vi "fast scanner v2.1.vi"() -> ()   [LabVIEW 2015]
uses:
  libs/Controls/outofrange.ctl
  libs/Controls/loopclock.ctl
  libs/Controls/fast scanner.ctl
  libs/Controls/String.ctl
  libs/Controls/Number.ctl
  <vilib>/Analysis/Matrix/Datatypes/RealMatrix.ctl
  <vilib>/userdefined/High Color/IMAQdx.ctl
  <vilib>/Analysis/6fits.llb/Curve Fitting Criteria.ctl
  <vilib>/Utility/miscctls.llb/LVFormatAndPrecisionTypeDef.ctl
  <vilib>/Utility/file.llb/Write Delimited Spreadsheet (string).vi
  <vilib>/Utility/file.llb/Read Delimited Spreadsheet (string).vi
  <vilib>/Utility/file.llb/Write Delimited Spreadsheet (I64).vi
  <vilib>/Utility/file.llb/Write Delimited Spreadsheet (DBL).vi
  Zaber A Series/Zaber A Series.lvlib
  libs/Proximity_sensor/MEDAQLib/MEDAQLib.lvlib
  <vilib>/Analysis/Matrix/NI_Matrix.lvlib
  <vilib>/Analysis/NI_AALPro.lvlib
panel:
  in  "Pause button 2":refnum<vi>
  in  "Acceleration\n [mm/s^2] 2":dbl=10.0 min=1.0 max=488.0 step=1.0
  in  "Speed Z [mm/s] 2":dbl(slide) caption="Z Speed\n[mm/s]" min=0.5 max=10.0 step=0.5 scale=0.5..10.0
  out "Measurement On!":bool
  out "Program Closed":bool
  out "Proximity on":bool
  out "Shutter Open":bool
  in  "Data folder path":path=path "D:/Users/XRF/Desktop/Dante_acquire6/Scan Data"
  out "DANTE loaded":bool
  out "IP added":bool
  out "Library Initialized":bool
  out "DANTE configured":bool
  out "Enum":T1=enum."MoveToStartPoint"
  out "scan mode":bool
  out "Port":refnum<visa-resource-name>
  out "MotorsReady":bool
  out "Speed 2":T2 scale=0.0..30.0
  in  "Tab Control":T3(tab)
  in  "Connect/Disconnect Prox":bool
  out "Proximity distance":dbl
  in  "Home":bool
  in  "StopMotion":bool
  in  "GoToZ":bool
  in  "GoToY":bool
  in  "GoToX":bool
  in  "GoTo Z [mm]":dbl format="%#.8g"
  in  "GoTo Y [mm]":dbl format="%#.8g"
  in  "GoTo X [mm]":dbl format="%#.8g"
  in  "Reduced Speed":bool
  in  "Speed Z [mm/s]":dbl(slide)=1.0 caption="Z Speed\n[mm/s]" min=0.5 max=10.0 step=0.5 scale=0.5..10.0
  in  "XY Speed\n[mm/s]":dbl(slide)=1.0 min=1.0 max=75.0 step=1.0 scale=1.0..75.0
  in  "Right":bool
  in  "Left":bool
  in  "Down":bool
  in  "Up":bool
  out "X [mm]":dbl format="%#.8g"
  out "Y [mm]":dbl format="%#.8g"
  out "Z [mm]":dbl format="%#.3g"
  out "Assignment":cluster{"Microstep Size":dbl, "Device":string}[](array[cluster])
  in  "Acceleration\n [mm/s^2]":dbl=10.0 min=1.0 max=488.0 step=1.0
  out "Error!":string
  in  "COM Port 2":string="COM5"
  in  "Sensor type 2":string="ild1420"
  in  "Closer":bool
  in  "Away":bool
  out "?":dbl[](graph)
  in  "Prox. distance lower limit":dbl=70.0
  in  "Prox. distance upper limit":dbl=70.0
  in  "limit":T4(radio)=enum."off Selection 4"
  in  "Connect/Disconnect Camera":bool
  in  "Session In":T5="cam0"
  out "stats out":T6
  in  "Tab Control 2":enum32{"ACQUISITION", "CALIBRATION", "ROI"}(tab)
  in  "Shutter Port":refnum<visa-resource-name>="COM4"
  in  "MEASUREMENT_Start":bool
  out "Elapsed Time":dbl caption="Elapsed Time [s]" format="%#_4g"
  in  "Preset Time [s]":dbl=1.0 min=0.2 step=0.1
  out "Progress":u32 caption="%" min=1 step=1
  in  "Close DANTE":bool
  in  "INIT DANTE":bool
  in  "IP Address":string="10.96.0.113"
  out "identifier out":string
  in  "Config. file path":path=path "D:/Users/XRF/Desktop/Dante_acquire6/Configuration files/DefaultParameters.xml"
  in  "Servo Channel":u8=9
  in  "Pause":bool
  in  "Stop acq":bool
  in  "Open Shutter":bool
  in  "SaveSpectrum":bool
  in  "CALIB_ClearPoints":bool
  in  "CALIB_AddPoint":bool
  in  "CALIB_Execute":bool
  in  "CalibArray":T7
  out "Slope":dbl=0.010046367851622875 caption="Slope (keV/channel)" format="%#.6f"
  out "Intercept":dbl=-0.03941267387944358 caption="Intercept (keV)" format="%#_6f"
  in  "ROI_Load":bool
  in  "ROI_Save":bool
  in  "ROI_RemoveAll":bool
  in  "ROI_Remove":bool
  out "ROI_Array":T10(array[cluster]) {"ROI begin channel" step=0.001; "ROI end channel" step=0.001; "Intensity" step=0.001; "Net Intensity" step=0.001; "Gauss Fit" step=0.001; "FWHM [keV]" step=0.001; "Center [keV]" step=0.001}
  in  "ROI_LowCh":u32=1800 caption="Lower Channel"
  in  "ROI_UpCh":u32=2000 caption="Upper Channel"
  in  "ROI_Cancel":bool
  in  "ROI_Set":bool
  in  "ROI_Add":bool
  in  "APPEARANCE_CursorVis":bool
  in  "APPEARANCE_Log/Lin":bool=TRUE
  out "SpectraPlot":dbl[](graph) caption="Waveform Graph"
  in  "APPEARANCE_E/CH":bool
  in  "Pause scan":bool
  out "LineProgress":dbl(slide) scale=0.0..10.0
  in  "Add acc dist [mm]":dbl=1.0 caption="Single line measurement time:" min=0.0 step=0.1
  in  "X velocity [mm/s]":dbl=50.0 min=0.0 step=0.1
  out "Total scan time [s]":dbl=1.0 min=0.0 step=0.1
  out "Total line time [s]":dbl=1.0 min=0.0 step=0.1
  out "Acq time [s]":dbl=1.0 min=0.0 step=0.1
  in  "AcqStartDelay":dbl caption="Acq start delay [ms]"
  in  "Abort scan":bool
  out "Acc time [s]":dbl=1.0 min=0.0 step=0.1
  out "Acc dist [mm]":dbl=1.0 caption="Single line measurement time:" min=0.0 step=0.1
  in  "X accel":dbl caption="X acceleration [mm/s^2]"
  out "Line #":i32=1 caption="/" min=0 step=1
  out "X scan velocity [mm/s]":dbl=1.0 min=0.0 step=0.1
  in  "QUICKSCAN_Start":bool
  out "Y error":T11
  out "X error":T11
  out "total # of points":i32=1 min=0 step=1
  out "Y steps":i32=1 min=1 step=1
  out "X steps":i32=1 min=1 step=1
  in  "step Y [mm]":dbl=1.0 min=0.0 step=0.1
  in  "Y end [mm]":dbl=1.0
  in  "Y start [mm]":dbl
  in  "step X [mm]":dbl=1.0 min=0.0 step=0.1
  in  "X end [mm]":dbl=1.0
  in  "X start [mm]":dbl
  in  "PresetVal":u32 caption="Time per pixel [ms]"
  out "X speed error":T11
  out "total line #":i32=1 caption="/" min=0 step=1
  out "Return movement time [s]":dbl=1.0 min=0.0 step=0.1
  out "2D graph 1":dbl[][](graph) caption="A"
  in  "MAP-1":u16(ring) items=["Rh-Ka", "Cu-Ka", "Ar-Ka", "All"]
  out "2D graph 2":dbl[][](graph) caption="A"
  in  "MAP-2":u16(ring) items=["Rh-Ka", "Cu-Ka", "Ar-Ka", "All"]
  out "2D graph 3":dbl[][](graph) caption="A"
  in  "MAP-3":u16(ring) items=["Rh-Ka", "Cu-Ka", "Ar-Ka", "All"]
  out "2D graph 4":dbl[][](graph) caption="A"
  in  "MAP-4":u16(ring) items=["Rh-Ka", "Cu-Ka", "Ar-Ka"]
  out "Sum spectra per line":u32[](graph)
  out "Spectra":u16[][](graph)
  out "scan timing [ms]":dbl[][](array[numeric])
  out "Y positions array":dbl[](array[numeric])
  out "2DSet":dbl[][][](array[numeric])
  out "size(s)":i32[](array[numeric])
  out "X-coordinates_map":dbl[][](array[numeric])
  out "Y-coordinates_map":dbl[][](array[numeric])
  out "Z-coordinates_map":dbl[][](array[numeric])
  out "X start position":dbl
  out "X end position":dbl
  out "Y start position":dbl
  out "Y end position":dbl
  out "DPP Configuration":T12={"reset_recovery_time"=300, "edge_peaking_time"=5, "flat_top"=5, "peaking_time"=25, "gain"=1.0, "max_risetime"=35.0, "fast_filter_thr"=100, "zero_peak_freq"=5.0, "inverted_input"=0, "base_offset"=0, "reset_threshold"=1000, "overflow_recovery"=0, "tail_coefficient"=0.0, "energy_filter_thr"=25, "energy_baseline_thr"=25, "max_peaking_time"=0, "edge_flat_top"=1, "time_constant"=0.0, "baseline_samples"=64, "other_param"=0}
  out "ZaberError":errorcluster
  out "Loop Speed [1/s]":dbl caption="Elapsed Time [s]" format="%#_2f"
  # "ROI  Name       Begin           End         Intensity    Net intnsity   Gauss Fit      FWHM         Center\n                         channel      channel                                                              [keV]            [keV]"
  # "waiting \ntill stage \nreaches \nproper speed"
  # "sending \nmovement \ncommand"
  # "waiting till \nstage stops \n(breaking)"
  # "aquisition"
types:
  T1 = typedef "fast scanner.ctl" = enum16{"Initialisation", "IDLE", "Acquire", "SaveSpectra", "PrepareMap", "MoveToStartPoint", "AcquireLine", "Close"}
  T2 = typedef "loopclock.ctl" = dbl
  T3 = enum32{"Stage Control", "Spectrum", "Fast Scan Definition", "Map Data", "Map Data 2", "Map Data 3", "Map Data 4", "Line Data", "scan info", "scan info 2", "DPP Config"}
  T4 = enum32{"lower", "lower/upper", "off Selection 4"}
  T5 = typedef "IMAQdx.ctl" = refnum<k21>
  T6 = cluster{u64, u64, dbl, dbl, u32, u32, u32, u32, u32, u32, u32, u32, u32, u32, u32}
  T7 = typedef "NI_Matrix.lvlib/RealMatrix.ctl" = dbl[][]
  T8 = typedef "String.ctl" = string
  T9 = typedef "Number.ctl" = dbl
  T10 = cluster{"ROI name":T8, "ROI begin channel":T9, "ROI end channel":T9, "Intensity":T9, "Net Intensity":T9, "Gauss Fit":T9, "FWHM [keV]":T9, "Center [keV]":T9}[]
  T11 = typedef "outofrange.ctl" = bool
  T12 = cluster{"reset_recovery_time":u32, "edge_peaking_time":u32, "flat_top":u32, "peaking_time":u32, "gain":dbl, "max_risetime":dbl, "fast_filter_thr":u32, "zero_peak_freq":dbl, "inverted_input":u8, "base_offset":u32, "reset_threshold":u32, "overflow_recovery":u32, "tail_coefficient":dbl, "energy_filter_thr":u32, "energy_baseline_thr":u32, "max_peaking_time":u32, "edge_flat_top":u32, "time_constant":dbl, "baseline_samples":u32, "other_param":u32}
  T13 = cluster{"X min":dbl, "X max":dbl, "Y min":dbl, "Y max":dbl, "Z min":dbl, "Z max":dbl}
  T14 = enum32{"Size Tabs To Contents", "Size All Tabs to Largest Tab", "Fixed Tab Size"}
  T15 = enum8{"Enabled", "Disabled", "Disabled and Grayed Out"}
  T16 = cluster{"ROI name":string, "ROI begin channel":i64, "ROI end channel":i64, "Intensity":i64, "Net Intensity":i64, "Gauss Fit":dbl, "FWHM [keV]":dbl, "Center [keV]":dbl}
  T17 = typedef "LVFormatAndPrecisionTypeDef.ctl" = cluster{"Format":u8, "Precision":u8}
  T18 = cluster{"X abs start":dbl, "X abs end":dbl, "Y abs start":dbl, "Y abs end":dbl, "Z abs start":dbl, "Z abs end":dbl, "X step":dbl, "Y step":dbl, "Z step":dbl}
  T19 = typedef "ConfigurationDPP.ctl" = cluster{"reset_recovery_time":u32, "edge_peaking_time":u32, "flat_top":u32, "peaking_time":u32, "gain":dbl, "max_risetime":dbl, "fast_filter_thr":u32, "zero_peak_freq":dbl, "inverted_input":u8, "base_offset":u32, "reset_threshold":u32, "overflow_recovery":u32, "tail_coefficient":dbl, "energy_filter_thr":u32, "energy_baseline_thr":u32, "max_peaking_time":u32, "edge_flat_top":u32, "time_constant":dbl, "baseline_samples":u32, "other_param":u32}
  T20 = cluster{"ROI name":string, "ROI begin channel":i64, "ROI end channel":i64, "Intensity":i64, "Net Intensity":i64, "Gauss Fit":dbl, "FWHM [keV]":dbl, "Center [keV]":dbl}[]
  T21 = typedef "NI_AALPro.lvlib/Curve Fitting Criteria.ctl" = u16
  T22 = typedef "LVMinMaxIncTypeDef.ctl" = cluster{"Minimum":dbl, "Maximum":dbl, "Increment":dbl}
  T23 = typedef "LVRangeTypeDef.ctl" = cluster{"Minimum":dbl, "Maximum":dbl, "Increment":dbl, "Minor Increment":dbl, "Start":dbl}
  T24 = cluster{"scaledData[0]":dbl, "scaledData[1]":dbl, "scaledData[2]":dbl, "scaledData[3]":dbl, "scaledData[4]":dbl, "scaledData[5]":dbl, "scaledData[6]":dbl, "scaledData[7]":dbl, "scaledData[8]":dbl}
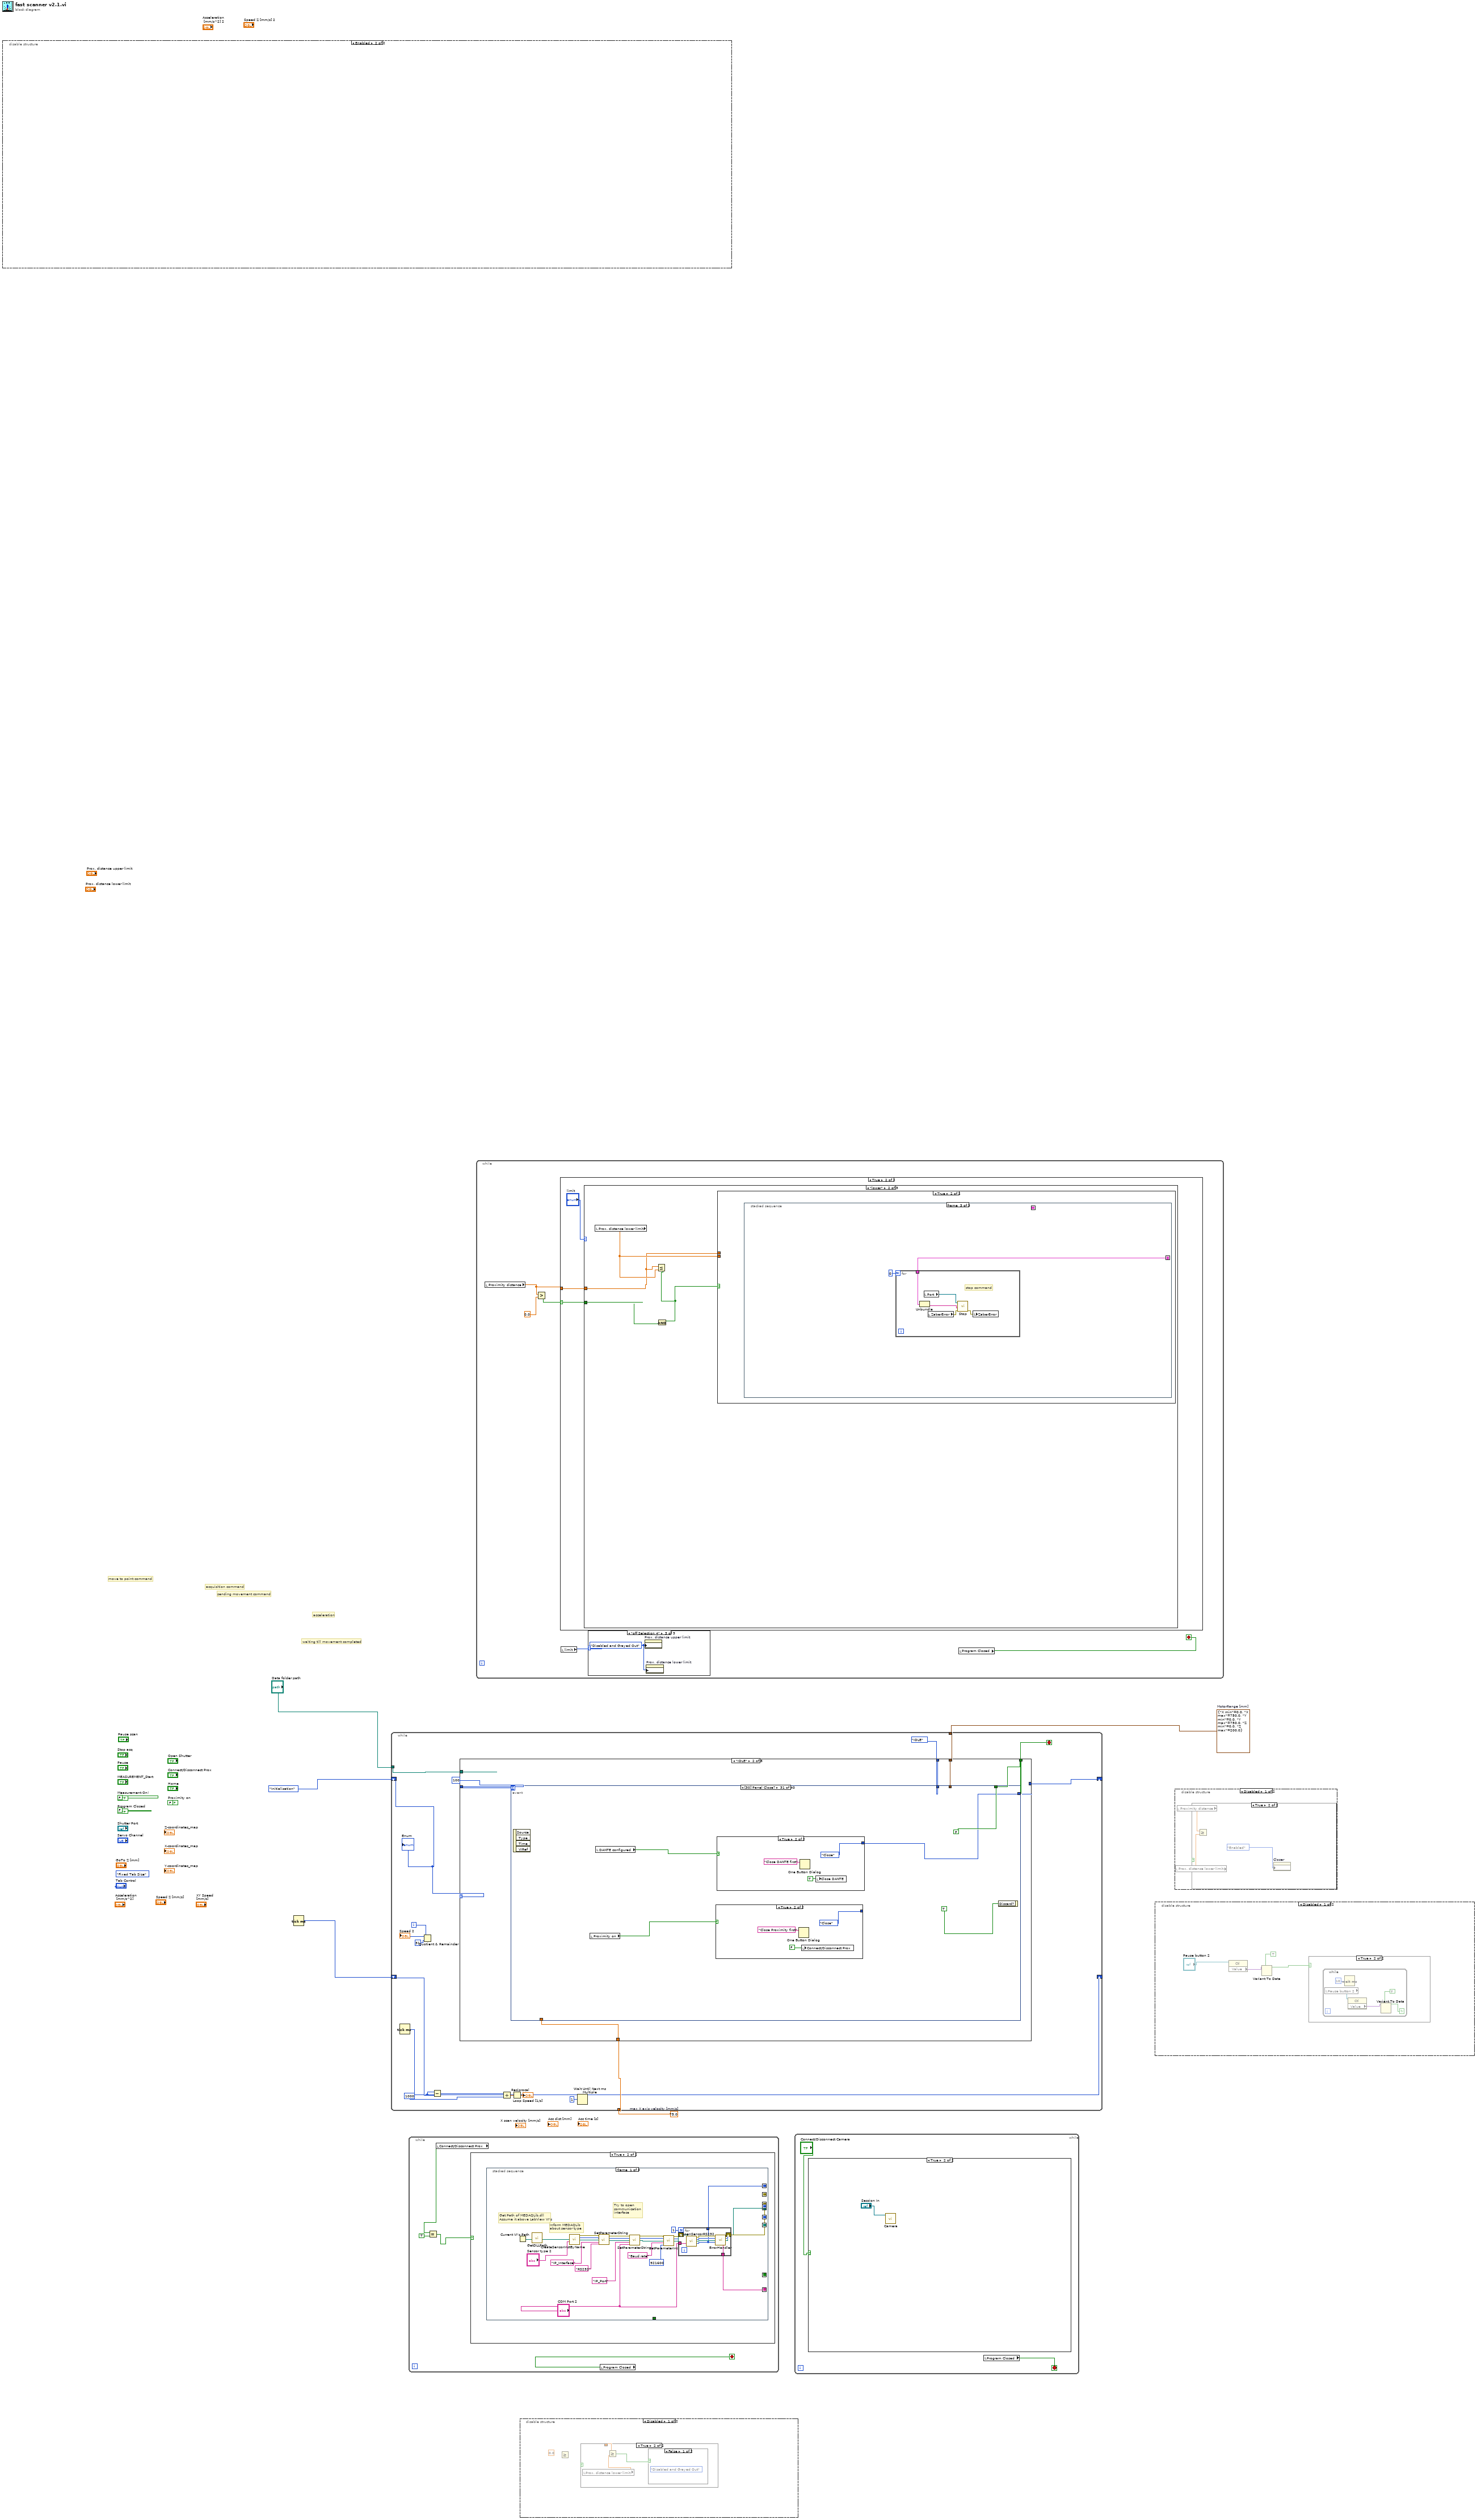
[diagram p0: block diagram]
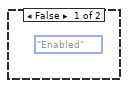
[diagram p2: hidden frame]
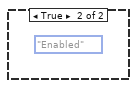
[diagram p3: hidden frame]
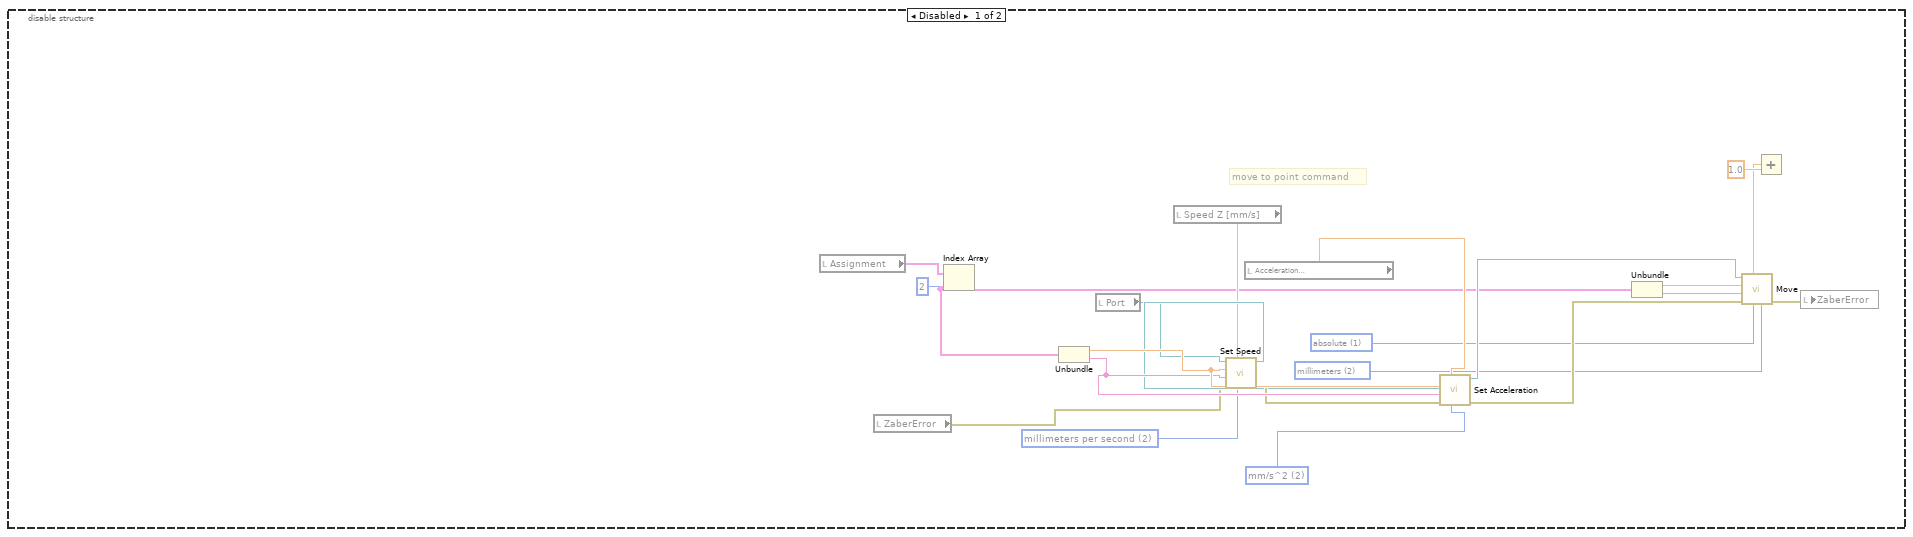
[diagram p10: hidden frame]
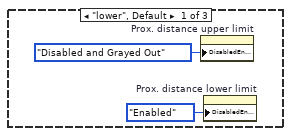
[diagram p11: hidden frame]
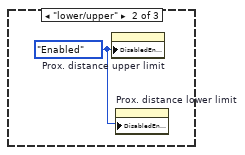
[diagram p12: hidden frame]
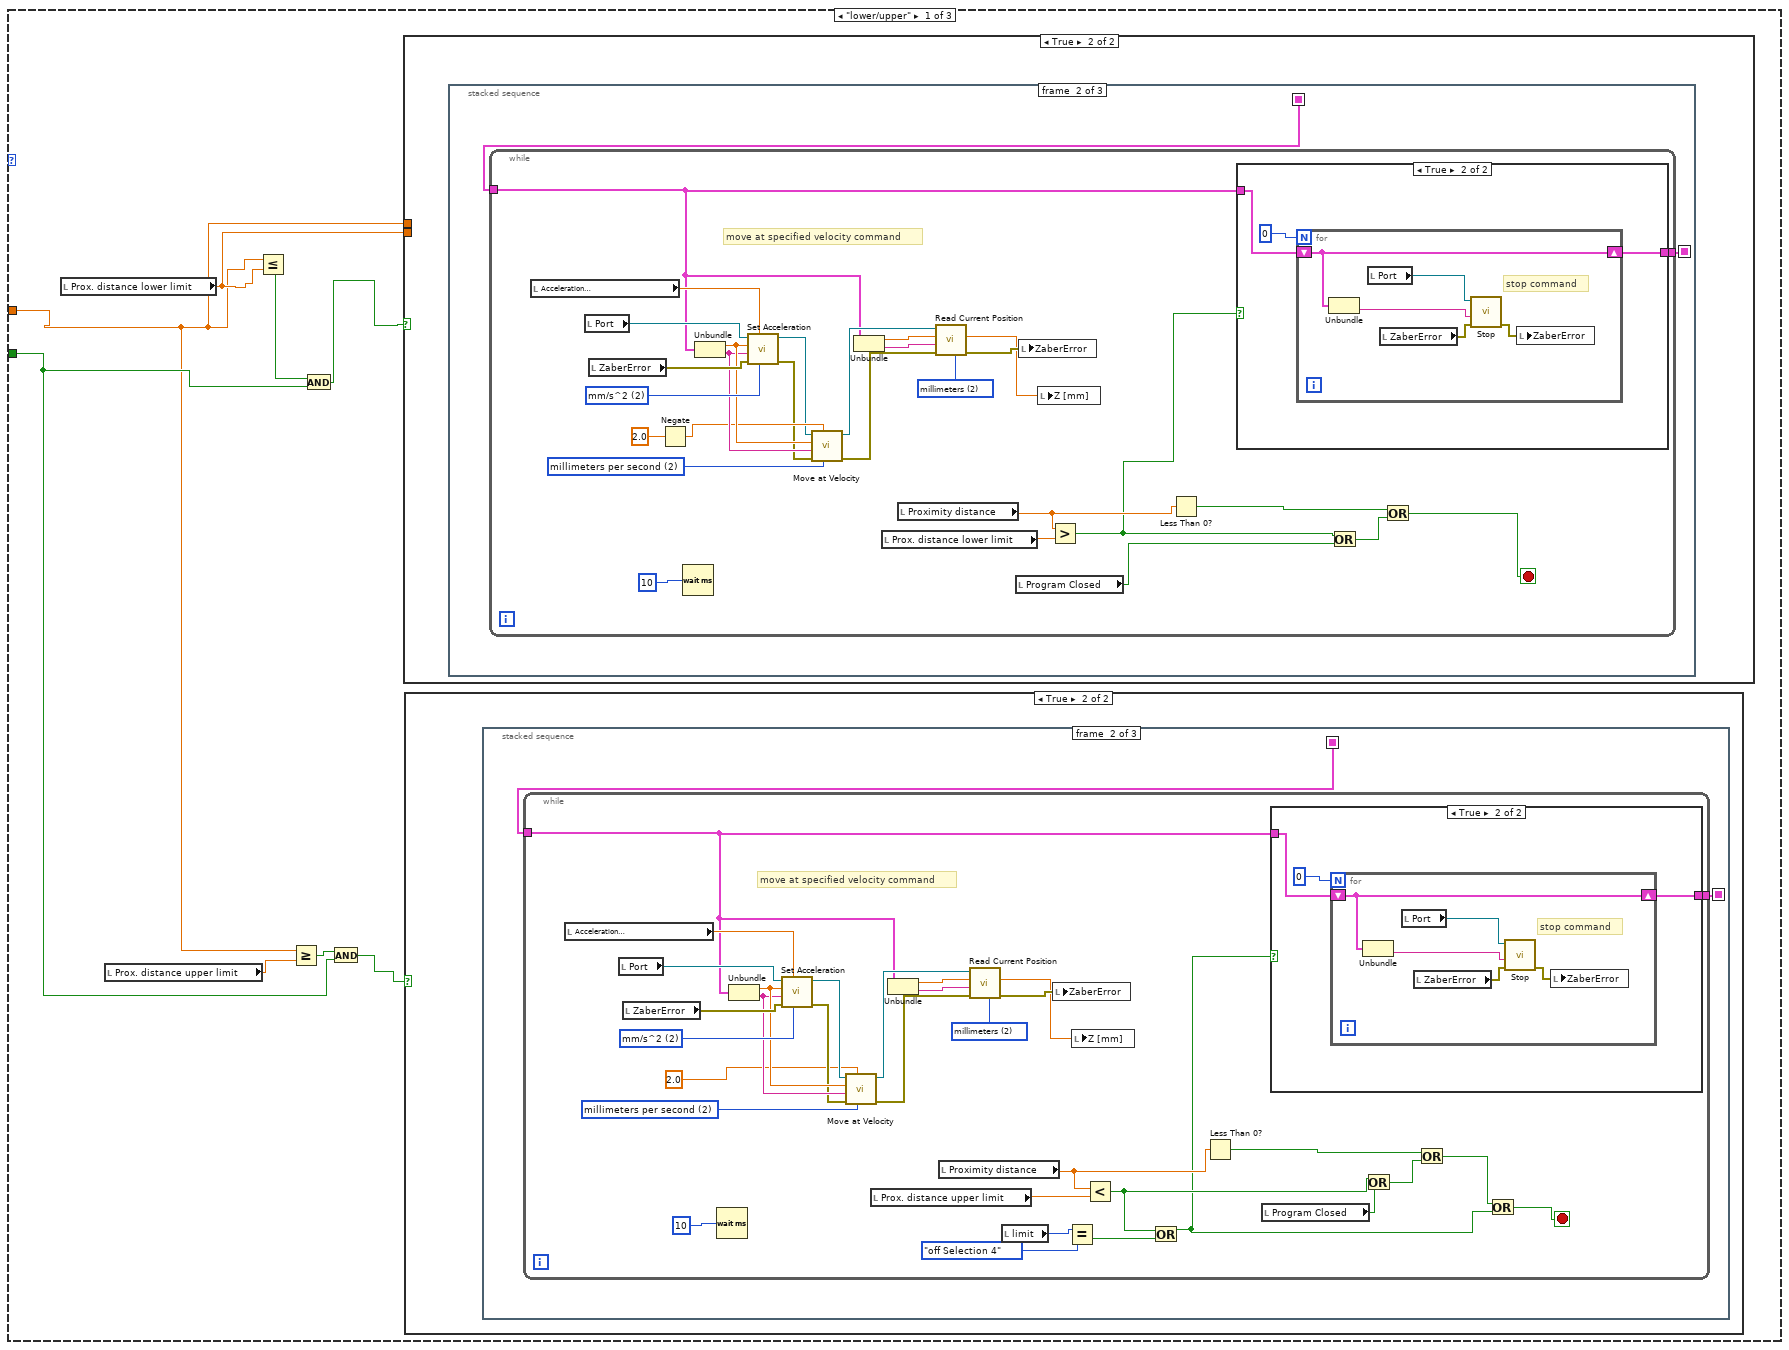
[diagram p14: hidden frame]
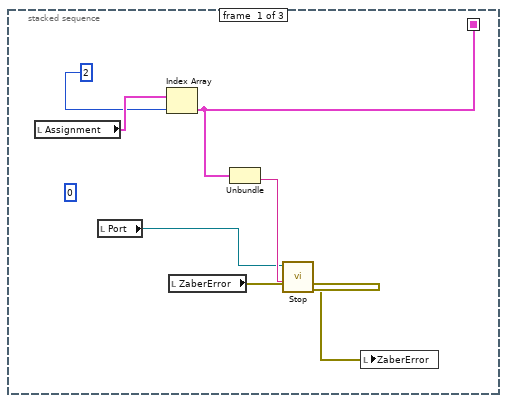
[diagram p16: hidden frame]
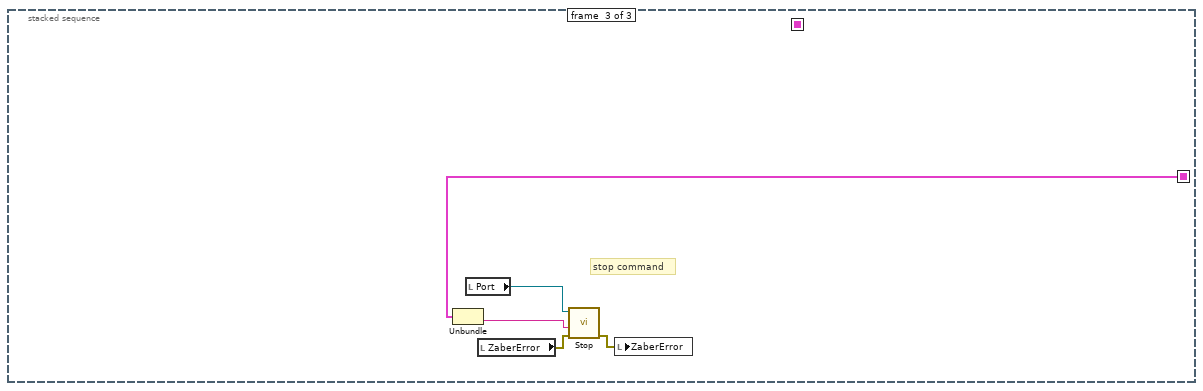
[diagram p18: hidden frame]
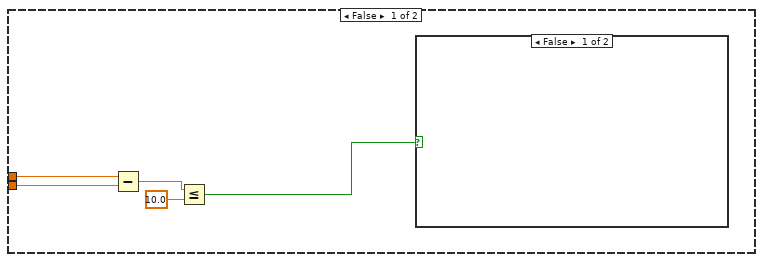
[diagram p19: hidden frame]
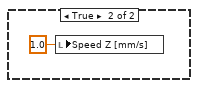
[diagram p20: hidden frame]
diagram:
  w5 = 75.0  # max X axis velocity [mm/s]
  w7 = T13 {"X min"=0.0, "X max"=750.0, "Y min"=0.0, "Y max"=750.0, "Z min"=0.0, "Z max"=200.0}  # MotorRange [mm]
  (unwired) T14."Fixed Tab Size" ("Tab Size")
  # "waiting till movement completed"
  # "sending movement command"
  # "acquisition command"
  # "move to point command"
  # "acceleration"
  n1 = disable-structure shown="Enabled" {
    frame Disabled {
      w23 = u16 2 items=["device units", "microns/s^2", "mm/s^2", "inches/s^2", "degrees/s^2"] ("Units (0: data)")
      w21 = u16 2 items=["device speed units", "microns per second", "millimeters per second", "inches per second", "degrees per second"] ("Units (0: device speed units)")
      w14 = u16 2 items=["microsteps", "microns", "millimeters", "inches", "degrees"] ("Units (0: microsteps)")
      w12 = u16 1 items=["relative", "absolute"] ("Movement Type (0: relative)")
      # "move to point command"
      n2 = local read "Assignment"() -> (w15:cluster{"Microstep Size":dbl, "Device":string}[])
      n3 = local read "ZaberError"() -> (w22:errorcluster)
      n4 = Index Array(array=w15, index=2) -> (element=w16:cluster{"Microstep Size":dbl, "Device":string})
      n5 = Unbundle(w16) -> ("Microstep Size"=w29:dbl, "Device"=w28:string)
      n6 = local read "Port"() -> (w19:refnum<visa-resource-name>)
      n7 = local read "Speed Z [mm/s]"() -> (w20:dbl)
      n8 = call "Set Speed.vi"("Units (0: data)"=w21, "New Speed"=w20, "error in (no error)"=w22, "Device and Axis"=w28, "Microstep Size (0)"=w29, "VISA resource name"=w19) -> ("error out"=w26:errorcluster, "VISA resource name out"=w24:refnum<visa-resource-name>)  [unwired: 4 in]
      n9 = local read "Acceleration\n [mm/s^2]"() -> (w30:dbl)
      n10 = call "Set Acceleration.vi"("Units (0: data)"=w23, "New Acceleration"=w30, "error in (no error)"=w26, "Device and Axis"=w28, "Microstep Size (0)"=w29, "VISA resource name"=w24) -> ("error out"=w27:errorcluster, "VISA resource name out"=w25:refnum<visa-resource-name>)  [unwired: 4 in]
      n11 = Unbundle(w16) -> ("Microstep Size"=w17:dbl, "Device"=w18:string)
      n12 = Add(y=1.0) -> (x+y=w9:dbl)  [unwired: 1 in]
      n13 = call "Move.vi"("Units (0: microsteps)"=w14, "Movement Type (0: relative)"=w12, "Move Distance (0)"=w9, "error in (no error)"=w27, "Device and Axis"=w18, "Microstep Size (0)"=w17, "VISA resource name"=w25) -> ("error out"=w13:errorcluster)  [unwired: 3 in, 1 out]
      n14 = local write "ZaberError"(w13) -> ()
    }
    frame Enabled {
    }
  }
  n15 = Tick Count (ms)() -> (millisecond timer value=w8:u32)
  n16 = while {
    shift-right: [w32] -> _
    shift-left: fast_scanner."Initialisation" ("Enum") -> [w36]
    shift-right: [w31] -> _
    shift-left: w8 -> [w48]
    tunnel: w7 -> [w37]
    tunnel: w5 -> [w35]
    tunnel: "Data folder path" -> [w34]
    i -> [w44]
    stop <- w33 stop-if-true
    n17 = Tick Count (ms)() -> (millisecond timer value=w31:u32)
    n18 = Quotient & Remainder(x=w44, y=31) -> (x-y*floor(x/y)=→"Speed 2":i32)  [unwired: 1 out]
    n19 = Subtract(x=w31, y=w48) -> (x-y=w46:u32)
    n20 = case shown="\"IDLE\"" w36 {
      tunnel: 100 ("LoopTimer [ms]") -> [_ w99 _ _ _ _ _ _]
      tunnel: [w50 w101 fast_scanner."IDLE" ("Enum") w1044 w1054 fast_scanner."AcquireLine" ("Enum") w1178 fast_scanner."Close" ("Enum")] -> w32
      tunnel: [FALSE ("VI stop") w100 FALSE ("VI stop") FALSE ("VI stop") FALSE ("VI stop") FALSE ("VI stop") FALSE ("VI stop") TRUE ("VI stop")] -> w33
      tunnel: fast_scanner."IDLE" ("Enum") -> [w50 w97 _ w1044 w1054 _ w1178 _]
      tunnel: w37 -> [_ w98 _ _ _ _ _ _]
      tunnel: w35 -> [_ w96 _ _ _ _ _ _]
      tunnel: w34 -> [_ _ _ _ _ _ w1177 _]
      frame "Initialisation", Default {
        n21 = stacked-sequence {
          frame #0 {
            w51 = FALSE ("DANTE loaded")
            w52 = T15."Disabled and Grayed Out" ("Disabled")
            w53 = FALSE ("batch mode")
            n22 = local write "scan mode"(w53) -> ()
            n23 = local write "QUICKSCAN_Start"(w53) -> ()
            n24 = local write "DANTE loaded"(w51) -> ()
            n25 = local write "Library Initialized"(w51) -> ()
            n26 = local write "IP added"(w51) -> ()
            n27 = control-ref of="This VI"() -> (w54:refnum<vi>)
            n28 = property class="VI"(reference=w54, "Edit Mode"=TRUE ("Edit Mode On Open")) -> ()  [unwired: 1 in, 2 out]
            n29 = property on="total line #" class="DigNum (strict)"("DisabledEnum"=w52) -> ()  [unwired: 2 in, 2 out]
            n30 = property on="Line #" class="DigNum (strict)"("DisabledEnum"=w52) -> ()  [unwired: 2 in, 2 out]
          }
          frame #1 {
            n31 = property on="Closer" class="Bool (strict)"("DisabledEnum"=T15."Enabled" ("Disabled")) -> ()  [unwired: 2 in, 2 out]
            n32 = property on="APPEARANCE_CursorVis" class="Bool (strict)"() -> ("Value"=w57:bool)  [unwired: 2 in, 2 out]
            n33 = property on="APPEARANCE_Log/Lin" class="Bool (strict)"() -> ("Value"=w58:bool)  [unwired: 2 in, 2 out]
            n34 = property on="APPEARANCE_CursorVis" class="Bool (strict)"("Val(Sgnl)"=w57) -> ()  [unwired: 2 in, 2 out]
            n35 = property on="APPEARANCE_Log/Lin" class="Bool (strict)"("Val(Sgnl)"=w58) -> ()  [unwired: 2 in, 2 out]
          }
          frame #2 {
            w68 = 1.0 ("New Speed")
            w69 = 10.0 ("New Speed")
            w72 = u16 2 items=["device units", "microns/s", "mm/s", "inches/s", "degrees/s"] ("Units (0: data)")
            # "setting default speed"
            n36 = call "Zaber_Init.vi"() -> ("Assignment"=w73:cluster{"Microstep Size":dbl, "Device":string}[], "Axes Ass"=→"MotorsReady":bool, "VISA resource name out"=w81:refnum<visa-resource-name>)
            "Assignment" <- w73
            n37 = Index Array(array=w73, index=2) -> (element=w60:cluster{"Microstep Size":dbl, "Device":string})
            n38 = Index Array(array=w73, index=1) -> (element=w62:cluster{"Microstep Size":dbl, "Device":string})
            n39 = Index Array(array=w73, index=0) -> (element=w67:cluster{"Microstep Size":dbl, "Device":string})
            n40 = local read "ZaberError"() -> (w82:errorcluster)
            n41 = Unbundle(w67) -> ("Microstep Size"=w66:dbl, "Device"=w65:string)
            n42 = call "Set Speed.vi"("Units (0: data)"=w72, "New Speed"=w69, "error in (no error)"=w82, "Device and Axis"=w65, "Microstep Size (0)"=w66, "VISA resource name"=w81) -> ("error out"=w78:errorcluster, "VISA resource name out"=w77:refnum<visa-resource-name>)  [unwired: 4 in]
            n43 = Unbundle(w62) -> ("Microstep Size"=w63:dbl, "Device"=w64:string)
            n44 = call "Set Speed.vi"("Units (0: data)"=w72, "New Speed"=w69, "error in (no error)"=w78, "Device and Axis"=w64, "Microstep Size (0)"=w63, "VISA resource name"=w77) -> ("error out"=w75:errorcluster, "VISA resource name out"=w76:refnum<visa-resource-name>)  [unwired: 4 in]
            n45 = local write "XY Speed\n[mm/s]"(w69) -> ()
            n46 = Unbundle(w60) -> ("Microstep Size"=w61:dbl, "Device"=w59:string)
            n47 = call "Set Speed.vi"("Units (0: data)"=w72, "New Speed"=w68, "error in (no error)"=w75, "Device and Axis"=w59, "Microstep Size (0)"=w61, "VISA resource name"=w76) -> ("error out"=w71:errorcluster, "VISA resource name out"=→"Port":refnum<visa-resource-name>)  [unwired: 4 in]
            n48 = local write "Speed Z [mm/s]"(w68) -> ()
            n49 = local write "ZaberError"(w71) -> ()
          }
          frame #3 {
            w87 = FALSE ("Boolean")
            n50 = local read "Shutter Port"() -> (w89:refnum<visa-resource-name>)
            n51 = local read "Servo Channel"() -> (w88:u8)
            n52 = control-ref of="Open Shutter"() -> (w84:refnum<vi>)
            n53 = local write "Open Shutter"(FALSE ("Open Shutter")) -> ()
            n54 = call "LINX_servo.vi"("Servo Channel"=w88, "Serial Port"=w89, "Boolean"=w87) -> ("Shatter Open"=w86:bool)  [unwired: 8 in]
            n55 = property on="Property Node" class="Bool (strict)"(reference=w84, "Value"=w87) -> ()  [unwired: 1 in, 2 out]
            n56 = local write "Shutter Open"(w86) -> ()
          }
          frame #4 {
            # "Close communication interface\nRelease MEDAQLib's internal structures"
            n57 = call "ReleaseSensorInstance.vi"() -> ("Fehler (Ausgang)"=w90:errorcluster, "instanceHandle"=w91:u32, "DLL-Path"=w92:path)  [unwired: 3 in, 10 out]
            n58 = call "CloseSensor.vi"("Fehler (Eingang, kein Fehler)"=w90, "instanceHandle"=w91, "DLL-Path"=w92) -> ()  [unwired: 13 out]
          }
          frame #5 {
            n59 = call "DANTE close.vi"() -> ("error out"=w93:errorcluster, "identifier out"=w94:string)  [unwired: 9 in, 1 out]
            n60 = local write "identifier out"(w94) -> ()
            n61 = case shown="No Error" w93 {
              frame No Error {
                w95 = FALSE ("DANTE loaded")
                n62 = local write "DANTE loaded"(w95) -> ()
                n63 = local write "Library Initialized"(w95) -> ()
                n64 = local write "IP added"(w95) -> ()
                n65 = local write "DANTE configured"(w95) -> ()
              }
              frame Error {
              }
            }
          }
        }
      }
      frame "IDLE" {
        n66 = event shown="[30] Panel Close?" {
          selector: _ -> [_ _ _ _ _ _ _ _ _ _ _ _ _ _ _ _ _ _ _ _ _ _ _ _ _ _ _ _ _ _ _ _ _ _ _ _ _ _ _ _]
          dyn-events: _ -> [_ _ _ _ _ _ _ _ _ _ _ _ _ _ _ _ _ _ _ _ _ _ _ _ _ _ _ _ _ _ _ _ _ _ _ _ _ _ _ _]
          timeout: w99 -> [_ _ _ _ _ _ _ _ _ _ _ _ _ _ _ _ _ _ _ _ _ _ _ _ _ _ _ _ _ _ _ _ _ _ _ _ _ _ _ _]
          tunnel: [FALSE ("VI stop") _ _ _ FALSE ("VI stop") FALSE ("VI stop") FALSE ("VI stop") FALSE ("VI stop") FALSE ("VI stop") FALSE ("VI stop") FALSE ("VI stop") FALSE ("VI stop") FALSE ("VI stop") FALSE ("VI stop") FALSE ("VI stop") FALSE ("VI stop") FALSE ("VI stop") FALSE ("VI stop") FALSE ("VI stop") FALSE ("VI stop") FALSE ("VI stop") FALSE ("VI stop") FALSE ("VI stop") FALSE ("VI stop") FALSE ("VI stop") w706 FALSE ("VI stop") FALSE ("VI stop") FALSE ("VI stop") FALSE ("VI stop") FALSE ("VI stop") FALSE ("VI stop") _ FALSE ("VI stop") FALSE ("VI stop") FALSE ("VI stop") FALSE ("VI stop") FALSE ("VI stop") FALSE ("VI stop") _] -> w100
          tunnel: [w102 w138 w143 _ w153 w157 w162 w169 w269 w285 w300 w318 w349 w352 w361 w441 w462 w465 w485 w539 w562 w585 w649 w662 w673 w705 w766 w802 w837 w881 w899 fast_scanner."Acquire" ("Enum") fast_scanner."SaveSpectra" ("Enum") w922 w926 w935 w973 w982 w992 w997] -> w101
          tunnel: w97 -> [_ w138 w143 _ w153 w157 w162 w169 w269 w285 w300 w318 w349 w352 w361 w441 w462 _ w485 w539 w562 w585 w649 w662 w673 w705 w766 w802 w837 w881 _ _ _ w922 w926 w935 w973 w982 w992 w997]
          tunnel: w98 -> [_ _ _ _ _ _ _ _ _ _ _ _ _ _ _ w429 w448 _ _ _ _ _ _ _ _ _ _ _ _ _ _ _ _ _ _ _ _ _ _ _]
          tunnel: w96 -> [_ _ _ _ _ _ _ _ _ _ _ _ _ _ _ w418 _ _ _ _ _ _ _ _ _ _ _ _ _ _ _ _ _ _ _ _ _ _ _ _]
          event Timeout {
            n67 = event-data() -> ()  [unwired: 1 in, 1 out]
            n68 = stacked-sequence {
              tunnel: [_ w135] -> w102
              frame #0 {
                w114 = u16 2 items=["microsteps", "microns", "millimeters", "inches"] ("Units (0: microsteps)")
                # "reading manipulator position"
                n69 = local read "Assignment"() -> (w113:cluster{"Microstep Size":dbl, "Device":string}[])
                n70 = local read "ZaberError"() -> (w126:errorcluster)
                n71 = local read "Port"() -> (w127:refnum<visa-resource-name>)
                n72 = Index Array(array=w113, index=0) -> (element=w112:cluster{"Microstep Size":dbl, "Device":string})
                n73 = Index Array(array=w113, index=1) -> (element=w108:cluster{"Microstep Size":dbl, "Device":string})
                n74 = Index Array(array=w113, index=2) -> (element=w104:cluster{"Microstep Size":dbl, "Device":string})
                n75 = Unbundle(w112) -> ("Microstep Size"=w111:dbl, "Device"=w110:string)
                n76 = call "Read Current Position.vi"("Units (0: microsteps)"=w114, "error in (no error)"=w126, "Device and Axis"=w110, "Microstep Size (0)"=w111, "VISA resource name"=w127) -> ("error out"=w125:errorcluster, "Position"=→"X [mm]":dbl, "VISA resource name out"=w124:refnum<visa-resource-name>)  [unwired: 4 in]
                n77 = Unbundle(w108) -> ("Microstep Size"=w109:dbl, "Device"=w107:string)
                n78 = call "Read Current Position.vi"("Units (0: microsteps)"=w114, "error in (no error)"=w125, "Device and Axis"=w107, "Microstep Size (0)"=w109, "VISA resource name"=w124) -> ("error out"=w123:errorcluster, "Position"=→"Y [mm]":dbl, "VISA resource name out"=w122:refnum<visa-resource-name>)  [unwired: 4 in]
                n79 = Unbundle(w104) -> ("Microstep Size"=w106:dbl, "Device"=w105:string)
                n80 = call "Read Current Position.vi"("Units (0: microsteps)"=w114, "error in (no error)"=w123, "Device and Axis"=w105, "Microstep Size (0)"=w106, "VISA resource name"=w122) -> ("error out"=w121:errorcluster, "Position"=→"Z [mm]":dbl)  [unwired: 4 in, 1 out]
                n81 = local write "ZaberError"(w121) -> ()
              }
              frame #1 {
                n82 = local read "scan mode"() -> (w128:bool)
                n83 = Select(t=T15."Disabled" ("Disabled"), s=w128, f=T15."Enabled" ("Disabled")) -> (s? t:f=w132:T15)
                n84 = case shown="False" w128 {
                  tunnel: [T15."Disabled and Grayed Out" ("Disabled") T15."Enabled" ("Disabled")] -> w129
                  frame False {
                  }
                  frame True {
                  }
                }
                n85 = property on="QUICKSCAN_Start" class="Bool (strict)"("DisabledEnum"=w132) -> ()  [unwired: 2 in, 2 out]
                n86 = property on="total line #" class="DigNum (strict)"("DisabledEnum"=w129) -> ()  [unwired: 2 in, 2 out]
                n87 = property on="Line #" class="DigNum (strict)"("DisabledEnum"=w129) -> ()  [unwired: 2 in, 2 out]
                n88 = Select(t=fast_scanner."MoveToStartPoint" ("Enum"), s=w128, f=fast_scanner."IDLE" ("Enum")) -> (s? t:f=w135:T1)
              }
            }
          }
          event "Open Shutter": Value Change {
            n89 = event-data() -> ()  [unwired: 1 in, 6 out]
            n90 = local read "Shutter Port"() -> (w141:refnum<visa-resource-name>)
            n91 = local read "Open Shutter"() -> (w142:bool)
            n92 = local read "Servo Channel"() -> (w140:u8)
            n93 = call "LINX_servo.vi"("Servo Channel"=w140, "Serial Port"=w141, "Boolean"=w142) -> ("Shatter Open"=→"Shutter Open":bool)  [unwired: 8 in]
          }
          event "Connect/Disconnect Prox": Value Change {
            n94 = event-data() -> ()  [unwired: 1 in, 6 out]
          }
          event "Connect/Disconnect Camera": Value Change {
            n95 = event-data() -> ()  [unwired: 1 in, 6 out]
          }
          event "INIT DANTE": Value Change {
            n96 = event-data() -> ()  [unwired: 1 in, 6 out]
            n97 = call "Load_XML2.vi"("XML File Path 2"="Config. file path") -> ("DPP Configuration"=w144:T19)  [unwired: 10 in]
            "DPP Configuration" <- w144
            n98 = call "DANTE init & config 2.vi"("DPP Configuration"=w144, "IP Address"="IP Address") -> ("DANTE configured"=→"DANTE configured":bool, "DANTE loaded"=→"DANTE loaded":bool, "IP added"=→"IP added":bool, "Library Initialized"=→"Library Initialized":bool, "identifier out"=→"identifier out":string)  [unwired: 5 in]
          }
          event "Close DANTE": Value Change {
            n99 = event-data() -> ()  [unwired: 1 in, 6 out]
            n100 = call "DANTE close.vi"() -> ("error out"=w154:errorcluster, "identifier out"=w155:string)  [unwired: 9 in, 1 out]
            n101 = local write "identifier out"(w155) -> ()
            n102 = case shown="No Error" w154 {
              frame No Error {
                w158 = FALSE ("DANTE loaded")
                n103 = local write "DANTE loaded"(w158) -> ()
                n104 = local write "Library Initialized"(w158) -> ()
                n105 = local write "IP added"(w158) -> ()
                n106 = local write "DANTE configured"(w158) -> ()
              }
              frame Error {
              }
            }
          }
          event "Abort scan": Value Change {
            n107 = event-data() -> ()  [unwired: 1 in, 6 out]
            n108 = local read "Shutter Open"() -> (w159:bool)
            n109 = case shown="True" w159 {
              frame False {
              }
              frame True {
                w166 = FALSE ("Boolean")
                n110 = local read "Shutter Port"() -> (w168:refnum<visa-resource-name>)
                n111 = local read "Servo Channel"() -> (w167:u8)
                n112 = control-ref of="Open Shutter"() -> (w164:refnum<vi>)
                n113 = call "LINX_servo.vi"("Servo Channel"=w167, "Serial Port"=w168, "Boolean"=w166) -> ("Shatter Open"=w165:bool)  [unwired: 8 in]
                n114 = local write "Shutter Open"(w165) -> ()
                n115 = property on="Property Node" class="Bool (strict)"(reference=w164, "Value"=w166) -> ()  [unwired: 1 in, 2 out]
              }
            }
            n116 = local write "scan mode"(FALSE ("scan mode")) -> ()
            n117 = local write "QUICKSCAN_Start"(FALSE ("QUICKSCAN_Start")) -> ()
          }
          event "ROI_Add": Value Change {
            n118 = event-data() -> ()  [unwired: 1 in, 6 out]
            n119 = stacked-sequence {
              seq-local: [_ w180 _ _ _] -> [_ _ w231 _ _]
              seq-local: [_ w179 _ _ _] -> [_ _ w230 _ _]
              frame #0 {
                w175 = TRUE ("Cursor.Visible")
                w177 = T15."Enabled" ("Disabled")
                n120 = control-ref of="SpectraPlot"() -> (w172:refnum<vi>)
                n121 = control-ref of="ROI_Add"() -> (w171:refnum<vi>)
                n122 = property class="WFGraph (strict)"(reference=w172, "Active Cursor"=u32 0, "Cursor.Visible"=w175, "Active Cursor"=u32 1, "Cursor.Visible"=w175) -> ()  [unwired: 1 in, 2 out]
                n123 = property on="Property Node" class="Bool"(reference=w171, "DisabledEnum"=T15."Disabled and Grayed Out" ("Disabled")) -> ()  [unwired: 1 in, 2 out]
                n124 = property on="ROI_Set" class="Bool (strict)"("DisabledEnum"=w177) -> ()  [unwired: 2 in, 2 out]
                n125 = property on="ROI_Cancel" class="Bool (strict)"("DisabledEnum"=w177) -> ()  [unwired: 2 in, 2 out]
                n126 = property on="SpectraPlot" class="WFGraph (strict)"() -> ("Value"=w176:dbl[])  [unwired: 2 in, 2 out]
                n127 = property on="SpectraPlot" class="WFGraph (strict)"("Val(Sgnl)"=w176) -> ()  [unwired: 2 in, 2 out]
              }
              frame #1 {
                n128 = while {
                  tunnel: [w183] -> w180
                  tunnel: [w181] -> w179
                  stop <- w182 stop-if-true
                  n129 = event shown="[4] \"ROI_Set\": Mouse Up" {
                    selector: _ -> [_ _ _ _ _]
                    dyn-events: _ -> [_ _ _ _ _]
                    timeout: 10 -> [_ _ _ _ _]
                    tunnel: [TRUE TRUE TRUE FALSE TRUE] -> w183
                    tunnel: [FALSE FALSE FALSE TRUE TRUE] -> w182
                    tunnel: [_ _ _ _ w227] -> w181
                    event Timeout {
                      n130 = event-data() -> ()  [unwired: 1 in, 2 out]
                    }
                    event "SpectraPlot": Mouse Up {
                      n131 = event-data() -> ()  [unwired: 1 in, 1 out]
                      n132 = local read "Intercept"() -> (w189:dbl)
                      n133 = control-ref of="SpectraPlot"() -> (w191:refnum<vi>)
                      n134 = property class="WFGraph (strict)"(reference=w191, "Active Cursor"=u32 1, "Active Cursor"=u32 0) -> ("Cursor.Cursor X"=w197:dbl, "Cursor.Cursor X"=w196:dbl)  [unwired: 1 in, 2 out]
                      n135 = local read "Slope"() -> (w190:dbl)
                      n136 = local read "APPEARANCE_E/CH"() -> (w195:bool)
                      n137 = case shown="False" w195 {
                        tunnel: [w207 w213] -> w193
                        tunnel: [w206 w212] -> w192
                        tunnel: w190 -> [_ w209]
                        tunnel: w189 -> [_ w208]
                        tunnel: w197 -> [w207 w211]
                        tunnel: w196 -> [w206 w210]
                        frame False {
                        }
                        frame True {
                          n138 = call "SUB_EnergyToChannel.vi"("Intercept"=w208, "Slope"=w209, "Energy"=w211) -> ("Channel"=w213:u32)
                          n139 = call "SUB_EnergyToChannel.vi"("Intercept"=w208, "Slope"=w209, "Energy"=w210) -> ("Channel"=w212:u32)
                        }
                      }
                      n140 = Less?(x=w193, y=w192) -> (x < y?=w194:bool)
                      n141 = case shown="False" w194 {
                        tunnel: w193 -> [w202 w205]
                        tunnel: w192 -> [w203 w204]
                        tunnel: [w203 w205] -> w188
                        tunnel: [w202 w204] -> w187
                        frame False {
                        }
                        frame True {
                        }
                      }
                      n142 = local write "ROI_LowCh"(w188) -> ()
                      n143 = local write "ROI_UpCh"(w187) -> ()
                    }
                    event "ROI_LowCh", "ROI_UpCh": Value Change {
                      n144 = event-data() -> ()  [unwired: 1 in, 1 out]
                      n145 = local read "Intercept"() -> (w217:dbl)
                      n146 = local read "Slope"() -> (w222:dbl)
                      n147 = call "SUB_ChannelToEnergy.vi"("Intercept"=w217, "Channel"="ROI_UpCh", "Slope"=w222) -> ("Energy"=w219:dbl)
                      n148 = call "SUB_ChannelToEnergy.vi"("Intercept"=w217, "Channel"="ROI_LowCh", "Slope"=w222) -> ("Energy"=w218:dbl)
                      n149 = control-ref of="SpectraPlot"() -> (w216:refnum<vi>)
                      n150 = property class="WFGraph (strict)"(reference=w216, "Active Cursor"=u32 1, "Cursor.Cursor X"=w219, "Active Cursor"=u32 0, "Cursor.Cursor X"=w218) -> ()  [unwired: 1 in, 2 out]
                    }
                    event "ROI_Cancel": Mouse Up {
                      n151 = event-data() -> ()  [unwired: 1 in, 7 out]
                    }
                    event "ROI_Set": Mouse Up {
                      n152 = event-data() -> ()  [unwired: 1 in, 1 out]
                      n153 = call "Prompt User for Input"() -> ("ROI name"=w227:string)  [unwired: 17 in, 2 out]
                    }
                  }
                }
              }
              frame #2 {
                n154 = case shown="True" w231 {
                  tunnel: w230 -> [_ w234]
                  frame False {
                  }
                  frame True {
                    n155 = local read "ROI_LowCh"() -> (w232:u32)
                    n156 = local read "ROI_UpCh"() -> (w233:u32)
                    n157 = local read "Intercept"() -> (w237:dbl)
                    n158 = local read "SpectraPlot"() -> (w250:dbl[])
                    n159 = Reshape Array(w250, 2048 ("dimension size")) -> (w249:dbl[])
                    n160 = local read "Slope"() -> (w236:dbl)
                    n161 = call "SUB_FitROI.vi"("Array"=w249, "Lower"=w232, "Upper"=w233) -> ("Net"=w242:i32, "centroid"=w240:dbl, "FWHM"=w238:dbl, "Integral"=w241:i32, "sum"=w243:dbl)  [unwired: 1 in]
                    n162 = call "SUB_ChannelToEnergy.vi"("Intercept"=w237, "Channel"=w240, "Slope"=w236) -> ("Energy"=w239:dbl)
                    n163 = call "SUB_ChannelToEnergy.vi"("Intercept"=w237, "Channel"=w238, "Slope"=w236) -> ("Energy"=w235:dbl)
                    n164 = Bundle By Name(cluster=T16 {"ROI name"="", "ROI begin channel"=0, "ROI end channel"=0, "Intensity"=0, "Net Intensity"=0, "Gauss Fit"=0.0, "FWHM [keV]"=0.0, "Center [keV]"=0.0} ("input cluster"), "ROI name"=w234, "ROI begin channel"=w232, "ROI end channel"=w233, "Intensity"=w241, "Net Intensity"=w242, "Gauss Fit"=w243, "FWHM [keV]"=w235, "Center [keV]"=w239) -> (w245:T16)
                    n165 = local read "ROI_Array"() -> (w244:T10)
                    n166 = Insert Into Array(array=w244, new element=w245) -> (→"ROI_Array":T10)  [unwired: 1 in]
                  }
                }
              }
              frame #3 {
                w254 = T15."Disabled and Grayed Out" ("Disabled")
                w255 = T15."Enabled" ("Disabled")
                w259 = FALSE ("Cursor.Visible")
                n167 = control-ref of="ROI_RemoveAll"() -> (w251:refnum<vi>)
                n168 = control-ref of="ROI_Add"() -> (w253:refnum<vi>)
                n169 = control-ref of="ROI_Remove"() -> (w252:refnum<vi>)
                n170 = property on="ROI_Cancel" class="Bool (strict)"("DisabledEnum"=w254) -> ()  [unwired: 2 in, 2 out]
                n171 = property on="ROI_Set" class="Bool (strict)"("DisabledEnum"=w254) -> ()  [unwired: 2 in, 2 out]
                n172 = property on="Property Node" class="Bool"(reference=w252, "DisabledEnum"=w255) -> ()  [unwired: 1 in, 2 out]
                n173 = property on="Property Node" class="Bool"(reference=w253, "DisabledEnum"=w255) -> ()  [unwired: 1 in, 2 out]
                n174 = property on="Property Node" class="Bool"(reference=w251, "DisabledEnum"=w255) -> ()  [unwired: 1 in, 2 out]
                n175 = control-ref of="SpectraPlot"() -> (w256:refnum<vi>)
                n176 = property class="WFGraph (strict)"(reference=w256, "Active Cursor"=u32 1, "Cursor.Visible"=w259, "Active Cursor"=u32 0, "Cursor.Visible"=w259) -> ()  [unwired: 1 in, 2 out]
              }
              frame #4 {
                n177 = local read "ROI_Array"() -> (w266:T10)
                n178 = for {
                  tunnel: w266 -> [w268] mode=indexing
                  tunnel: [w267] -> w261 mode=indexing
                  n179 = Unbundle By Name(w268) -> ("ROI name"=w267:T8)
                }
                n180 = control-ref of="MAP-2"() -> (w264:refnum<vi>)
                n181 = control-ref of="MAP-1"() -> (w265:refnum<vi>)
                n182 = control-ref of="MAP-3"() -> (w263:refnum<vi>)
                n183 = property on="Property Node" class="Ring (strict)"(reference=w265, "Strings []"=w261) -> ()  [unwired: 1 in, 2 out]
                n184 = control-ref of="MAP-4"() -> (w262:refnum<vi>)
                n185 = control-ref of="MAP-4"() -> (w260:refnum<vi>)
                n186 = property on="Property Node" class="Ring (strict)"(reference=w264, "Strings []"=w261) -> ()  [unwired: 1 in, 2 out]
                n187 = property on="Property Node" class="Ring (strict)"(reference=w263, "Strings []"=w261) -> ()  [unwired: 1 in, 2 out]
                n188 = property on="Property Node" class="Ring (strict)"(reference=w262, "Strings []"=w261) -> ()  [unwired: 1 in, 2 out]
                n189 = property on="Property Node" class="Ring (strict)"(reference=w260, "Strings []"=w261) -> ()  [unwired: 1 in, 2 out]
              }
            }
          }
          event "ROI_Remove": Value Change {
            n190 = event-data() -> ()  [unwired: 1 in, 6 out]
            n191 = stacked-sequence {
              frame #0 {
                n192 = call "Prompt User for Input2"() -> ("ROI to delete (first is 0)"=w274:dbl, "OK"=w272:bool)  [unwired: 17 in, 1 out]
                n193 = local read "ROI_Array"() -> (w271:T10)
                n194 = case shown="True" w272 {
                  tunnel: w274 -> [_ w279]
                  tunnel: w271 -> [w275 w277]
                  tunnel: [w275 w276] -> w273
                  frame False {
                  }
                  frame True {
                    n195 = Delete From Array(array=w277, length=1, index=w279) -> (array with subset deleted=w276:T10)  [unwired: 1 out]
                  }
                }
                n196 = local write "ROI_Array"(w273) -> ()
              }
              frame #1 {
                n197 = local read "ROI_Array"() -> (w282:T10)
                n198 = for {
                  tunnel: w282 -> [w284] mode=indexing
                  tunnel: [w283] -> w281 mode=indexing
                  n199 = Unbundle By Name(w284) -> ("ROI name"=w283:T8)
                }
                n200 = control-ref of="MAP-1"() -> (w280:refnum<vi>)
                n201 = property on="Property Node" class="Ring (strict)"(reference=w280, "Strings []"=w281) -> ()  [unwired: 1 in, 2 out]
              }
            }
          }
          event "ROI_RemoveAll": Value Change {
            n202 = event-data() -> ()  [unwired: 1 in, 6 out]
            n203 = Two Button Dialog(message="Do you really want to remove all ROIs?", 1:"No" ("F button name (\"Cancel\")"), 2:"Yes" ("T button name (\"OK\")")) -> (T button?=w287:bool)
            n204 = case shown="True" w287 {
              frame False {
              }
              frame True {
                w298 = T15."Disabled and Grayed Out" ("Disabled")
                n205 = control-ref of="ROI_Remove"() -> (w291:refnum<vi>)
                n206 = control-ref of="ROI_RemoveAll"() -> (w292:refnum<vi>)
                n207 = Initialize Array(T16 {"ROI name"="", "ROI begin channel"=0, "ROI end channel"=0, "Intensity"=0, "Net Intensity"=0, "Gauss Fit"=0.0, "FWHM [keV]"=0.0, "Center [keV]"=0.0} ("input cluster")) -> (w296:T20)  [unwired: 1 in]
                n208 = property on="Property Node" class="Bool"(reference=w292, "DisabledEnum"=w298) -> ()  [unwired: 1 in, 2 out]
                n209 = property on="Property Node" class="Bool"(reference=w291, "DisabledEnum"=w298) -> ()  [unwired: 1 in, 2 out]
                n210 = local write "ROI_Array"(w296) -> ()
                n211 = Initialize Array("") -> (w294:string[])  [unwired: 1 in]
                n212 = control-ref of="MAP-1"() -> (w293:refnum<vi>)
                n213 = property on="Property Node" class="Ring (strict)"(reference=w293, "Strings []"=w294) -> ()  [unwired: 1 in, 2 out]
              }
            }
          }
          event "ROI_Save": Value Change {
            n214 = event-data() -> ("NewVal"=w299:bool)  [unwired: 1 in, 5 out]
            n215 = case shown="True" w299 {
              frame False {
              }
              frame True {
                n216 = local read "ROI_Array"() -> (w309:T10)
                n217 = for {
                  tunnel: w309 -> [w315] mode=indexing
                  tunnel: [w314] -> w308 mode=indexing
                  tunnel: [w312] -> w306 mode=indexing
                  tunnel: [w310] -> w307 mode=indexing
                  n218 = Unbundle By Name(w315) -> ("ROI name"=w314:T8, "ROI begin channel"=w313:T9, "ROI end channel"=w311:T9)
                  n219 = Number To Decimal String(number=w311) -> (decimal integer string=w310:string)  [unwired: 1 in]
                  n220 = Number To Decimal String(number=w313) -> (decimal integer string=w312:string)  [unwired: 1 in]
                }
                n221 = Build Array(w308, w306, w307) -> (w305:T8[][])
                n222 = call "File Dialog"("pattern (all files)"="*.roi") -> ("selected path"=w302:path)  [unwired: 11 in, 3 out]
                n223 = Transpose 2D Array(2D array=w305) -> (transposed array=w303:T8[][])
                n224 = call-poly <vilib>:"Write Delimited Spreadsheet.vi"("file path (dialog if empty)"=w302, "2D data"=w303) -> ()  [unwired: 12 in, 2 out]
              }
            }
          }
          event "ROI_Load": Value Change {
            n225 = event-data() -> ("NewVal"=w316:bool)  [unwired: 1 in, 5 out]
            n226 = case shown="True" w316 {
              frame False {
              }
              frame True {
                n227 = call-poly <vilib>:"Read Delimited Spreadsheet.vi"() -> ("all rows"=w324:string[][])  [unwired: 10 in, 5 out]
                n228 = for {
                  tunnel: w324 -> [w336] mode=indexing
                  tunnel: [w335] -> w325 mode=indexing
                  tunnel: [w334] -> w320 mode=indexing
                  n229 = Index Array(array=w336, index=0) -> (element=w334:string)
                  n230 = Index Array(array=w336, index=1) -> (element=w330:string)
                  n231 = Index Array(array=w336, index=2) -> (element=w329:string)
                  n232 = Decimal String To Number(string=w330) -> (number=w328:i32)  [unwired: 2 in, 1 out]
                  n233 = Decimal String To Number(string=w329) -> (number=w327:i32)  [unwired: 2 in, 1 out]
                  n234 = Bundle By Name(cluster=T16 {"ROI name"="", "ROI begin channel"=0, "ROI end channel"=0, "Intensity"=0, "Net Intensity"=0, "Gauss Fit"=0.0, "FWHM [keV]"=0.0, "Center [keV]"=0.0} ("input cluster"), "ROI name"=w334, "ROI begin channel"=w328, "ROI end channel"=w327) -> (w335:T16)
                }
                n235 = control-ref of="MAP-2"() -> (w322:refnum<vi>)
                n236 = control-ref of="MAP-3"() -> (w321:refnum<vi>)
                n237 = property on="Property Node" class="Ring (strict)"(reference=w322, "Strings []"=w320) -> ()  [unwired: 1 in, 2 out]
                n238 = property on="Property Node" class="Ring (strict)"(reference=w321, "Strings []"=w320) -> ()  [unwired: 1 in, 2 out]
                n239 = control-ref of="MAP-1"() -> (w323:refnum<vi>)
                n240 = control-ref of="MAP-4"() -> (w319:refnum<vi>)
                n241 = property on="Property Node" class="Ring (strict)"(reference=w323, "Strings []"=w320) -> ()  [unwired: 1 in, 2 out]
                n242 = property on="Property Node" class="Ring (strict)"(reference=w319, "Strings []"=w320) -> ()  [unwired: 1 in, 2 out]
                n243 = local write "ROI_Array"(w325) -> ()
              }
            }
          }
          event "CALIB_AddPoint": Value Change {
            n244 = event-data() -> ()  [unwired: 1 in, 6 out]
            n245 = control-ref of="SpectraPlot"() -> (w337:refnum<vi>)
            n246 = property on="Property Node" class="WFGraph (strict)"(reference=w337, "Active Cursor"=u32 2) -> ("Cursor.Cursor X"=w348:dbl)  [unwired: 1 in, 2 out]
            n247 = call "Enter the peak energy in keV."() -> ("Energy [keV]"=w340:dbl)  [unwired: 17 in, 2 out]
            n248 = Array Size(array="CalibArray") -> (size(s)=w344:i32[])
            n249 = Index Array(array=w344, index=0) -> (element=w339:i32)
            n250 = Increment(x=w339) -> (x+1=w346:i32)
            n251 = To Double Precision Float(number=w346) -> (double precision float=w341:dbl)
            n252 = Build Array(w341, w348, w340) -> (w342:dbl[])
            n253 = Insert Into Array(array="CalibArray", new element=w342) -> (w343:T7)  [unwired: 2 in]
            n254 = local write "CalibArray"(w343) -> ()
          }
          event "CALIB_ClearPoints": Value Change {
            n255 = event-data() -> ()  [unwired: 1 in, 6 out]
            n256 = local write "CalibArray"(T7 [] ("SIRIUS1_CalibArray")) -> ()
          }
          event "CALIB_Execute": Value Change {
            n257 = event-data() -> ()  [unwired: 1 in, 6 out]
            n258 = local read "CalibArray"() -> (w359:T7)
            n259 = Array Size(array=w359) -> (size(s)=w355:i32[])
            n260 = Index Array(array=w355, index=0) -> (element=w356:i32)
            n261 = Less Or Equal?(x=w356, y=1) -> (x <= y?=w358:bool)
            n262 = case shown="False" w358 {
              tunnel: w359 -> [w369 _]
              tunnel: w356 -> [w366 _]
              frame False {
                n263 = for {
                  N: w366 -> [_]
                  tunnel: [w372] -> w368 mode=indexing
                  tunnel: [w371] -> w367 mode=indexing
                  tunnel: w369 -> [w370]
                  i -> [w373]
                  n264 = Index Array(array=w370, index (row) #1=w373, index (col) #1=1 ("index (col)"), index (row) #2=w373, index (col) #2=2 ("index (col)")) -> (element #1=w372:dbl, element #2=w371:dbl)
                }
                n265 = Two Button Dialog(message="Calibration will done" ("warning IN"), 1:"Cancel" ("Cancel text"), 2:"Proceed" ("OK text")) -> (T button?=w362:bool)
                n266 = case shown="True" w362 {
                  tunnel: w368 -> [_ w380]
                  tunnel: w367 -> [_ w379]
                  frame False {
                  }
                  frame True {
                    w381 = T21 0 items=["Least Square", "Least Absolute Residual", "Bisquare"] ("method")
                    n267 = call <vilib>:"Linear Fit Coefficients.vi"("Y"=w379, "X"=w380, "method"=w381) -> ("slope"=→"Slope":dbl, "intercept"=→"Intercept":dbl)  [unwired: 10 in, 1 out]
                    n268 = local write "APPEARANCE_E/CH"(TRUE ("Energy/channels")) -> ()
                  }
                }
              }
              frame True {
                n269 = One Button Dialog(message="Calibration cannot be done: not enough points!") -> ()  [unwired: 1 in, 1 out]
              }
            }
          }
          event "X end [mm]", "PresetVal", "X accel", "X velocity [mm/s]", "step X [mm]", "Add acc dist [mm]": Value Change {
            n270 = event-data() -> ()  [unwired: 1 in, 6 out]
            n271 = local read "PresetVal"() -> (w425:u32)
            n272 = Divide(x=w425, y=1000.0 ("x")) -> (x/y=w423:dbl)
            n273 = Multiply(x="X accel", y=2.0) -> (x*y=w420:dbl)
            n274 = Subtract(x="X end [mm]", y="X start [mm]") -> (x-y=w412:dbl)
            n275 = Subtract(x="X end [mm]", y="X start [mm]") -> (x-y=w395:dbl)
            n276 = call "quotient.vi"("Y"="step X [mm]", "X"=w412) -> ("s? t:f"=w410:dbl, "x = y?"=w411:bool)  [unwired: 1 in]
            n277 = Divide(x=w412, y=w410) -> (x/y=w414:dbl)
            n278 = Absolute Value(x=w410) -> (abs(x)=w413:dbl)
            n279 = Select(t="step X [mm]", s=w411, f=w414) -> (s? t:f=w427:dbl)
            n280 = Divide(x=w427, y=w423) -> (x/y=w385:dbl)
            n281 = local write "X scan velocity [mm/s]"(w385) -> ()
            n282 = Square(x=w385) -> (x^2=w422:dbl)
            n283 = Divide(x=w422, y=w420) -> (x/y=w389:dbl)
            n284 = Subtract(x="X start [mm]", y=w389) -> (x-y=w416:dbl)
            n285 = Greater?(x=w385, y=w418) -> (0:→"X speed error":bool)
            n286 = Add(x="X end [mm]", y=w389) -> (x+y=w417:dbl)
            n287 = Multiply(x=w389, y=2.0) -> (x*y=w391:dbl)
            n288 = Add(x=w389, y="Add acc dist [mm]") -> (x+y=w388:dbl)
            n289 = Divide(x=w391, y="X accel") -> (x/y=w390:dbl)
            n290 = Square Root(x=w390) -> (sqrt(x)=w387:dbl)
            n291 = local write "Acc dist [mm]"(w388) -> ()
            n292 = Add(x=w395, y=w389) -> (x+y=w394:dbl)
            n293 = To Long Integer(number=w413) -> (32bit integer=w433:i32)
            n294 = Divide(x="Add acc dist [mm]", y=w385) -> (x/y=w383:dbl)
            n295 = Add(x=w394, y=w389) -> (x+y=w393:dbl)
            n296 = Add(x=w387, y=w383) -> (x+y=w386:dbl)
            n297 = Increment(x=w433) -> (x+1=w409:i32)
            "X steps" <- w409
            n298 = local read "X [mm]"() -> (w437:dbl)
            n299 = local write "Acc time [s]"(w386) -> ()
            n300 = Add(x=w437, y=w416) -> (x+y=w432:dbl)
            n301 = Add(x=w437, y=w417) -> (x+y=w431:dbl)
            n302 = Unbundle By Name(w429) -> ("X min"=w438:dbl, "X max"=w436:dbl)
            n303 = local write "X end [mm]"("X end [mm]") -> ()
            n304 = local write "step X [mm]"(w427) -> ()
            n305 = Less?(x=w432, y=w438) -> (x < y?=w434:bool)
            n306 = Greater?(x=w431, y=w436) -> (0:w435:bool)
            n307 = Divide(x=w393, y="X velocity [mm/s]") -> (x/y=w401:dbl)
            "Return movement time [s]" <- w401
            n308 = Or(x=w434, y=w435) -> (x .or. y?=→"X error":bool)
            n309 = local read "Y steps"() -> (w402:i32)
            n310 = Subtract(x="X end [mm]", y="X start [mm]") -> (x-y=w408:dbl)
            n311 = Divide(x=w408, y=w385) -> (x/y=w407:dbl)
            "Acq time [s]" <- w407
            n312 = Compound Arithmetic op=MULTIPLY(w409, w402) -> (→"total # of points":i32)
            n313 = Multiply(x=2.0, y=w387) -> (x*y=w406:dbl)
            n314 = Add(x=w406, y=w407) -> (x+y=w404:dbl)
            "Total line time [s]" <- w404
            n315 = Decrement(x=w402) -> (x-1=w403:i32)
            n316 = Multiply(x=w402, y=w404) -> (x*y=w399:dbl)
            n317 = Multiply(x=w403, y=w401) -> (x*y=w400:dbl)
            n318 = Add(x=w399, y=w400) -> (x+y=→"Total scan time [s]":dbl)
          }
          event "Y start [mm]", "Y end [mm]", "Y steps", "step Y [mm]": Value Change {
            n319 = event-data() -> ()  [unwired: 1 in, 6 out]
            n320 = Subtract(x="Y end [mm]", y="Y start [mm]") -> (x-y=w445:dbl)
            n321 = call "quotient.vi"("Y"="step Y [mm]", "X"=w445) -> ("s? t:f"=w443:dbl, "x = y?"=w444:bool)  [unwired: 1 in]
            n322 = Divide(x=w445, y=w443) -> (x/y=w446:dbl)
            n323 = Select(t="step Y [mm]", s=w444, f=w446) -> (s? t:f=w449:dbl)
            n324 = To Long Integer(number=w443) -> (32bit integer=w460:i32)
            n325 = local read "Y [mm]"() -> (w458:dbl)
            n326 = local write "Y end [mm]"("Y end [mm]") -> ()
            n327 = local write "step Y [mm]"(w449) -> ()
            n328 = Increment(x=w460) -> (x+1=w442:i32)
            "Y steps" <- w442
            n329 = local read "X steps"() -> (w459:i32)
            n330 = Unbundle By Name(w448) -> ("Y min"=w454:dbl, "Y max"=w453:dbl)
            n331 = Add(x=w458, y="Y start [mm]") -> (x+y=w451:dbl)
            n332 = Add(x=w458, y="Y end [mm]") -> (x+y=w450:dbl)
            n333 = Less?(x=w451, y=w454) -> (x < y?=w456:bool)
            n334 = Greater?(x=w450, y=w453) -> (0:w457:bool)
            n335 = Compound Arithmetic op=MULTIPLY(w442, w459) -> (w447:i32)
            n336 = Or(x=w456, y=w457) -> (x .or. y?=→"Y error":bool)
            n337 = local write "total # of points"(w447) -> ()
          }
          event "QUICKSCAN_Start": Value Change {
            n338 = event-data() -> ()  [unwired: 1 in, 6 out]
            n339 = stacked-sequence {
              tunnel: [w468 _] -> w465
              frame #0 {
                n340 = local read "X speed error"() -> (w473:T11)
                n341 = local read "X error"() -> (w471:T11)
                n342 = local read "Y error"() -> (w472:T11)
                n343 = Not(x=w471) -> (.not. x?=w474:T11)
                n344 = Not(x=w472) -> (.not. x?=w475:T11)
                n345 = Not(x=w473) -> (.not. x?=w476:T11)
                n346 = Compound Arithmetic op=AND(w474, w475, w476) -> (w467:T11)
                n347 = Select(t=fast_scanner."PrepareMap" ("Enum"), s=w467, f=fast_scanner."IDLE" ("Enum")) -> (s? t:f=w468:T1)
              }
              frame #1 {
                w479 = TRUE ("Boolean")
                n348 = local read "Shutter Port"() -> (w481:refnum<visa-resource-name>)
                n349 = local read "Servo Channel"() -> (w480:u8)
                n350 = control-ref of="Open Shutter"() -> (w477:refnum<vi>)
                n351 = call "LINX_servo.vi"("Servo Channel"=w480, "Serial Port"=w481, "Boolean"=w479) -> ("Shatter Open"=w478:bool)  [unwired: 8 in]
                n352 = property on="Property Node" class="Bool (strict)"(reference=w477, "Value"=w479) -> ()  [unwired: 1 in, 2 out]
                n353 = local write "Shutter Open"(w478) -> ()
              }
            }
          }
          event "Up": Value Change {
            n354 = event-data() -> ("NewVal"=w487:bool)  [unwired: 1 in, 5 out]
            n355 = local read "Assignment"() -> (w482:cluster{"Microstep Size":dbl, "Device":string}[])
            n356 = Index Array(array=w482, index=1) -> (element=w483:cluster{"Microstep Size":dbl, "Device":string})
            n357 = case shown="True" w487 {
              tunnel: w483 -> [_ w504]
              frame False {
                # "stop command"
                n358 = local read "Port"() -> (w490:refnum<visa-resource-name>)
                n359 = local read "ZaberError"() -> (w489:errorcluster)
                n360 = call "Stop.vi"("error in (no error)"=w489, "VISA resource name"=w490) -> ("error out"=w488:errorcluster)  [unwired: 8 in, 1 out]
                n361 = local write "ZaberError"(w488) -> ()
              }
              frame True {
                w502 = u16 2 items=["device units", "microns/s^2", "mm/s^2", "inches/s^2", "degrees/s^2"] ("Units (0: data)")
                w492 = u16 2 items=["device speed units", "microns per second", "millimeters per second", "inches per second", "degrees per second"] ("Units (0: device speed units)")
                # "move at specified velocity command"
                n362 = local read "Acceleration\n [mm/s^2]"() -> (w501:dbl)
                n363 = local read "ZaberError"() -> (w500:errorcluster)
                n364 = local read "Port"() -> (w499:refnum<visa-resource-name>)
                n365 = local read "XY Speed\n[mm/s]"() -> (w503:dbl)
                n366 = Negate(x=w503) -> (-x=w491:dbl)
                n367 = Unbundle(w504) -> ("Microstep Size"=w496:dbl, "Device"=w495:string)
                n368 = call "Set Acceleration.vi"("Units (0: data)"=w502, "New Acceleration"=w501, "error in (no error)"=w500, "Device and Axis"=w495, "Microstep Size (0)"=w496, "VISA resource name"=w499) -> ("error out"=w498:errorcluster, "VISA resource name out"=w497:refnum<visa-resource-name>)  [unwired: 4 in]
                n369 = call "Move at Velocity.vi"("Units (0: device speed units)"=w492, "Velocity"=w491, "error in (no error)"=w498, "Device and Axis"=w495, "Microstep Size (0)"=w496, "VISA resource name"=w497) -> ("error out"=w493:errorcluster, "VISA resource name out"=w494:refnum<visa-resource-name>)  [unwired: 4 in]
                n370 = while {
                  shift-right: [w509] -> _
                  shift-left: w494 -> [w512]
                  shift-right: [w510] -> w505
                  shift-left: w493 -> [w511]
                  tunnel: w504 -> [w508]
                  stop <- w515 stop-if-true
                  w514 = u16 2 items=["microsteps", "microns", "millimeters", "inches"] ("Units (0: microsteps)")
                  n371 = Unbundle(w508) -> ("Microstep Size"=w507:dbl, "Device"=w506:string)
                  n372 = Wait (ms)(milliseconds to wait=u32 100) -> ()  [unwired: 1 out]
                  n373 = call "Read Current Position.vi"("Units (0: microsteps)"=w514, "error in (no error)"=w511, "Device and Axis"=w506, "Microstep Size (0)"=w507, "VISA resource name"=w512) -> ("error out"=w510:errorcluster, "Position"=w513:dbl, "VISA resource name out"=w509:refnum<visa-resource-name>)  [unwired: 4 in]
                  n374 = Not(x="Up") -> (.not. x?=w515:bool)
                  n375 = local write "Y [mm]"(w513) -> ()
                }
                n376 = local write "ZaberError"(w505) -> ()
              }
            }
          }
          event "GoToY": Value Change {
            w519 = u16 2 items=["device units", "microns/s^2", "mm/s^2", "inches/s^2", "degrees/s^2"] ("Units (0: data)")
            w528 = u16 2 items=["device speed units", "microns per second", "millimeters per second", "inches per second", "degrees per second"] ("Units (0: device speed units)")
            w534 = u16 2 items=["microsteps", "microns", "millimeters", "inches", "degrees"] ("Units (0: microsteps)")
            w537 = u16 1 items=["relative", "absolute"] ("Movement Type (0: relative)")
            n377 = event-data() -> ()  [unwired: 1 in, 6 out]
            n378 = local read "Assignment"() -> (w533:cluster{"Microstep Size":dbl, "Device":string}[])
            n379 = Index Array(array=w533, index=1) -> (element=w530:cluster{"Microstep Size":dbl, "Device":string})
            n380 = local read "Port"() -> (w526:refnum<visa-resource-name>)
            n381 = local read "ZaberError"() -> (w529:errorcluster)
            n382 = local read "XY Speed\n[mm/s]"() -> (w527:dbl)
            n383 = Unbundle(w530) -> ("Microstep Size"=w525:dbl, "Device"=w524:string)
            n384 = local read "Acceleration\n [mm/s^2]"() -> (w518:dbl)
            n385 = call "Set Speed.vi"("Units (0: data)"=w528, "New Speed"=w527, "error in (no error)"=w529, "Device and Axis"=w524, "Microstep Size (0)"=w525, "VISA resource name"=w526) -> ("error out"=w523:errorcluster, "VISA resource name out"=w521:refnum<visa-resource-name>)  [unwired: 4 in]
            n386 = call "Set Acceleration.vi"("Units (0: data)"=w519, "New Acceleration"=w518, "error in (no error)"=w523, "Device and Axis"=w524, "Microstep Size (0)"=w525, "VISA resource name"=w521) -> ("error out"=w522:errorcluster, "VISA resource name out"=w520:refnum<visa-resource-name>)  [unwired: 4 in]
            n387 = Unbundle(w530) -> ("Microstep Size"=w532:dbl, "Device"=w531:string)
            n388 = call "Move.vi"("Units (0: microsteps)"=w534, "Movement Type (0: relative)"=w537, "Move Distance (0)"="GoTo Y [mm]", "error in (no error)"=w522, "Device and Axis"=w531, "Microstep Size (0)"=w532, "VISA resource name"=w520) -> ("error out"=w535:errorcluster)  [unwired: 3 in, 1 out]
            n389 = local write "ZaberError"(w535) -> ()
          }
          event "GoToX": Value Change {
            w542 = u16 2 items=["device units", "microns/s^2", "mm/s^2", "inches/s^2", "degrees/s^2"] ("Units (0: data)")
            w553 = u16 2 items=["device speed units", "microns per second", "millimeters per second", "inches per second", "degrees per second"] ("Units (0: device speed units)")
            w557 = u16 2 items=["microsteps", "microns", "millimeters", "inches", "degrees"] ("Units (0: microsteps)")
            w559 = u16 1 items=["relative", "absolute"] ("Movement Type (0: relative)")
            # "move to point command"
            n390 = event-data() -> ()  [unwired: 1 in, 6 out]
            n391 = local read "Assignment"() -> (w552:cluster{"Microstep Size":dbl, "Device":string}[])
            n392 = local read "XY Speed\n[mm/s]"() -> (w555:dbl)
            n393 = local read "Port"() -> (w554:refnum<visa-resource-name>)
            n394 = Index Array(array=w552, index=0) -> (element=w549:cluster{"Microstep Size":dbl, "Device":string})
            n395 = local read "ZaberError"() -> (w556:errorcluster)
            n396 = Unbundle(w549) -> ("Microstep Size"=w544:dbl, "Device"=w543:string)
            n397 = local read "Acceleration\n [mm/s^2]"() -> (w541:dbl)
            n398 = call "Set Speed.vi"("Units (0: data)"=w553, "New Speed"=w555, "error in (no error)"=w556, "Device and Axis"=w543, "Microstep Size (0)"=w544, "VISA resource name"=w554) -> ("error out"=w546:errorcluster, "VISA resource name out"=w548:refnum<visa-resource-name>)  [unwired: 4 in]
            n399 = call "Set Acceleration.vi"("Units (0: data)"=w542, "New Acceleration"=w541, "error in (no error)"=w546, "Device and Axis"=w543, "Microstep Size (0)"=w544, "VISA resource name"=w548) -> ("error out"=w545:errorcluster, "VISA resource name out"=w547:refnum<visa-resource-name>)  [unwired: 4 in]
            n400 = Unbundle(w549) -> ("Microstep Size"=w551:dbl, "Device"=w550:string)
            n401 = call "Move.vi"("Units (0: microsteps)"=w557, "Movement Type (0: relative)"=w559, "Move Distance (0)"="GoTo X [mm]", "error in (no error)"=w545, "Device and Axis"=w550, "Microstep Size (0)"=w551, "VISA resource name"=w547) -> ("error out"=w558:errorcluster)  [unwired: 3 in, 1 out]
            n402 = local write "ZaberError"(w558) -> ()
          }
          event "Home": Value Change {
            w577 = u16 2 items=["device units", "microns/s^2", "mm/s^2", "inches/s^2", "degrees/s^2"] ("Units (0: data)")
            w575 = u16 2 items=["device speed units", "microns per second", "millimeters per second", "inches per second", "degrees per second"] ("Units (0: device speed units)")
            w568 = u16 2 items=["microsteps", "microns", "millimeters", "inches", "degrees"] ("Units (0: microsteps)")
            w566 = u16 1 items=["relative", "absolute"] ("Movement Type (0: relative)")
            w604 = u16 2 items=["device units", "microns/s^2", "mm/s^2", "inches/s^2", "degrees/s^2"] ("Units (0: data)")
            w595 = u16 2 items=["device speed units", "microns per second", "millimeters per second", "inches per second", "degrees per second"] ("Units (0: device speed units)")
            w589 = u16 2 items=["microsteps", "microns", "millimeters", "inches", "degrees"] ("Units (0: microsteps)")
            w587 = u16 1 items=["relative", "absolute"] ("Movement Type (0: relative)")
            w564 = 0.0 ("Move Distance (0)")
            w626 = u16 2 items=["device units", "microns/s^2", "mm/s^2", "inches/s^2", "degrees/s^2"] ("Units (0: data)")
            w615 = u16 2 items=["device speed units", "microns per second", "millimeters per second", "inches per second", "degrees per second"] ("Units (0: device speed units)")
            w611 = u16 2 items=["microsteps", "microns", "millimeters", "inches", "degrees"] ("Units (0: microsteps)")
            w609 = u16 1 items=["relative", "absolute"] ("Movement Type (0: relative)")
            # "move to point command"
            # "move to point command"
            n403 = event-data() -> ()  [unwired: 1 in, 6 out]
            n404 = local read "Assignment"() -> (w616:cluster{"Microstep Size":dbl, "Device":string}[])
            n405 = local read "Assignment"() -> (w590:cluster{"Microstep Size":dbl, "Device":string}[])
            n406 = Index Array(array=w590, index=1) -> (element=w593:cluster{"Microstep Size":dbl, "Device":string})
            n407 = local read "Port"() -> (w597:refnum<visa-resource-name>)
            n408 = local read "XY Speed\n[mm/s]"() -> (w596:dbl)
            n409 = local read "XY Speed\n[mm/s]"() -> (w613:dbl)
            n410 = local read "ZaberError"() -> (w594:errorcluster)
            n411 = local read "Port"() -> (w614:refnum<visa-resource-name>)
            n412 = Index Array(array=w616, index=0) -> (element=w619:cluster{"Microstep Size":dbl, "Device":string})
            n413 = local read "ZaberError"() -> (w612:errorcluster)
            n414 = Unbundle(w593) -> ("Microstep Size"=w598:dbl, "Device"=w599:string)
            n415 = local read "Acceleration\n [mm/s^2]"() -> (w605:dbl)
            n416 = Unbundle(w619) -> ("Microstep Size"=w624:dbl, "Device"=w625:string)
            n417 = call "Set Speed.vi"("Units (0: data)"=w595, "New Speed"=w596, "error in (no error)"=w594, "Device and Axis"=w599, "Microstep Size (0)"=w598, "VISA resource name"=w597) -> ("error out"=w600:errorcluster, "VISA resource name out"=w602:refnum<visa-resource-name>)  [unwired: 4 in]
            n418 = call "Set Speed.vi"("Units (0: data)"=w615, "New Speed"=w613, "error in (no error)"=w612, "Device and Axis"=w625, "Microstep Size (0)"=w624, "VISA resource name"=w614) -> ("error out"=w622:errorcluster, "VISA resource name out"=w620:refnum<visa-resource-name>)  [unwired: 4 in]
            n419 = local read "Acceleration\n [mm/s^2]"() -> (w627:dbl)
            n420 = call "Set Acceleration.vi"("Units (0: data)"=w604, "New Acceleration"=w605, "error in (no error)"=w600, "Device and Axis"=w599, "Microstep Size (0)"=w598, "VISA resource name"=w602) -> ("error out"=w601:errorcluster, "VISA resource name out"=w603:refnum<visa-resource-name>)  [unwired: 4 in]
            n421 = call "Set Acceleration.vi"("Units (0: data)"=w626, "New Acceleration"=w627, "error in (no error)"=w622, "Device and Axis"=w625, "Microstep Size (0)"=w624, "VISA resource name"=w620) -> ("error out"=w623:errorcluster, "VISA resource name out"=w621:refnum<visa-resource-name>)  [unwired: 4 in]
            n422 = local read "Assignment"() -> (w569:cluster{"Microstep Size":dbl, "Device":string}[])
            n423 = Unbundle(w619) -> ("Microstep Size"=w617:dbl, "Device"=w618:string)
            n424 = local read "ZaberError"() -> (w576:errorcluster)
            n425 = Unbundle(w593) -> ("Microstep Size"=w591:dbl, "Device"=w592:string)
            n426 = call "Move.vi"("Units (0: microsteps)"=w611, "Movement Type (0: relative)"=w609, "Move Distance (0)"=w564, "error in (no error)"=w623, "Device and Axis"=w618, "Microstep Size (0)"=w617, "VISA resource name"=w621) -> ("error out"=w610:errorcluster)  [unwired: 3 in, 1 out]
            n427 = Index Array(array=w569, index=2) -> (element=w570:cluster{"Microstep Size":dbl, "Device":string})
            n428 = call "Move.vi"("Units (0: microsteps)"=w589, "Movement Type (0: relative)"=w587, "Move Distance (0)"=0.0, "error in (no error)"=w601, "Device and Axis"=w592, "Microstep Size (0)"=w591, "VISA resource name"=w603) -> ("error out"=w588:errorcluster)  [unwired: 3 in, 1 out]
            n429 = local write "ZaberError"(w610) -> ()
            n430 = local write "ZaberError"(w588) -> ()
            n431 = local read "Speed Z [mm/s]"() -> (w574:dbl)
            n432 = local read "Port"() -> (w573:refnum<visa-resource-name>)
            n433 = Unbundle(w570) -> ("Microstep Size"=w583:dbl, "Device"=w582:string)
            n434 = call "Set Speed.vi"("Units (0: data)"=w575, "New Speed"=w574, "error in (no error)"=w576, "Device and Axis"=w582, "Microstep Size (0)"=w583, "VISA resource name"=w573) -> ("error out"=w580:errorcluster, "VISA resource name out"=w578:refnum<visa-resource-name>)  [unwired: 4 in]
            n435 = local read "Acceleration\n [mm/s^2]"() -> (w584:dbl)
            n436 = call "Set Acceleration.vi"("Units (0: data)"=w577, "New Acceleration"=w584, "error in (no error)"=w580, "Device and Axis"=w582, "Microstep Size (0)"=w583, "VISA resource name"=w578) -> ("error out"=w581:errorcluster, "VISA resource name out"=w579:refnum<visa-resource-name>)  [unwired: 4 in]
            n437 = Unbundle(w570) -> ("Microstep Size"=w571:dbl, "Device"=w572:string)
            n438 = call "Move.vi"("Units (0: microsteps)"=w568, "Movement Type (0: relative)"=w566, "Move Distance (0)"=w564, "error in (no error)"=w581, "Device and Axis"=w572, "Microstep Size (0)"=w571, "VISA resource name"=w579) -> ("error out"=w567:errorcluster)  [unwired: 3 in, 1 out]
            n439 = local write "ZaberError"(w567) -> ()
          }
          event "GoToZ": Value Change {
            w636 = u16 2 items=["device units", "microns/s^2", "mm/s^2", "inches/s^2", "degrees/s^2"] ("Units (0: data)")
            w638 = u16 2 items=["device speed units", "microns per second", "millimeters per second", "inches per second", "degrees per second"] ("Units (0: device speed units)")
            w645 = u16 2 items=["microsteps", "microns", "millimeters", "inches", "degrees"] ("Units (0: microsteps)")
            w647 = u16 1 items=["relative", "absolute"] ("Movement Type (0: relative)")
            # "move to point command"
            n440 = event-data() -> ()  [unwired: 1 in, 6 out]
            n441 = disable-structure shown="Disabled" {
              disable-tunnel: [w653 _] -> _
              frame Disabled {
                n442 = local read "Prox. distance lower limit"() -> (w651:dbl)
                n443 = local read "Proximity distance"() -> (w652:dbl)
                n444 = Less?(x=w652, y=0.0) -> (x < y?=w654:bool)
                n445 = Greater Or Equal?(x=w652, y=w651) -> (x >= y?=w655:bool)
                n446 = Or(x=w654, y=w655) -> (x .or. y?=w653:bool)
              }
              frame Enabled {
              }
            }
            n447 = local read "Assignment"() -> (w644:cluster{"Microstep Size":dbl, "Device":string}[])
            n448 = local read "ZaberError"() -> (w637:errorcluster)
            n449 = Index Array(array=w644, index=2) -> (element=w643:cluster{"Microstep Size":dbl, "Device":string})
            n450 = local read "Speed Z [mm/s]"() -> (w639:dbl)
            n451 = local read "Port"() -> (w640:refnum<visa-resource-name>)
            n452 = Unbundle(w643) -> ("Microstep Size"=w630:dbl, "Device"=w631:string)
            n453 = call "Set Speed.vi"("Units (0: data)"=w638, "New Speed"=w639, "error in (no error)"=w637, "Device and Axis"=w631, "Microstep Size (0)"=w630, "VISA resource name"=w640) -> ("error out"=w633:errorcluster, "VISA resource name out"=w635:refnum<visa-resource-name>)  [unwired: 4 in]
            n454 = local read "Acceleration\n [mm/s^2]"() -> (w629:dbl)
            n455 = call "Set Acceleration.vi"("Units (0: data)"=w636, "New Acceleration"=w629, "error in (no error)"=w633, "Device and Axis"=w631, "Microstep Size (0)"=w630, "VISA resource name"=w635) -> ("error out"=w632:errorcluster, "VISA resource name out"=w634:refnum<visa-resource-name>)  [unwired: 4 in]
            n456 = local read "GoTo Z [mm]"() -> (w628:dbl)
            n457 = Unbundle(w643) -> ("Microstep Size"=w642:dbl, "Device"=w641:string)
            n458 = call "Move.vi"("Units (0: microsteps)"=w645, "Movement Type (0: relative)"=w647, "Move Distance (0)"=w628, "error in (no error)"=w632, "Device and Axis"=w641, "Microstep Size (0)"=w642, "VISA resource name"=w634) -> ("error out"=w646:errorcluster)  [unwired: 3 in, 1 out]
            n459 = local write "ZaberError"(w646) -> ()
          }
          event "StopMotion": Value Change {
            # "stop command"
            n460 = event-data() -> ()  [unwired: 1 in, 6 out]
            n461 = local read "Assignment"() -> (w660:cluster{"Microstep Size":dbl, "Device":string}[])
            n462 = local read "ZaberError"() -> (w658:errorcluster)
            n463 = local read "Port"() -> (w659:refnum<visa-resource-name>)
            n464 = for {
              tunnel: w660 -> [w664] mode=indexing
              shift-right: [w665] -> _
              shift-left: w659 -> [w668]
              shift-right: [w666] -> w657
              shift-left: w658 -> [w667]
              n465 = Unbundle(w664) -> ("Device"=w663:string)  [unwired: 1 out]
              n466 = call "Stop.vi"("error in (no error)"=w667, "Device and Axis"=w663, "VISA resource name"=w668) -> ("error out"=w666:errorcluster, "VISA resource name out"=w665:refnum<visa-resource-name>)  [unwired: 7 in]
            }
            n467 = local write "ZaberError"(w657) -> ()
          }
          event "Down": Value Change {
            n468 = event-data() -> ("NewVal"=w672:bool)  [unwired: 1 in, 5 out]
            n469 = local read "Assignment"() -> (w669:cluster{"Microstep Size":dbl, "Device":string}[])
            n470 = Index Array(array=w669, index=1) -> (element=w670:cluster{"Microstep Size":dbl, "Device":string})
            n471 = case shown="True" w672 {
              tunnel: w670 -> [_ w690]
              frame False {
                # "stop command"
                n472 = local read "Port"() -> (w677:refnum<visa-resource-name>)
                n473 = local read "ZaberError"() -> (w676:errorcluster)
                n474 = call "Stop.vi"("error in (no error)"=w676, "VISA resource name"=w677) -> ("error out"=w675:errorcluster)  [unwired: 8 in, 1 out]
                n475 = local write "ZaberError"(w675) -> ()
              }
              frame True {
                w689 = u16 2 items=["device units", "microns/s^2", "mm/s^2", "inches/s^2", "degrees/s^2"] ("Units (0: data)")
                w680 = u16 2 items=["device speed units", "microns per second", "millimeters per second", "inches per second", "degrees per second"] ("Units (0: device speed units)")
                # "move at specified velocity command"
                n476 = local read "Acceleration\n [mm/s^2]"() -> (w688:dbl)
                n477 = local read "ZaberError"() -> (w686:errorcluster)
                n478 = local read "Port"() -> (w687:refnum<visa-resource-name>)
                n479 = local read "XY Speed\n[mm/s]"() -> (w681:dbl)
                n480 = Unbundle(w690) -> ("Microstep Size"=w678:dbl, "Device"=w679:string)
                n481 = call "Set Acceleration.vi"("Units (0: data)"=w689, "New Acceleration"=w688, "error in (no error)"=w686, "Device and Axis"=w679, "Microstep Size (0)"=w678, "VISA resource name"=w687) -> ("error out"=w684:errorcluster, "VISA resource name out"=w685:refnum<visa-resource-name>)  [unwired: 4 in]
                n482 = call "Move at Velocity.vi"("Units (0: device speed units)"=w680, "Velocity"=w681, "error in (no error)"=w684, "Device and Axis"=w679, "Microstep Size (0)"=w678, "VISA resource name"=w685) -> ("error out"=w682:errorcluster, "VISA resource name out"=w683:refnum<visa-resource-name>)  [unwired: 4 in]
                n483 = while {
                  shift-right: [w696] -> _
                  shift-left: w683 -> [w699]
                  shift-right: [w697] -> w691
                  shift-left: w682 -> [w698]
                  tunnel: w690 -> [w692]
                  stop <- w702 stop-if-true
                  w701 = u16 2 items=["microsteps", "microns", "millimeters", "inches"] ("Units (0: microsteps)")
                  n484 = Wait (ms)(milliseconds to wait=u32 100) -> ()  [unwired: 1 out]
                  n485 = Unbundle(w692) -> ("Microstep Size"=w694:dbl, "Device"=w693:string)
                  n486 = call "Read Current Position.vi"("Units (0: microsteps)"=w701, "error in (no error)"=w698, "Device and Axis"=w693, "Microstep Size (0)"=w694, "VISA resource name"=w699) -> ("error out"=w697:errorcluster, "Position"=w700:dbl, "VISA resource name out"=w696:refnum<visa-resource-name>)  [unwired: 4 in]
                  n487 = Not(x="Down") -> (.not. x?=w702:bool)
                  n488 = local write "Y [mm]"(w700) -> ()
                }
                n489 = local write "ZaberError"(w691) -> ()
              }
            }
          }
          event "Closer": Value Change {
            n490 = event-data() -> ("NewVal"=w704:bool)  [unwired: 1 in, 5 out]
            n491 = case shown="False" w704 {
              tunnel: [FALSE ("VI stop") FALSE ("VI stop")] -> w706
              frame False {
                n492 = flat-sequence {
                  frame #0 {
                    n493 = local read "Assignment"() -> (w708:cluster{"Microstep Size":dbl, "Device":string}[])
                    n494 = local read "ZaberError"() -> (w710:errorcluster)
                    n495 = local read "Port"() -> (w709:refnum<visa-resource-name>)
                    n496 = for {
                      tunnel: w708 -> [w713] mode=indexing
                      shift-right: [w714] -> _
                      shift-left: w709 -> [w717]
                      shift-right: [w715] -> w711
                      shift-left: w710 -> [w716]
                      n497 = Unbundle(w713) -> ("Device"=w712:string)  [unwired: 1 out]
                      n498 = call "Stop.vi"("error in (no error)"=w716, "Device and Axis"=w712, "VISA resource name"=w717) -> ("error out"=w715:errorcluster, "VISA resource name out"=w714:refnum<visa-resource-name>)  [unwired: 7 in]
                    }
                    n499 = local write "ZaberError"(w711) -> ()
                  }
                }
              }
              frame True {
                w731 = u16 2 items=["device units", "microns/s^2", "mm/s^2", "inches/s^2", "degrees/s^2"] ("Units (0: data)")
                w725 = u16 2 items=["device speed units", "microns per second", "millimeters per second", "inches per second", "degrees per second"] ("Units (0: device speed units)")
                # "move at specified velocity command"
                n500 = disable-structure shown="Disabled" {
                  frame Disabled {
                    n501 = local read "Proximity distance"() -> (w749:dbl)
                    n502 = Greater?(x=w749, y=0.0) -> (0:w747:bool)
                    n503 = case shown="True" w747 {
                      tunnel: w749 -> [_ w755]
                      tunnel: [TRUE w758] -> _
                      frame False {
                      }
                      frame True {
                        n504 = local read "Prox. distance lower limit"() -> (w754:dbl)
                        n505 = local read "Proximity on"() -> (w759:bool)
                        n506 = Subtract(x=w755, y=w754) -> (x-y=w753:dbl)
                        n507 = Less Or Equal?(x=w753, y=15.0) -> (x <= y?=w751:bool)
                        n508 = Add(x=0.0, y=w754) -> (x+y=w757:dbl)
                        n509 = case shown="True" w751 {
                          frame False {
                          }
                          frame True {
                            n510 = local write "Speed Z [mm/s]"(1.0 ("Speed Z [mm/s]")) -> ()
                          }
                        }
                        n511 = Greater Or Equal?(x=w755, y=w757) -> (x >= y?=w760:bool)
                        n512 = And(x=w760, y=w759) -> (x .and. y?=w758:bool)
                      }
                    }
                  }
                  frame Enabled {
                  }
                }
                n513 = local read "Acceleration\n [mm/s^2]"() -> (w732:dbl)
                n514 = local read "Assignment"() -> (w721:cluster{"Microstep Size":dbl, "Device":string}[])
                n515 = local read "ZaberError"() -> (w729:errorcluster)
                n516 = local read "Speed Z [mm/s]"() -> (w719:dbl)
                n517 = local read "Port"() -> (w730:refnum<visa-resource-name>)
                n518 = Index Array(array=w721, index=2) -> (element=w720:cluster{"Microstep Size":dbl, "Device":string})
                n519 = Unbundle(w720) -> ("Microstep Size"=w727:dbl, "Device"=w726:string)
                n520 = call "Set Acceleration.vi"("Units (0: data)"=w731, "New Acceleration"=w732, "error in (no error)"=w729, "Device and Axis"=w726, "Microstep Size (0)"=w727, "VISA resource name"=w730) -> ("error out"=w728:errorcluster, "VISA resource name out"=w723:refnum<visa-resource-name>)  [unwired: 4 in]
                n521 = call "Move at Velocity.vi"("Units (0: device speed units)"=w725, "Velocity"=w719, "error in (no error)"=w728, "Device and Axis"=w726, "Microstep Size (0)"=w727, "VISA resource name"=w723) -> ("error out"=w724:errorcluster, "VISA resource name out"=w722:refnum<visa-resource-name>)  [unwired: 4 in]
                n522 = while {
                  shift-right: [w740] -> _
                  shift-left: w722 -> [w743]
                  shift-right: [w741] -> w733
                  shift-left: w724 -> [w742]
                  tunnel: w720 -> [w735]
                  stop <- w745 stop-if-true
                  w744 = u16 2 items=["microsteps", "microns", "millimeters", "inches"] ("Units (0: microsteps)")
                  n523 = Wait (ms)(milliseconds to wait=u32 10) -> ()  [unwired: 1 out]
                  n524 = Unbundle(w735) -> ("Microstep Size"=w737:dbl, "Device"=w736:string)
                  n525 = call "Read Current Position.vi"("Units (0: microsteps)"=w744, "error in (no error)"=w742, "Device and Axis"=w736, "Microstep Size (0)"=w737, "VISA resource name"=w743) -> ("error out"=w741:errorcluster, "Position"=w739:dbl, "VISA resource name out"=w740:refnum<visa-resource-name>)  [unwired: 4 in]
                  n526 = Not(x="Closer") -> (.not. x?=w745:bool)
                  n527 = local write "Z [mm]"(w739) -> ()
                }
                n528 = local write "ZaberError"(w733) -> ()
              }
            }
          }
          event "Left": Value Change {
            n529 = event-data() -> ("NewVal"=w763:bool)  [unwired: 1 in, 5 out]
            n530 = local read "Assignment"() -> (w762:cluster{"Microstep Size":dbl, "Device":string}[])
            n531 = Index Array(array=w762, index=0) -> (element=w764:cluster{"Microstep Size":dbl, "Device":string})
            n532 = case shown="True" w763 {
              tunnel: w764 -> [_ w783]
              frame False {
                # "stop command"
                n533 = local read "Port"() -> (w770:refnum<visa-resource-name>)
                n534 = local read "ZaberError"() -> (w769:errorcluster)
                n535 = call "Stop.vi"("error in (no error)"=w769, "VISA resource name"=w770) -> ("error out"=w768:errorcluster)  [unwired: 8 in, 1 out]
                n536 = local write "ZaberError"(w768) -> ()
              }
              frame True {
                w782 = u16 2 items=["device units", "microns/s^2", "mm/s^2", "inches/s^2", "degrees/s^2"] ("Units (0: data)")
                w772 = u16 2 items=["device speed units", "microns per second", "millimeters per second", "inches per second", "degrees per second"] ("Units (0: device speed units)")
                # "move at specified velocity command"
                n537 = local read "ZaberError"() -> (w779:errorcluster)
                n538 = local read "XY Speed\n[mm/s]"() -> (w784:dbl)
                n539 = local read "Port"() -> (w780:refnum<visa-resource-name>)
                n540 = Negate(x=w784) -> (-x=w771:dbl)
                n541 = local read "Acceleration\n [mm/s^2]"() -> (w781:dbl)
                n542 = Unbundle(w783) -> ("Microstep Size"=w774:dbl, "Device"=w773:string)
                n543 = call "Set Acceleration.vi"("Units (0: data)"=w782, "New Acceleration"=w781, "error in (no error)"=w779, "Device and Axis"=w773, "Microstep Size (0)"=w774, "VISA resource name"=w780) -> ("error out"=w777:errorcluster, "VISA resource name out"=w778:refnum<visa-resource-name>)  [unwired: 4 in]
                n544 = call "Move at Velocity.vi"("Units (0: device speed units)"=w772, "Velocity"=w771, "error in (no error)"=w777, "Device and Axis"=w773, "Microstep Size (0)"=w774, "VISA resource name"=w778) -> ("error out"=w775:errorcluster, "VISA resource name out"=w776:refnum<visa-resource-name>)  [unwired: 4 in]
                n545 = while {
                  shift-right: [w791] -> _
                  shift-left: w776 -> [w794]
                  shift-right: [w792] -> w785
                  shift-left: w775 -> [w793]
                  tunnel: w783 -> [w788]
                  stop <- w796 stop-if-true
                  w795 = u16 2 items=["microsteps", "microns", "millimeters", "inches"] ("Units (0: microsteps)")
                  n546 = Unbundle(w788) -> ("Microstep Size"=w787:dbl, "Device"=w786:string)
                  n547 = Wait (ms)(milliseconds to wait=u32 100) -> ()  [unwired: 1 out]
                  n548 = call "Read Current Position.vi"("Units (0: microsteps)"=w795, "error in (no error)"=w793, "Device and Axis"=w786, "Microstep Size (0)"=w787, "VISA resource name"=w794) -> ("error out"=w792:errorcluster, "Position"=w790:dbl, "VISA resource name out"=w791:refnum<visa-resource-name>)  [unwired: 4 in]
                  n549 = Not(x="Left") -> (.not. x?=w796:bool)
                  n550 = local write "X [mm]"(w790) -> ()
                }
                n551 = local write "ZaberError"(w785) -> ()
              }
            }
          }
          event "Right": Value Change {
            n552 = event-data() -> ("NewVal"=w799:bool)  [unwired: 1 in, 5 out]
            n553 = local read "Assignment"() -> (w798:cluster{"Microstep Size":dbl, "Device":string}[])
            n554 = Index Array(array=w798, index=0) -> (element=w800:cluster{"Microstep Size":dbl, "Device":string})
            n555 = case shown="True" w799 {
              tunnel: w800 -> [_ w819]
              frame False {
                # "stop command"
                n556 = local read "Port"() -> (w806:refnum<visa-resource-name>)
                n557 = local read "ZaberError"() -> (w805:errorcluster)
                n558 = call "Stop.vi"("error in (no error)"=w805, "VISA resource name"=w806) -> ("error out"=w804:errorcluster)  [unwired: 8 in, 1 out]
                n559 = local write "ZaberError"(w804) -> ()
              }
              frame True {
                w818 = u16 2 items=["device units", "microns/s^2", "mm/s^2", "inches/s^2", "degrees/s^2"] ("Units (0: data)")
                w808 = u16 2 items=["device speed units", "microns per second", "millimeters per second", "inches per second", "degrees per second"] ("Units (0: device speed units)")
                # "move at specified velocity command"
                n560 = local read "Acceleration\n [mm/s^2]"() -> (w817:dbl)
                n561 = local read "ZaberError"() -> (w816:errorcluster)
                n562 = local read "XY Speed\n[mm/s]"() -> (w807:dbl)
                n563 = local read "Port"() -> (w815:refnum<visa-resource-name>)
                n564 = Unbundle(w819) -> ("Microstep Size"=w810:dbl, "Device"=w809:string)
                n565 = call "Set Acceleration.vi"("Units (0: data)"=w818, "New Acceleration"=w817, "error in (no error)"=w816, "Device and Axis"=w809, "Microstep Size (0)"=w810, "VISA resource name"=w815) -> ("error out"=w814:errorcluster, "VISA resource name out"=w813:refnum<visa-resource-name>)  [unwired: 4 in]
                n566 = call "Move at Velocity.vi"("Units (0: device speed units)"=w808, "Velocity"=w807, "error in (no error)"=w814, "Device and Axis"=w809, "Microstep Size (0)"=w810, "VISA resource name"=w813) -> ("error out"=w811:errorcluster, "VISA resource name out"=w812:refnum<visa-resource-name>)  [unwired: 4 in]
                n567 = while {
                  shift-right: [w826] -> _
                  shift-left: w812 -> [w829]
                  shift-right: [w827] -> w820
                  shift-left: w811 -> [w828]
                  tunnel: w819 -> [w821]
                  stop <- w831 stop-if-true
                  w830 = u16 2 items=["microsteps", "microns", "millimeters", "inches"] ("Units (0: microsteps)")
                  n568 = Wait (ms)(milliseconds to wait=u32 100) -> ()  [unwired: 1 out]
                  n569 = Unbundle(w821) -> ("Microstep Size"=w823:dbl, "Device"=w822:string)
                  n570 = call "Read Current Position.vi"("Units (0: microsteps)"=w830, "error in (no error)"=w828, "Device and Axis"=w822, "Microstep Size (0)"=w823, "VISA resource name"=w829) -> ("error out"=w827:errorcluster, "Position"=w825:dbl, "VISA resource name out"=w826:refnum<visa-resource-name>)  [unwired: 4 in]
                  n571 = Not(x="Right") -> (.not. x?=w831:bool)
                  n572 = local write "X [mm]"(w825) -> ()
                }
                n573 = local write "ZaberError"(w820) -> ()
              }
            }
          }
          event "Away": Value Change {
            n574 = event-data() -> ("NewVal"=w834:bool)  [unwired: 1 in, 5 out]
            n575 = local read "Assignment"() -> (w833:cluster{"Microstep Size":dbl, "Device":string}[])
            n576 = Index Array(array=w833, index=2) -> (element=w835:cluster{"Microstep Size":dbl, "Device":string})
            n577 = case shown="True" w834 {
              tunnel: w835 -> [_ w854]
              frame False {
                # "stop command"
                n578 = local read "Port"() -> (w841:refnum<visa-resource-name>)
                n579 = local read "ZaberError"() -> (w840:errorcluster)
                n580 = call "Stop.vi"("error in (no error)"=w840, "VISA resource name"=w841) -> ("error out"=w839:errorcluster)  [unwired: 8 in, 1 out]
                n581 = local write "ZaberError"(w839) -> ()
              }
              frame True {
                w853 = u16 2 items=["device units", "microns/s^2", "mm/s^2", "inches/s^2", "degrees/s^2"] ("Units (0: data)")
                w847 = u16 2 items=["device speed units", "microns per second", "millimeters per second", "inches per second", "degrees per second"] ("Units (0: device speed units)")
                # "move at specified velocity command"
                n582 = local read "Acceleration\n [mm/s^2]"() -> (w852:dbl)
                n583 = local read "Speed Z [mm/s]"() -> (w855:dbl)
                n584 = local read "Port"() -> (w850:refnum<visa-resource-name>)
                n585 = local read "ZaberError"() -> (w851:errorcluster)
                n586 = Negate(x=w855) -> (-x=w846:dbl)
                n587 = Unbundle(w854) -> ("Microstep Size"=w849:dbl, "Device"=w848:string)
                n588 = call "Set Acceleration.vi"("Units (0: data)"=w853, "New Acceleration"=w852, "error in (no error)"=w851, "Device and Axis"=w848, "Microstep Size (0)"=w849, "VISA resource name"=w850) -> ("error out"=w844:errorcluster, "VISA resource name out"=w845:refnum<visa-resource-name>)  [unwired: 4 in]
                n589 = call "Move at Velocity.vi"("Units (0: device speed units)"=w847, "Velocity"=w846, "error in (no error)"=w844, "Device and Axis"=w848, "Microstep Size (0)"=w849, "VISA resource name"=w845) -> ("error out"=w843:errorcluster, "VISA resource name out"=w842:refnum<visa-resource-name>)  [unwired: 4 in]
                n590 = while {
                  shift-right: [w862] -> _
                  shift-left: w842 -> [w865]
                  shift-right: [w863] -> w856
                  shift-left: w843 -> [w864]
                  tunnel: w854 -> [w859]
                  stop <- w867 stop-if-true
                  w866 = u16 2 items=["microsteps", "microns", "millimeters", "inches"] ("Units (0: microsteps)")
                  n591 = Unbundle(w859) -> ("Microstep Size"=w858:dbl, "Device"=w857:string)
                  n592 = Wait (ms)(milliseconds to wait=u32 50) -> ()  [unwired: 1 out]
                  n593 = call "Read Current Position.vi"("Units (0: microsteps)"=w866, "error in (no error)"=w864, "Device and Axis"=w857, "Microstep Size (0)"=w858, "VISA resource name"=w865) -> ("error out"=w863:errorcluster, "Position"=w861:dbl, "VISA resource name out"=w862:refnum<visa-resource-name>)  [unwired: 4 in]
                  n594 = Not(x="Away") -> (.not. x?=w867:bool)
                  n595 = local write "Z [mm]"(w861) -> ()
                }
                n596 = local write "ZaberError"(w856) -> ()
              }
            }
          }
          event "Reduced Speed": Value Change {
            n597 = event-data() -> ("NewVal"=w883:bool)  [unwired: 1 in, 5 out]
            n598 = case shown="False" w883 {
              tunnel: [1.0 ("Minimum") 0.1 ("Minimum")] -> w880
              tunnel: [75.0 ("Minimum") 7.5 ("Minimum")] -> w879
              tunnel: [1.0 ("Minimum") 0.1 ("Minimum")] -> w878
              tunnel: [0.5 ("Minimum") 0.05 ("Minimum")] -> w871
              tunnel: [10.0 ("Minimum") 1.0 ("Minimum")] -> w870
              tunnel: [0.5 ("Minimum") 0.05 ("Minimum")] -> w869
              frame False {
                # "full speed"
              }
              frame True {
                # "reduced speed"
              }
            }
            n599 = property on="Speed Z [mm/s]" class="Slide (strict)"() -> ("Data Range"=w873:T22, "Scale.Range"=w872:T23)  [unwired: 2 in, 2 out]
            n600 = property on="XY Speed\n[mm/s]" class="Slide (strict)"() -> ("Data Range"=w885:T22, "Scale.Range"=w877:T23)  [unwired: 2 in, 2 out]
            n601 = Bundle By Name(cluster=w885, "Minimum"=w880, "Maximum"=w879, "Increment"=w878) -> (w884:T22)
            n602 = Bundle By Name(cluster=w877, "Minimum"=w880, "Maximum"=w879, "Increment"=w878) -> (w876:T23)
            n603 = Bundle By Name(cluster=w873, "Minimum"=w871, "Maximum"=w870, "Increment"=w869) -> (w875:T22)
            n604 = Bundle By Name(cluster=w872, "Minimum"=w871, "Maximum"=w870, "Increment"=w869) -> (w874:T23)
            n605 = property on="XY Speed\n[mm/s]" class="Slide (strict)"("Data Range"=w884, "Scale.Range"=w876) -> ()  [unwired: 2 in, 2 out]
            n606 = property on="Speed Z [mm/s]" class="Slide (strict)"("Data Range"=w875, "Scale.Range"=w874) -> ()  [unwired: 2 in, 2 out]
          }
          event Panel Close? {
            n607 = event-data() -> ()  [unwired: 1 in, 4 out]
            n608 = local read "Proximity on"() -> (w898:bool)
            n609 = local read "DANTE configured"() -> (w900:bool)
            n610 = case shown="True" w898 {
              tunnel: [fast_scanner."Close" ("Enum") fast_scanner."Close" ("Enum")] -> _
              frame False {
              }
              frame True {
                n611 = One Button Dialog(message="Close Proximity first") -> ()  [unwired: 1 in, 1 out]
                n612 = local write "Connect/Disconnect Prox"(FALSE ("Connect/Disconnect Prox")) -> ()
              }
            }
            n613 = case shown="True" w900 {
              tunnel: [fast_scanner."Close" ("Enum") fast_scanner."Close" ("Enum")] -> w899
              frame False {
              }
              frame True {
                n614 = One Button Dialog(message="Close DANTE first") -> ()  [unwired: 1 in, 1 out]
                n615 = local write "Close DANTE"(TRUE ("Close DANTE")) -> ()
              }
            }
            n616 = event-data("Discard?"=TRUE) -> ()  [unwired: 1 in, 1 out]
          }
          event "MEASUREMENT_Start": Value Change {
            w915 = TRUE ("Boolean")
            n617 = event-data() -> ()  [unwired: 1 in, 5 out]
            n618 = local read "Shutter Port"() -> (w913:refnum<visa-resource-name>)
            n619 = control-ref of="Open Shutter"() -> (w912:refnum<vi>)
            n620 = local read "Servo Channel"() -> (w914:u8)
            n621 = call "LINX_servo.vi"("Servo Channel"=w914, "Serial Port"=w913, "Boolean"=w915) -> ("Shatter Open"=w916:bool)  [unwired: 8 in]
            n622 = property on="Property Node" class="Bool (strict)"(reference=w912, "Value"=w915) -> ()  [unwired: 1 in, 2 out]
            n623 = local write "Shutter Open"(w916) -> ()
          }
          event "SaveSpectrum": Value Change {
            n624 = event-data() -> ()  [unwired: 1 in, 6 out]
          }
          event "APPEARANCE_CursorVis": Value Change {
            n625 = event-data() -> ("NewVal"=w920:bool)  [unwired: 1 in]
            n626 = control-ref of="SpectraPlot"() -> (w919:refnum<vi>)
            n627 = property on="Property Node" class="WFGraph (strict)"(reference=w919, "Cursor Palette Vis"=w920, "Active Cursor"=u32 2, "Cursor.Visible"=w920) -> ()  [unwired: 1 in, 2 out]
          }
          event "APPEARANCE_Log/Lin": Value Change {
            n628 = event-data() -> ("NewVal"=w927:bool)  [unwired: 1 in]
            n629 = Boolean To (0,1)(Boolean=w927) -> (0, 1=w925:i16)
            n630 = control-ref of="SpectraPlot"() -> (w924:refnum<vi>)
            n631 = property on="Property Node" class="WFGraph (strict)"(reference=w924, "YScale.Mapping Mode"=w925) -> ()  [unwired: 1 in, 2 out]
          }
          event "APPEARANCE_E/CH": Value Change {
            n632 = event-data() -> ("NewVal"=w929:bool)  [unwired: 1 in, 5 out]
            n633 = flat-sequence {
              tunnel: [w942] -> w934
              tunnel: [w941] -> w933
              tunnel: [w937] -> w932
              tunnel: [w938] -> w931
              tunnel: [w939] -> w930
              tunnel: w929 -> [w937]
              tunnel: w934 -> [w953]
              tunnel: w933 -> [w952]
              tunnel: w932 -> [w951]
              tunnel: w931 -> [w944]
              tunnel: w930 -> [w943]
              frame #0 {
                n634 = control-ref of="SpectraPlot"() -> (w938:refnum<vi>)
                n635 = property class="WFGraph (strict)"(reference=w938, "Active Cursor"=u32 2) -> ("Cursor.Cursor X"=w939:dbl)  [unwired: 1 in, 2 out]
                n636 = local read "Intercept"() -> (w941:dbl)
                n637 = local read "Slope"() -> (w942:dbl)
              }
              frame #1 {
                n638 = case shown="False" w951 {
                  tunnel: ["Channels" ("X Scale.Name Label.Text") "Energy (keV)"] -> w950
                  tunnel: [T17 {"Format"=0, "Precision"=0} ("X Scale.Display Format") T17 {"Format"=0, "Precision"=2} ("X Scale.Display Format")] -> w949
                  tunnel: [0.0 ("Energy 1st channel (keV)") w964] -> w947
                  tunnel: [1.0 ("Energy step (keV)") w963] -> w948
                  tunnel: [w957 w966] -> w946
                  tunnel: w952 -> [w955 w964]
                  tunnel: w953 -> [w954 w963]
                  tunnel: w943 -> [w956 w965]
                  frame False {
                    # "energy -> channels"
                    n639 = Subtract(x=w956, y=w955) -> (x-y=w958:dbl)
                    n640 = Divide(x=w958, y=w954) -> (x/y=w957:dbl)
                  }
                  frame True {
                    # "channels -> energy"
                    n641 = Multiply(x=w965, y=w963) -> (x*y=w967:dbl)
                    n642 = Add(x=w964, y=w967) -> (x+y=w966:dbl)
                  }
                }
                n643 = property class="WFGraph (strict)"(reference=w944, "XScale.NameLbl.Text"=w950, "XScale.Format & Precision"=w949, "XScale.Multiplier"=w948, "XScale.Offset"=w947, "Active Cursor"=u32 2, "Cursor.Cursor X"=w946) -> ()  [unwired: 1 in, 2 out]
              }
            }
          }
          event "MAP-1": Value Change {
            n644 = event-data() -> ()  [unwired: 1 in, 6 out]
            n645 = local read "2DSet"() -> (w972:dbl[][][])
            n646 = for {
              tunnel: w972 -> [w975] mode=indexing
              tunnel: "MAP-1" -> [w977]
              tunnel: [w975] -> w971
              i -> [w978]
              stop <- w976 stop-if-true
              n647 = Equal?(x=w977, y=w978) -> (x = y?=w976:bool)
            }
            "2D graph 1" <- w971
          }
          event "MAP-2": Value Change {
            n648 = event-data() -> ()  [unwired: 1 in, 6 out]
            n649 = local read "2DSet"() -> (w979:dbl[][][])
            n650 = for {
              tunnel: w979 -> [w984] mode=indexing
              tunnel: "MAP-2" -> [w986]
              tunnel: [w984] -> w980
              i -> [w987]
              stop <- w985 stop-if-true
              n651 = Equal?(x=w986, y=w987) -> (x = y?=w985:bool)
            }
            "2D graph 2" <- w980
          }
          event "MAP-3": Value Change {
            n652 = event-data() -> ()  [unwired: 1 in, 6 out]
            n653 = local read "2DSet"() -> (w988:dbl[][][])
            n654 = for {
              tunnel: w988 -> [w993] mode=indexing
              tunnel: "MAP-3" -> [w995]
              tunnel: [w993] -> w989
              i -> [w996]
              stop <- w994 stop-if-true
              n655 = Equal?(x=w995, y=w996) -> (x = y?=w994:bool)
            }
            "2D graph 3" <- w989
          }
          event "MAP-4": Value Change {
            n656 = event-data() -> ()  [unwired: 1 in, 6 out]
            n657 = local read "2DSet"() -> (w1000:dbl[][][])
            n658 = for {
              tunnel: w1000 -> [w1001] mode=indexing
              tunnel: "MAP-4" -> [w1003]
              tunnel: [w1001] -> w998
              i -> [w1004]
              stop <- w1002 stop-if-true
              n659 = Equal?(x=w1003, y=w1004) -> (x = y?=w1002:bool)
            }
            "2D graph 4" <- w998
          }
        }
      }
      frame "Acquire" {
        # "if not mapping plot last spectra on spectra plot"
        n660 = flat-sequence {
          tunnel: [w1008] -> w1005
          tunnel: w1005 -> [w1012]
          frame #0 {
            n661 = Tick Count (ms)() -> (millisecond timer value=w1008:u32)
          }
          frame #1 {
            n662 = control-ref of="Stop acq"() -> (w1009:refnum<vi>)
            n663 = control-ref of="Pause"() -> (w1010:refnum<vi>)
            n664 = while {
              tunnel: "Preset Time [s]" -> [w1024]
              tunnel: w1012 -> [w1027]
              tunnel: w1009 -> [_]
              stop <- w1020 stop-if-true
              n665 = Tick Count (ms)() -> (millisecond timer value=w1028:u32)
              n666 = local read "Pause"() -> (w1022:bool)
              n667 = Subtract(x=w1028, y=w1027) -> (x-y=w1026:u32)
              n668 = case shown="True" w1022 {
                frame False {
                }
                frame True {
                  n669 = while {
                    stop <- w1033 continue-if-true
                    n670 = local read "Pause"() -> (w1033:bool)
                    n671 = Wait (ms)(milliseconds to wait=u32 10) -> ()  [unwired: 1 out]
                  }
                }
              }
              n672 = Divide(x=w1026, y=u32 1000) -> (x/y=w1025:dbl)
              "Elapsed Time" <- w1025
              n673 = Divide(x=w1025, y=w1024) -> (x/y=w1031:dbl)
              n674 = Multiply(x=w1031, y=100.0) -> (x*y=→"Progress":dbl)
              n675 = local read "Stop acq"() -> (w1021:bool)
              n676 = Greater Or Equal?(x=w1025, y=w1024) -> (x >= y?=w1023:bool)
              n677 = Or(x=w1023, y=w1021) -> (x .or. y?=w1020:bool)
            }
            n678 = Multiply(x="Preset Time [s]", y=10.0) -> (x*y=w1014:dbl)
            n679 = local read "identifier out"() -> (w1016:string)
            n680 = control-ref of="SpectraPlot"() -> (w1019:refnum<vi>)
            n681 = control-ref of="Measurement On!"() -> (w1013:refnum<vi>)
            n682 = call "DANTE acquire single.vi"("Acq in progress"=w1013, "Single Spectrum"=w1019, "Pause button"=w1010, "Acquisition time [s]"=w1014, "Stop Button"=w1009, "identifier out"=w1016) -> ("stats out"=→"stats out":T6, "single spectrum"=→"SpectraPlot":dbl[])  [unwired: 4 in]
          }
          frame #2 {
            n683 = local read "Shutter Open"() -> (w1035:bool)
            n684 = case shown="True" w1035 {
              frame False {
              }
              frame True {
                w1038 = FALSE ("Pause")
                w1041 = FALSE ("Boolean")
                n685 = control-ref of="Open Shutter"() -> (w1037:refnum<vi>)
                n686 = local read "Shutter Port"() -> (w1039:refnum<visa-resource-name>)
                n687 = local read "Servo Channel"() -> (w1040:u8)
                n688 = call "LINX_servo.vi"("Servo Channel"=w1040, "Serial Port"=w1039, "Boolean"=w1041) -> ("Shatter Open"=w1042:bool)  [unwired: 8 in]
                n689 = property on="Property Node" class="Bool (strict)"(reference=w1037, "Value"=w1041) -> ()  [unwired: 1 in, 2 out]
                n690 = local write "Shutter Open"(w1042) -> ()
                n691 = property on="Pause" class="Bool (strict)"("Value"=w1038) -> ()  [unwired: 2 in, 2 out]
                n692 = property on="MEASUREMENT_Start" class="Bool (strict)"("Value"=w1038) -> ()  [unwired: 2 in, 2 out]
              }
            }
            n693 = property on="Stop acq" class="Bool (strict)"("Value"=FALSE ("Stop acq")) -> ()  [unwired: 2 in, 2 out]
          }
        }
      }
      frame "SaveSpectra" {
        n694 = stacked-sequence {
          frame #0 {
            n695 = local read "scan mode"() -> (w1051:bool)
            n696 = local read "Data folder path"() -> (w1053:path)
            n697 = Select(t=path "", s=w1051, f=w1053) -> (s? t:f=w1052:path)
            n698 = local read "SpectraPlot"() -> (w1049:dbl[])
            n699 = call "Spectrum name"() -> ("Name"=w1050:string)  [unwired: 17 in, 2 out]
            n700 = local read "X [mm]"() -> (w1048:dbl)
            n701 = local read "Z [mm]"() -> (w1046:dbl)
            n702 = local read "Y [mm]"() -> (w1047:dbl)
            n703 = call "SaveSpe.vi"("Z"=w1046, "Y"=w1047, "X"=w1048, "Spectrum"=w1049, "name"=w1050, "data folder path"=w1052) -> ()  [unwired: 2 in]
          }
          frame #1 {
          }
        }
      }
      frame "PrepareMap" {
        n704 = stacked-sequence {
          frame #0 {
            n705 = local read "X end [mm]"() -> (w1068:dbl)
            n706 = local read "X start [mm]"() -> (w1072:dbl)
            n707 = local read "Y start [mm]"() -> (w1076:dbl)
            n708 = local read "step Y [mm]"() -> (w1073:dbl)
            n709 = local read "X [mm]"() -> (w1067:dbl)
            n710 = local read "X [mm]"() -> (w1071:dbl)
            n711 = local read "Y [mm]"() -> (w1075:dbl)
            n712 = Add(x=w1068, y=w1067) -> (x+y=→"X end position":dbl)
            n713 = local read "Y steps"() -> (w1065:i32)
            "total line #" <- w1065
            n714 = Add(x=w1072, y=w1071) -> (x+y=→"X start position":dbl)
            n715 = Add(x=w1075, y=w1076) -> (x+y=w1074:dbl)
            n716 = for {
              N: w1065 -> [_]
              tunnel: w1074 -> [w1083]
              tunnel: w1073 -> [w1084]
              tunnel: [w1081] -> w1058 mode=indexing
              i -> [w1085]
              n717 = Multiply(x=w1084, y=w1085) -> (x*y=w1082:dbl)
              n718 = Add(x=w1083, y=w1082) -> (x+y=w1081:dbl)
            }
            "Y positions array" <- w1058
            n719 = local read "X steps"() -> (w1062:i32)
            n720 = local read "Y steps"() -> (w1061:i32)
            n721 = Increment(x=w1061) -> (x+1=w1060:i32)
            n722 = Initialize Array(u32 0 ("element"), w1062, w1060) -> (w1059:u32[][])
            n723 = Array Max & Min(array=w1058) -> (max value=→"Y end position":dbl, min value=→"Y start position":dbl)  [unwired: 2 out]
            n724 = local write "2D graph 1"(w1059) -> ()
            n725 = for {
              N: w1065 -> [_]
              tunnel: [w1078] -> w1064 mode=indexing
              n726 = Initialize Array(0.0 ("element"), 4 ("dimension size")) -> (w1078:dbl[])
            }
            "scan timing [ms]" <- w1064
            "scan mode" <- TRUE ("scan mode")
            "Line #" <- 1 ("Line #")
          }
          frame #1 {
            w1100 = 0.0 ("Z step")
            w1087 = u16 1 items=["X->Z->Y"=6, "Y->Z->X"=5, "Z->X->Y"=3, "Y->X->Z"=2, "Z->Y->X"=4, "X->Y->Z"=1] ("Order selection")
            n727 = local read "X start position"() -> (w1103:dbl)
            n728 = local read "Y start position"() -> (w1101:dbl)
            n729 = local read "X end position"() -> (w1102:dbl)
            n730 = local read "Y end position"() -> (w1099:dbl)
            n731 = local read "step Y [mm]"() -> (w1098:dbl)
            n732 = local read "step X [mm]"() -> (w1097:dbl)
            n733 = control-ref of="2D graph 1"() -> (w1109:refnum<vi>)
            n734 = Bundle By Name(cluster=T18 {"X abs start"=0.0, "X abs end"=0.0, "Y abs start"=0.0, "Y abs end"=0.0, "Z abs start"=0.0, "Z abs end"=0.0, "X step"=0.0, "Y step"=0.0, "Z step"=0.0} ("Scan\nCoords \n[mm]"), "X abs start"=w1103, "X abs end"=w1102, "Y abs start"=w1101, "Y abs end"=w1099, "Z abs start"=w1100, "Z abs end"=w1100, "X step"=w1098, "Y step"=w1097, "Z step"=w1100) -> (w1088:T18)
            n735 = control-ref of="2D graph 4"() -> (w1086:refnum<vi>)
            n736 = control-ref of="2D graph 2"() -> (w1096:refnum<vi>)
            n737 = call "Set2DPlots.vi"("error in (no error)"=errorcluster {"status"=FALSE, "code"=0, "source"=""}, "ScanCoords [mm]"=w1088, "Order selection"=w1087, "2D graph 3"=w1109) -> ("error out"=w1094:errorcluster, "initialized array"=w1106:dbl[][])
            n738 = call "Set2DPlots.vi"("error in (no error)"=w1094, "ScanCoords [mm]"=w1088, "Order selection"=w1087, "2D graph 3"=w1096) -> ("error out"=w1089:errorcluster)  [unwired: 1 out]
            n739 = local read "ROI_Array"() -> (w1107:T10)
            n740 = control-ref of="2D graph 3"() -> (w1095:refnum<vi>)
            n741 = call "Set2DPlots.vi"("error in (no error)"=w1089, "ScanCoords [mm]"=w1088, "Order selection"=w1087, "2D graph 3"=w1095) -> ()  [unwired: 2 out]
            n742 = call "Set2DPlots.vi"("error in (no error)"=w1089, "ScanCoords [mm]"=w1088, "Order selection"=w1087, "2D graph 3"=w1086) -> ()  [unwired: 2 out]
            n743 = Array Size(array=w1107) -> (size(s)=w1105:i32)
            n744 = for {
              N: w1105 -> [_]
              tunnel: w1106 -> [w1110]
              tunnel: [w1110] -> w1093 mode=indexing
            }
            "2DSet" <- w1093
            n745 = local read "Acq time [s]"() -> (w1090:dbl)
            n746 = Array Size(array=w1093) -> (size(s)=→"size(s)":i32[])
            n747 = property on="LineProgress" class="Slide (strict)"("Scale.Minimum"=0.0 ("Scale.Range:Minimum"), "Scale.Maximum"=w1090) -> ()  [unwired: 2 in, 2 out]
          }
          frame #2 {
            n748 = local read "total line #"() -> (w1112:i32)
            n749 = local read "X steps"() -> (w1111:i32)
            n750 = Initialize Array(0.0 ("element"), w1112, w1111) -> (w1113:dbl[][])
            n751 = local write "Z-coordinates_map"(w1113) -> ()
            n752 = local write "X-coordinates_map"(w1113) -> ()
            n753 = local write "Y-coordinates_map"(w1113) -> ()
          }
        }
      }
      frame "MoveToStartPoint" {
        n754 = stacked-sequence {
          frame #0 {
            w1123 = u16 2 items=["device units", "microns/s^2", "mm/s^2", "inches/s^2", "degrees/s^2"] ("Units (0: data)")
            w1131 = u16 2 items=["device speed units", "microns per second", "millimeters per second", "inches per second", "degrees per second"] ("Units (0: device speed units)")
            w1137 = u16 2 items=["microsteps", "microns", "millimeters", "inches", "degrees"] ("Units (0: microsteps)")
            w1139 = u16 1 items=["relative", "absolute"] ("Movement Type (0: relative)")
            n755 = local read "Line #"() -> (w1118:i32)
            n756 = local read "Y positions array"() -> (w1122:dbl[])
            n757 = local read "Assignment"() -> (w1136:cluster{"Microstep Size":dbl, "Device":string}[])
            n758 = Decrement(x=w1118) -> (x-1=w1117:i32)
            n759 = Index Array(array=w1122, index=w1117) -> (element=w1121:dbl)
            n760 = Index Array(array=w1136, index=1) -> (element=w1133:cluster{"Microstep Size":dbl, "Device":string})
            n761 = local read "Port"() -> (w1130:refnum<visa-resource-name>)
            n762 = local read "ZaberError"() -> (w1132:errorcluster)
            n763 = local read "X velocity [mm/s]"() -> (w1119:dbl)
            n764 = Unbundle(w1133) -> ("Microstep Size"=w1129:dbl, "Device"=w1128:string)
            n765 = call "Set Speed.vi"("Units (0: data)"=w1131, "New Speed"=w1119, "error in (no error)"=w1132, "Device and Axis"=w1128, "Microstep Size (0)"=w1129, "VISA resource name"=w1130) -> ("error out"=w1127:errorcluster, "VISA resource name out"=w1125:refnum<visa-resource-name>)  [unwired: 4 in]
            n766 = local read "X accel"() -> (w1120:dbl)
            n767 = call "Set Acceleration.vi"("Units (0: data)"=w1123, "New Acceleration"=w1120, "error in (no error)"=w1127, "Device and Axis"=w1128, "Microstep Size (0)"=w1129, "VISA resource name"=w1125) -> ("error out"=w1126:errorcluster, "VISA resource name out"=w1124:refnum<visa-resource-name>)  [unwired: 4 in]
            n768 = Unbundle(w1133) -> ("Microstep Size"=w1135:dbl, "Device"=w1134:string)
            n769 = call "Move.vi"("Units (0: microsteps)"=w1137, "Movement Type (0: relative)"=w1139, "Move Distance (0)"=w1121, "error in (no error)"=w1126, "Device and Axis"=w1134, "Microstep Size (0)"=w1135, "VISA resource name"=w1124) -> ("error out"=w1138:errorcluster)  [unwired: 3 in, 1 out]
            n770 = local write "ZaberError"(w1138) -> ()
          }
          frame #1 {
            w1146 = u16 2 items=["device units", "microns/s^2", "mm/s^2", "inches/s^2", "degrees/s^2"] ("Units (0: data)")
            w1157 = u16 2 items=["device speed units", "microns per second", "millimeters per second", "inches per second", "degrees per second"] ("Units (0: device speed units)")
            w1160 = u16 2 items=["microsteps", "microns", "millimeters", "inches", "degrees"] ("Units (0: microsteps)")
            w1162 = u16 1 items=["relative", "absolute"] ("Movement Type (0: relative)")
            # "move to point command"
            n771 = local read "Assignment"() -> (w1156:cluster{"Microstep Size":dbl, "Device":string}[])
            n772 = local read "Port"() -> (w1158:refnum<visa-resource-name>)
            n773 = Index Array(array=w1156, index=0) -> (element=w1153:cluster{"Microstep Size":dbl, "Device":string})
            n774 = local read "ZaberError"() -> (w1159:errorcluster)
            n775 = local read "X velocity [mm/s]"() -> (w1141:dbl)
            n776 = Unbundle(w1153) -> ("Microstep Size"=w1148:dbl, "Device"=w1147:string)
            n777 = call "Set Speed.vi"("Units (0: data)"=w1157, "New Speed"=w1141, "error in (no error)"=w1159, "Device and Axis"=w1147, "Microstep Size (0)"=w1148, "VISA resource name"=w1158) -> ("error out"=w1150:errorcluster, "VISA resource name out"=w1152:refnum<visa-resource-name>)  [unwired: 4 in]
            n778 = local read "X start position"() -> (w1145:dbl)
            n779 = local read "Acc dist [mm]"() -> (w1144:dbl)
            n780 = local read "X accel"() -> (w1142:dbl)
            n781 = call "Set Acceleration.vi"("Units (0: data)"=w1146, "New Acceleration"=w1142, "error in (no error)"=w1150, "Device and Axis"=w1147, "Microstep Size (0)"=w1148, "VISA resource name"=w1152) -> ("error out"=w1149:errorcluster, "VISA resource name out"=w1151:refnum<visa-resource-name>)  [unwired: 4 in]
            n782 = Subtract(x=w1145, y=w1144) -> (x-y=w1143:dbl)
            n783 = Unbundle(w1153) -> ("Microstep Size"=w1155:dbl, "Device"=w1154:string)
            n784 = call "Move.vi"("Units (0: microsteps)"=w1160, "Movement Type (0: relative)"=w1162, "Move Distance (0)"=w1143, "error in (no error)"=w1149, "Device and Axis"=w1154, "Microstep Size (0)"=w1155, "VISA resource name"=w1151) -> ("error out"=w1161:errorcluster)  [unwired: 3 in, 1 out]
            n785 = local write "ZaberError"(w1161) -> ()
          }
          frame #2 {
            # "wait till movement is completed"
            n786 = local read "Assignment"() -> (w1166:cluster{"Microstep Size":dbl, "Device":string}[])
            n787 = local read "ZaberError"() -> (w1169:errorcluster)
            n788 = local read "Port"() -> (w1170:refnum<visa-resource-name>)
            n789 = Index Array(array=w1166, index=0) -> (element=w1167:cluster{"Microstep Size":dbl, "Device":string})
            n790 = Index Array(array=w1166, index=1) -> (element=w1168:cluster{"Microstep Size":dbl, "Device":string})
            n791 = Unbundle(w1167) -> ("Device"=w1171:string)  [unwired: 1 out]
            n792 = call "Poll Until Idle.vi"("error in (no error)"=w1169, "Device and Axis"=w1171, "VISA resource name"=w1170) -> ("error out"=w1173:errorcluster, "VISA resource name out"=w1176:refnum<visa-resource-name>)  [unwired: 7 in]
            n793 = Unbundle(w1168) -> ("Device"=w1172:string)  [unwired: 1 out]
            n794 = call "Poll Until Idle.vi"("error in (no error)"=w1173, "Device and Axis"=w1172, "VISA resource name"=w1176) -> ("error out"=w1174:errorcluster, "VISA resource name out"=w1175:refnum<visa-resource-name>)  [unwired: 7 in]
            n795 = local write "Port"(w1175) -> ()
            n796 = local write "ZaberError"(w1174) -> ()
          }
        }
      }
      frame "AcquireLine" {
        # "spectra"
        # "stats"
        # "fullstats"
        # "Z"
        # "X"
        # "Y"
        n797 = stacked-sequence {
          seq-local: [w1180 _ _ _ _ _ _ _ _ _ _ _ _ _ _ _] -> [_ _ w1205 _ _ _ _ _ _ _ _ _ _ _ _ _]
          seq-local: [_ _ w1206 _ _ _ _ _ _ _ _ _ _ _ _ _] -> [_ _ _ _ w1213 _ _ _ _ _ _ _ _ _ _ _]
          seq-local: [_ _ _ _ w1214 _ _ _ _ _ _ _ _ _ _ _] -> [_ _ _ _ _ _ w1271 _ _ _ _ _ _ _ _ _]
          seq-local: [_ _ w1204 _ _ _ _ _ _ _ _ _ _ _ _ _] -> [_ _ _ _ _ _ _ _ _ _ _ _ _ w1362 _ _]
          seq-local: [_ _ _ _ _ _ w1270 _ _ _ _ _ _ _ _ _] -> [_ _ _ _ _ _ _ _ _ _ _ _ _ w1360 _ _]
          seq-local: [_ _ _ _ _ _ w1269 _ _ _ _ _ _ _ _ _] -> [_ _ _ _ _ _ _ _ w1280 _ _ _ _ _ _ _]
          seq-local: [_ _ _ _ _ _ _ _ w1279 _ _ _ _ _ _ _] -> [_ _ _ _ _ _ _ _ _ _ _ _ _ w1359 _ _]
          seq-local: [_ _ _ _ w1212 _ _ _ _ _ _ _ _ _ _ _] -> [_ _ _ _ _ _ _ _ _ _ _ _ _ w1361 _ _]
          seq-local: [_ _ _ _ _ w1227 _ _ _ _ _ _ _ _ _ _] -> [_ _ _ _ _ _ _ _ _ w1286 _ _ w1335 _ _ _]
          seq-local: [_ _ _ _ _ w1225 _ _ _ _ _ _ _ _ _ _] -> [_ _ _ _ _ _ _ _ _ _ _ _ w1351 _ _ _]
          seq-local: [_ _ _ _ _ w1224 _ _ _ _ _ _ _ _ _ _] -> [_ _ _ _ _ _ _ _ _ _ _ _ w1344 _ _ _]
          seq-local: [_ _ _ _ _ _ _ _ _ w1284 _ _ _ _ _ _] -> [_ _ _ _ _ _ _ _ _ _ w1298 _ _ _ _ _]
          seq-local: [_ _ _ _ _ w1218 _ _ _ _ _ _ _ _ _ _] -> [_ _ _ _ _ _ _ _ _ _ _ w1328 _ _ _ _]
          seq-local: [_ _ _ _ _ w1217 _ _ _ _ _ _ _ _ _ _] -> [_ _ _ _ _ _ _ _ _ _ _ w1326 _ _ _ _]
          seq-local: [_ _ _ _ _ w1216 _ _ _ _ _ _ _ _ _ _] -> [_ _ _ _ _ _ _ _ _ _ _ w1325 _ _ _ _]
          tunnel: w1177 -> [_ _ _ _ _ _ _ _ _ _ _ _ w1334 _ w1373 _]
          frame #0 {
            n798 = Tick Count (ms)() -> (millisecond timer value=w1180:u32)
          }
          frame #1 {
            w1203 = u16 2 items=["device units", "microns/s^2", "mm/s^2", "inches/s^2", "degrees/s^2"] ("Units (0: data)")
            w1192 = u16 2 items=["device speed units", "microns per second", "millimeters per second", "inches per second", "degrees per second"] ("Units (0: device speed units)")
            w1189 = u16 2 items=["microsteps", "microns", "millimeters", "inches", "degrees"] ("Units (0: microsteps)")
            w1187 = u16 1 items=["relative", "absolute"] ("Movement Type (0: relative)")
            n799 = local read "Assignment"() -> (w1193:cluster{"Microstep Size":dbl, "Device":string}[])
            n800 = local read "Port"() -> (w1191:refnum<visa-resource-name>)
            n801 = Index Array(array=w1193, index=0) -> (element=w1196:cluster{"Microstep Size":dbl, "Device":string})
            n802 = local read "ZaberError"() -> (w1190:errorcluster)
            n803 = local read "X scan velocity [mm/s]"() -> (w1185:dbl)
            n804 = local read "X accel"() -> (w1184:dbl)
            n805 = Unbundle(w1196) -> ("Microstep Size"=w1201:dbl, "Device"=w1202:string)
            n806 = call "Set Speed.vi"("Units (0: data)"=w1192, "New Speed"=w1185, "error in (no error)"=w1190, "Device and Axis"=w1202, "Microstep Size (0)"=w1201, "VISA resource name"=w1191) -> ("error out"=w1199:errorcluster, "VISA resource name out"=w1197:refnum<visa-resource-name>)  [unwired: 4 in]
            n807 = local read "Acc dist [mm]"() -> (w1181:dbl)
            n808 = local read "X end position"() -> (w1182:dbl)
            n809 = call "Set Acceleration.vi"("Units (0: data)"=w1203, "New Acceleration"=w1184, "error in (no error)"=w1199, "Device and Axis"=w1202, "Microstep Size (0)"=w1201, "VISA resource name"=w1197) -> ("error out"=w1200:errorcluster, "VISA resource name out"=w1198:refnum<visa-resource-name>)  [unwired: 4 in]
            n810 = Add(x=w1182, y=w1181) -> (x+y=w1183:dbl)
            n811 = Unbundle(w1196) -> ("Microstep Size"=w1194:dbl, "Device"=w1195:string)
            n812 = call "Move.vi"("Units (0: microsteps)"=w1189, "Movement Type (0: relative)"=w1187, "Move Distance (0)"=w1183, "error in (no error)"=w1200, "Device and Axis"=w1195, "Microstep Size (0)"=w1194, "VISA resource name"=w1198) -> ("error out"=w1188:errorcluster)  [unwired: 3 in, 1 out]
            n813 = local write "ZaberError"(w1188) -> ()
          }
          frame #2 {
            n814 = Tick Count (ms)() -> (millisecond timer value=w1206:u32)
            n815 = Subtract(x=w1206, y=w1205) -> (x-y=w1204:u32)
          }
          frame #3 {
            n816 = local read "Acc time [s]"() -> (w1209:dbl)
            n817 = Multiply(x=1000.0 ("y"), y=w1209) -> (x*y=w1208:dbl)
            n818 = Add(x="AcqStartDelay", y=w1208) -> (x+y=w1207:dbl)
            n819 = Wait (ms)(milliseconds to wait=w1207) -> ()  [unwired: 1 out]
          }
          frame #4 {
            n820 = Tick Count (ms)() -> (millisecond timer value=w1214:u32)
            n821 = Subtract(x=w1214, y=w1213) -> (x-y=w1212:u32)
          }
          frame #5 {
            w1219 = dbl[] []
            # "acquisition command + waiting till acquisition is done (subVI is suppose to stop after finish)"
            n822 = control-ref of="Pause scan"() -> (w1215:refnum<vi>)
            n823 = Multiply(x="PresetVal", y=10.0) -> (x*y=w1223:dbl)
            n824 = local read "X steps"() -> (w1220:i32)
            n825 = local read "identifier out"() -> (w1229:string)
            n826 = call "DANTE acquire multiple.vi"("Number of boards in chain"=u8 1, "Map points"=w1220, "Time per spectrum [ms]"=w1223, "Pause button 2"=w1215, "identifier out"=w1229) -> ("Statistics"=w1225:dbl[][], "spectra"=w1227:u16[][], "adv stats"=w1224:u64[][])  [unwired: 4 in]
            n827 = for {
              N: w1220 -> [_]
              tunnel: "PresetVal" -> [w1261]
              shift-right: [w1259] -> w1218
              shift-left: w1219 -> [w1260]
              shift-right: [w1234] -> w1217
              shift-left: w1219 -> [w1235]
              shift-right: [w1231] -> w1216
              shift-left: w1219 -> [w1232]
              w1247 = u16 2 items=["microsteps", "microns", "millimeters", "inches"] ("Units (0: microsteps)")
              n828 = local read "Assignment"() -> (w1248:cluster{"Microstep Size":dbl, "Device":string}[])
              n829 = local read "ZaberError"() -> (w1238:errorcluster)
              n830 = local read "Port"() -> (w1237:refnum<visa-resource-name>)
              n831 = Index Array(array=w1248, index=0) -> (element=w1249:cluster{"Microstep Size":dbl, "Device":string})
              n832 = Index Array(array=w1248, index=1) -> (element=w1253:cluster{"Microstep Size":dbl, "Device":string})
              n833 = Index Array(array=w1248, index=2) -> (element=w1257:cluster{"Microstep Size":dbl, "Device":string})
              n834 = Unbundle(w1249) -> ("Microstep Size"=w1250:dbl, "Device"=w1251:string)
              n835 = call "Read Current Position.vi"("Units (0: microsteps)"=w1247, "error in (no error)"=w1238, "Device and Axis"=w1251, "Microstep Size (0)"=w1250, "VISA resource name"=w1237) -> ("error out"=w1239:errorcluster, "Position"=w1233:dbl, "VISA resource name out"=w1240:refnum<visa-resource-name>)  [unwired: 4 in]
              n836 = local read "Proximity distance"() -> (w1258:dbl)
              n837 = Unbundle(w1253) -> ("Microstep Size"=w1252:dbl, "Device"=w1254:string)
              n838 = call "Read Current Position.vi"("Units (0: microsteps)"=w1247, "error in (no error)"=w1239, "Device and Axis"=w1254, "Microstep Size (0)"=w1252, "VISA resource name"=w1240) -> ("error out"=w1241:errorcluster, "Position"=w1230:dbl, "VISA resource name out"=w1242:refnum<visa-resource-name>)  [unwired: 4 in]
              n839 = Unbundle(w1257) -> ("Microstep Size"=w1255:dbl, "Device"=w1256:string)
              n840 = Wait (ms)(milliseconds to wait=w1261) -> ()  [unwired: 1 out]
              n841 = call "Read Current Position.vi"("Units (0: microsteps)"=w1247, "error in (no error)"=w1241, "Device and Axis"=w1256, "Microstep Size (0)"=w1255, "VISA resource name"=w1242) -> ("error out"=w1243:errorcluster, "Position"=w1236:dbl)  [unwired: 4 in, 1 out]
              n842 = Build Array (concatenate)(w1260, w1258) -> (w1259:dbl[])
              n843 = Build Array (concatenate)(w1235, w1233) -> (w1234:dbl[])
              n844 = Build Array (concatenate)(w1232, w1230) -> (w1231:dbl[])
              n845 = local write "ZaberError"(w1243) -> ()
              n846 = local write "X [mm]"(w1233) -> ()
              n847 = local write "Y [mm]"(w1230) -> ()
              n848 = local write "Z [mm]"(w1236) -> ()
            }
            n849 = local read "Acq time [s]"() -> (w1222:dbl)
            n850 = while {
              tunnel: w1222 -> [w1265]
              tunnel: "PresetVal" -> [w1263]
              i -> [w1268]
              stop <- w1264 stop-if-true
              n851 = Multiply(x=w1263, y=w1268) -> (x*y=w1267:u32)
              n852 = Wait (ms)(milliseconds to wait=w1263) -> ()  [unwired: 1 out]
              n853 = Divide(x=w1267, y=u32 1000) -> (x/y=w1262:dbl)
              "LineProgress" <- w1262
              n854 = Greater?(x=w1262, y=w1265) -> (0:w1264:bool)
            }
          }
          frame #6 {
            n855 = Tick Count (ms)() -> (millisecond timer value=w1269:u32)
            n856 = Subtract(x=w1269, y=w1271) -> (x-y=w1270:u32)
          }
          frame #7 {
            # "waiting till movement is completed - decelleration"
            n857 = local read "Assignment"() -> (w1276:cluster{"Microstep Size":dbl, "Device":string}[])
            n858 = Index Array(array=w1276, index=0) -> (element=w1277:cluster{"Microstep Size":dbl, "Device":string})
            n859 = local read "ZaberError"() -> (w1273:errorcluster)
            n860 = local read "Port"() -> (w1278:refnum<visa-resource-name>)
            n861 = Unbundle(w1277) -> ("Device"=w1274:string)  [unwired: 1 out]
            n862 = call "Poll Until Idle.vi"("error in (no error)"=w1273, "Device and Axis"=w1274, "VISA resource name"=w1278) -> ("error out"=w1272:errorcluster)  [unwired: 7 in, 1 out]
            n863 = local write "ZaberError"(w1272) -> ()
          }
          frame #8 {
            n864 = Tick Count (ms)() -> (millisecond timer value=w1281:u32)
            n865 = Subtract(x=w1281, y=w1280) -> (x-y=w1279:u32)
          }
          frame #9 {
            # "saving data"
            n866 = local read "ROI_Array"() -> (w1287:T10)
            n867 = local read "Line #"() -> (w1282:i32)
            n868 = Decrement(x=w1282) -> (x-1=w1283:i32)
            n869 = local read "2DSet"() -> (w1285:dbl[][][])
            n870 = for {
              tunnel: [w1297] -> w1288
              tunnel: w1287 -> [w1296] mode=indexing
              tunnel: w1286 -> [w1293]
              tunnel: w1285 -> [w1292] mode=indexing
              tunnel: w1283 -> [w1289]
              tunnel: [w1290] -> w1284 mode=indexing
              n871 = Unbundle By Name(w1296) -> ("ROI begin channel"=w1295:T9, "ROI end channel"=w1294:T9)
              n872 = call "Extract LineData.vi"("ROI End"=w1294, "Input Data"=w1293, "ROI Beg"=w1295) -> ("ROI Data"=w1291:u32[], "Sum spectra"=w1297:u32[])  [unwired: 1 out]
              n873 = Replace Array Subset(array=w1292, new element=w1291, index (col)=w1289) -> (w1290:dbl[][])  [unwired: 1 in]
            }
            "Sum spectra per line" <- w1288
            n874 = local write "2DSet"(w1284) -> ()
            "Spectra" <- w1286
          }
          frame #10 {
            n875 = local read "MAP-4"() -> (w1300:u16)
            n876 = local read "MAP-1"() -> (w1305:u16)
            n877 = local read "MAP-2"() -> (w1303:u16)
            n878 = local read "MAP-3"() -> (w1302:u16)
            n879 = for {
              tunnel: w1298 -> [w1319] mode=indexing
              tunnel: w1305 -> [w1321]
              tunnel: [w1319] -> w1306
              i -> [w1322]
              stop <- w1320 stop-if-true
              n880 = Equal?(x=w1321, y=w1322) -> (x = y?=w1320:bool)
            }
            n881 = for {
              tunnel: w1298 -> [w1311] mode=indexing
              tunnel: w1302 -> [w1313]
              tunnel: [w1311] -> w1301
              i -> [w1314]
              stop <- w1312 stop-if-true
              n882 = Equal?(x=w1313, y=w1314) -> (x = y?=w1312:bool)
            }
            n883 = for {
              tunnel: w1298 -> [w1307] mode=indexing
              tunnel: w1300 -> [w1309]
              tunnel: [w1307] -> w1299
              i -> [w1310]
              stop <- w1308 stop-if-true
              n884 = Equal?(x=w1309, y=w1310) -> (x = y?=w1308:bool)
            }
            n885 = for {
              tunnel: w1298 -> [w1315] mode=indexing
              tunnel: w1303 -> [w1317]
              tunnel: [w1315] -> w1304
              i -> [w1318]
              stop <- w1316 stop-if-true
              n886 = Equal?(x=w1317, y=w1318) -> (x = y?=w1316:bool)
            }
            n887 = local write "2D graph 1"(w1306) -> ()
            n888 = local write "2D graph 2"(w1304) -> ()
            n889 = local write "2D graph 3"(w1301) -> ()
            n890 = local write "2D graph 4"(w1299) -> ()
          }
          frame #11 {
            n891 = local read "Z-coordinates_map"() -> (w1329:dbl[][])
            n892 = local read "X-coordinates_map"() -> (w1330:dbl[][])
            n893 = local read "Y-coordinates_map"() -> (w1331:dbl[][])
            n894 = local read "Line #"() -> (w1332:i32)
            n895 = Decrement(x=w1332) -> (x-1=w1333:i32)
            n896 = Replace Array Subset(array=w1331, new element=w1325, index (row)=w1333) -> (w1323:dbl[][])  [unwired: 1 in]
            n897 = Replace Array Subset(array=w1329, new element=w1328, index (row)=w1333) -> (w1327:dbl[][])  [unwired: 1 in]
            n898 = Replace Array Subset(array=w1330, new element=w1326, index (row)=w1333) -> (w1324:dbl[][])  [unwired: 1 in]
            n899 = local write "Z-coordinates_map"(w1327) -> ()
            n900 = local write "X-coordinates_map"(w1324) -> ()
            n901 = local write "Y-coordinates_map"(w1323) -> ()
          }
          frame #12 {
            w1343 = "Map_" ("string")
            w1338 = ";"
            n902 = Get Date/Time In Seconds() -> (seconds since 1Jan1904=w1348:timestamp)
            n903 = local read "Line #"() -> (w1345:i32)
            n904 = call "csv_names.vi"("Numeric"=w1345) -> ("concatenated string"=w1337:string)  [unwired: 1 in]
            n905 = Format Date/Time String(time format string (%c)="%04Y_%02m_%02d_%02H_%02M_%S_", seconds (now)=w1348, UTC format=FALSE ("want seconds? (F)")) -> (date/time string=w1342:string)
            n906 = Concatenate Strings(w1343, w1342, w1337, "_spectr.csv" ("string")) -> (w1336:string)
            n907 = Concatenate Strings(w1343, w1342, w1337, "_stat.csv" ("string")) -> (w1350:string)
            n908 = Concatenate Strings(w1343, w1342, w1337, "_advstat.csv" ("string")) -> (w1340:string)
            n909 = Build Path(base path=w1334, name or relative path=w1336) -> (appended path=w1353:path)
            n910 = Build Path(base path=w1334, name or relative path=w1350) -> (appended path=w1349:path)
            n911 = Build Path(base path=w1334, name or relative path=w1340) -> (appended path=w1339:path)
            n912 = call-poly <vilib>:"Write Delimited Spreadsheet.vi"("file path (dialog if empty)"=w1353, "2D data"=w1335, "delimiter (\\t)"=w1338) -> ()  [unwired: 11 in, 2 out]
            n913 = call-poly <vilib>:"Write Delimited Spreadsheet.vi"("file path (dialog if empty)"=w1349, "2D data"=w1351, "delimiter (\\t)"=w1338) -> ()  [unwired: 11 in, 2 out]
            n914 = call-poly <vilib>:"Write Delimited Spreadsheet.vi"("file path (dialog if empty)"=w1339, "2D data"=w1344, "delimiter (\\t)"=w1338) -> ()  [unwired: 11 in, 2 out]
          }
          frame #13 {
            n915 = local read "total line #"() -> (w1363:i32)
            n916 = local read "Line #"() -> (w1356:i32)
            n917 = local read "scan timing [ms]"() -> (w1357:dbl[][])
            n918 = Equal?(x=w1363, y=w1356) -> (x = y?=w1364:bool)
            n919 = case shown="True" w1364 {
              frame False {
                (unwired) FALSE ("scan mode")
                n920 = local read "Line #"() -> (w1365:i32)
                n921 = Increment(x=w1365) -> (x+1=w1366:i32)
                n922 = local write "Line #"(w1366) -> ()
              }
              frame True {
                w1369 = FALSE ("Boolean")
                n923 = local read "Shutter Port"() -> (w1371:refnum<visa-resource-name>)
                n924 = local write "scan mode"(FALSE ("scan mode")) -> ()
                n925 = local read "Servo Channel"() -> (w1370:u8)
                n926 = control-ref of="Open Shutter"() -> (w1367:refnum<vi>)
                n927 = call "LINX_servo.vi"("Servo Channel"=w1370, "Serial Port"=w1371, "Boolean"=w1369) -> ("Shatter Open"=w1368:bool)  [unwired: 8 in]
                n928 = property on="Property Node" class="Bool (strict)"(reference=w1367, "Value"=w1369) -> ()  [unwired: 1 in, 2 out]
                n929 = local write "Shutter Open"(w1368) -> ()
              }
            }
            n930 = Build Array(w1362, w1361, w1360, w1359) -> (w1358:u32[])
            n931 = Insert Into Array(array=w1357, index (row)=w1356, new element=w1358) -> (w1355:dbl[][])  [unwired: 1 in]
            n932 = local write "scan timing [ms]"(w1355) -> ()
          }
          frame #14 {
            n933 = local read "total line #"() -> (w1374:i32)
            n934 = local read "Line #"() -> (w1375:i32)
            n935 = Equal?(x=w1374, y=w1375) -> (x = y?=w1376:bool)
            n936 = case shown="True" w1376 {
              tunnel: w1373 -> [w1381 _]
              frame True {
                w1377 = ";" ("delimiter (\\t)")
                n937 = Get Date/Time In Seconds() -> (seconds since 1Jan1904=w1397:timestamp)
                n938 = Format Date/Time String(time format string (%c)="%04Y_%02m_%02d_%02H_%02M", seconds (now)=w1397, UTC format=FALSE ("want seconds? (F)")) -> (date/time string=w1383:string)
                n939 = Concatenate Strings("Z_corrdinates_Scan_" ("string"), w1383, ".csv" ("string")) -> (w1393:string)
                n940 = Concatenate Strings("X_corrdinates_Scan_" ("string"), w1383, ".csv" ("string")) -> (w1390:string)
                n941 = Concatenate Strings("Y_corrdinates_Scan_" ("string"), w1383, ".csv" ("string")) -> (w1384:string)
                n942 = Build Path(base path=w1381, name or relative path=w1393) -> (appended path=w1392:path)
                n943 = Build Path(base path=w1381, name or relative path=w1390) -> (appended path=w1387:path)
                n944 = Build Path(base path=w1381, name or relative path=w1384) -> (appended path=w1380:path)
                n945 = local read "Z-coordinates_map"() -> (w1391:dbl[][])
                n946 = local read "X-coordinates_map"() -> (w1386:dbl[][])
                n947 = local read "Y-coordinates_map"() -> (w1379:dbl[][])
                n948 = call-poly <vilib>:"Write Delimited Spreadsheet.vi"("file path (dialog if empty)"=w1392, "2D data"=w1391, "delimiter (\\t)"=w1377) -> ()  [unwired: 11 in, 2 out]
                n949 = call-poly <vilib>:"Write Delimited Spreadsheet.vi"("file path (dialog if empty)"=w1387, "2D data"=w1386, "delimiter (\\t)"=w1377) -> ()  [unwired: 11 in, 2 out]
                n950 = call-poly <vilib>:"Write Delimited Spreadsheet.vi"("file path (dialog if empty)"=w1380, "2D data"=w1379, "delimiter (\\t)"=w1377) -> ()  [unwired: 11 in, 2 out]
              }
              frame False {
              }
            }
          }
          frame #15 {
          }
        }
      }
      frame "Close" {
        n951 = local read "ZaberError"() -> (w1405:errorcluster)
        n952 = local read "Port"() -> (w1404:refnum<visa-resource-name>)
        n953 = local read "Library Initialized"() -> (w1398:bool)
        n954 = call "Close.vi"("error in (no error)"=w1405, "VISA resource name"=w1404) -> ("error out"=→"ZaberError":errorcluster)  [unwired: 9 in]
        n955 = local read "Shutter Open"() -> (w1400:bool)
        n956 = case shown="True" w1398 {
          frame False {
          }
          frame True {
            n957 = call "DANTE close.vi"() -> ("error out"=w1406:errorcluster, "identifier out"=w1407:string)  [unwired: 9 in, 1 out]
            n958 = local write "identifier out"(w1407) -> ()
            n959 = case shown="No Error" w1406 {
              frame No Error {
                w1408 = FALSE ("DANTE loaded")
                n960 = local write "DANTE loaded"(w1408) -> ()
                n961 = local write "Library Initialized"(w1408) -> ()
                n962 = local write "IP added"(w1408) -> ()
                n963 = local write "DANTE configured"(w1408) -> ()
              }
              frame Error {
              }
            }
          }
        }
        n964 = case shown="True" w1400 {
          frame False {
          }
          frame True {
            w1411 = FALSE ("Boolean")
            n965 = local read "Shutter Port"() -> (w1413:refnum<visa-resource-name>)
            n966 = local read "Servo Channel"() -> (w1412:u8)
            n967 = control-ref of="Open Shutter"() -> (w1409:refnum<vi>)
            n968 = call "LINX_servo.vi"("Servo Channel"=w1412, "Serial Port"=w1413, "Boolean"=w1411) -> ("Shatter Open"=w1410:bool)  [unwired: 8 in]
            n969 = local write "Shutter Open"(w1410) -> ()
            n970 = property on="Property Node" class="Bool (strict)"(reference=w1409, "Value"=w1411) -> ()  [unwired: 1 in, 2 out]
          }
        }
        n971 = local write "Program Closed"(TRUE ("Program Close")) -> ()
      }
    }
    n972 = Divide(x=w46, y=u32 1000) -> (x/y=w47:dbl)
    n973 = Reciprocal(x=w47) -> (1/x=→"Loop Speed [1/s]":dbl)
    n974 = Wait Until Next ms Multiple(millisecond multiple=u32 1) -> ()  [unwired: 1 out]
    "Enum" <- w36
  }
  n975 = while {
    stop <- w1414 stop-if-true
    n976 = local read "Connect/Disconnect Prox"() -> (w1417:bool)
    n977 = Equal?(x=w1417, y=TRUE) -> (x = y?=w1415:bool)
    n978 = case shown="True" w1415 {
      frame False {
        (unwired) FALSE
      }
      frame True {
        n979 = stacked-sequence {
          seq-local: [w1421 _ _] -> [_ w1465 _]
          seq-local: [w1423 _ _] -> [_ w1467 _]
          seq-local: [w1422 _ _] -> [_ w1466 _]
          seq-local: [w1420 _ _] -> [_ w1461 _]
          seq-local: [w1419 _ _] -> [_ w1459 _]
          seq-local: [_ w1464 _] -> [_ _ w1491]
          seq-local: [_ w1463 _] -> [_ _ w1490]
          seq-local: [_ w1462 _] -> [_ _ w1489]
          seq-local: [_ w1460 _] -> [_ _ w1488]
          tunnel: [_ _ w1488] -> _
          frame #0 {
            # "Try to open\ncommunication\ninterface"
            # "Inform MEDAQLib\nabout sensor type"
            # "Get Path of MEDAQLib.dll\nAssume it above LabView VI's"
            n980 = Current VI's Path() -> (path=w1438:path)
            n981 = call "GetDLLPath.vi"("VI-Path"=w1438) -> ("DLL-Path"=w1439:path)  [unwired: 10 out]
            n982 = call "CreateSensorInstByName.vi"("DLL-Path"=w1439, "sensor"="Sensor type 2") -> ("Fehler (Ausgang)"=w1436:errorcluster, "instanceHandle"=w1434:u32, "DLL-Path"=w1429:path)  [unwired: 1 in, 10 out]
            n983 = call "SetParameterString.vi"("Fehler (Eingang, kein Fehler)"=w1436, "instanceHandle"=w1434, "DLL-Path"=w1429, "paramName"="IP_Interface", "paramValue"="RS232") -> ("Fehler (Ausgang)"=w1437:errorcluster, "instanceHandle"=w1433:u32, "DLL-Path"=w1430:path)  [unwired: 7 in, 1 out]
            n984 = call "SetParameterString.vi"("Fehler (Eingang, kein Fehler)"=w1437, "instanceHandle"=w1433, "DLL-Path"=w1430, "paramName"="IP_Port", "paramValue"="COM Port 2") -> ("Fehler (Ausgang)"=w1435:errorcluster, "instanceHandle"=w1432:u32, "DLL-Path"=w1431:path)  [unwired: 7 in, 1 out]
            n985 = call "SetParameterInt.vi"("Fehler (Eingang, kein Fehler)"=w1435, "instanceHandle"=w1432, "DLL-Path"=w1431, "paramName"="Baud rate", "paramValue"=921600) -> ("Fehler (Ausgang)"=w1440:errorcluster, "instanceHandle"=w1441:u32, "DLL-Path"=w1442:path)  [unwired: 7 in, 1 out]
            n986 = for {
              N: 1 -> [_]
              tunnel: "COM Port 2" -> [w1456]
              tunnel: [w1446] -> w1420
              tunnel: [w1445] -> w1419
              shift-right: [w1447] -> w1421
              shift-left: w1442 -> [w1455]
              shift-right: [w1448] -> w1422
              shift-left: w1441 -> [w1454]
              shift-right: [w1449] -> w1423
              shift-left: w1440 -> [w1453]
              n987 = call "OpenSensorRS232.vi"("Fehler (Eingang, kein Fehler)"=w1453, "instanceHandle"=w1454, "DLL-Path"=w1455, "port"=w1456) -> ("Fehler (Ausgang)"=w1452:errorcluster, "instanceHandle"=w1451:u32, "DLL-Path"=w1450:path, "ERR_CODE"=w1445:i32)  [unwired: 8 in]
              n988 = call "ErrorHandler.vi"("Fehler (Eingang, kein Fehler)"=w1452, "instanceHandle"=w1451, "DLL-Path"=w1450, "ERR_CODE"=w1445) -> ("Fehler (Ausgang)"=w1449:errorcluster, "instanceHandle"=w1448:u32, "DLL-Path"=w1447:path, "errText"=w1446:string)  [unwired: 8 out]
            }
          }
          frame #1 {
            n989 = Equal?(x=w1459, y=0) -> (x = y?=w1457:bool)
            n990 = while {
              shift-right: [w1487] -> w1464
              shift-left: w1467 -> [w1479]
              shift-right: [w1486] -> w1463
              shift-left: w1466 -> [w1478]
              shift-right: [w1485] -> w1462
              shift-left: w1465 -> [w1477]
              tunnel: [w1469] -> w1460
              stop <- w1469 stop-if-true
              n991 = local read "Connect/Disconnect Prox"() -> (w1472:bool)
              n992 = call "Poll.vi"("Fehler (Eingang, kein Fehler)"=w1479, "instanceHandle"=w1478, "DLL-Path"=w1477, "maxValues"=1) -> ("Fehler (Ausgang)"=w1483:errorcluster, "instanceHandle"=w1482:u32, "DLL-Path"=w1481:path, "ERR_CODE"=w1480:i32, "scaledData"=w1473:dbl[])  [unwired: 6 in, 1 out]
              "?" <- w1473
              n993 = Wait (ms)(milliseconds to wait=u32 25) -> ()  [unwired: 1 out]
              n994 = call "ErrorHandler.vi"("Fehler (Eingang, kein Fehler)"=w1483, "instanceHandle"=w1482, "DLL-Path"=w1481, "ERR_CODE"=w1480) -> ("Fehler (Ausgang)"=w1487:errorcluster, "instanceHandle"=w1486:u32, "DLL-Path"=w1485:path, "errText"=w1475:string)  [unwired: 8 out]
              n995 = Array To Cluster(array=w1473) -> (cluster=w1474:T24)
              n996 = local write "Error!"(w1475) -> ()
              n997 = Equal?(x=w1472, y=FALSE) -> (x = y?=w1469:bool)
              n998 = Not(x=w1469) -> (.not. x?=w1470:bool)
              n999 = local write "Proximity on"(w1470) -> ()
              n1000 = Unbundle(w1474) -> ("scaledData[0]"=→"Proximity distance":dbl)  [unwired: 8 out]
            }
            n1001 = local write "Proximity on"(w1457) -> ()
            "Error!" <- w1461
          }
          frame #2 {
            # "Close communication interface\nRelease MEDAQLib's internal structures"
            n1002 = call "ReleaseSensorInstance.vi"("Fehler (Eingang, kein Fehler)"=w1491, "instanceHandle"=w1490, "DLL-Path"=w1489) -> ("Fehler (Ausgang)"=w1492:errorcluster, "instanceHandle"=w1493:u32, "DLL-Path"=w1494:path)  [unwired: 10 out]
            n1003 = call "CloseSensor.vi"("Fehler (Eingang, kein Fehler)"=w1492, "instanceHandle"=w1493, "DLL-Path"=w1494) -> ()  [unwired: 13 out]
          }
        }
      }
    }
    n1004 = local read "Program Closed"() -> (w1414:bool)
  }
  n1005 = while {
    stop <- w1496 stop-if-true
    n1006 = local read "Proximity distance"() -> (w1497:dbl)
    n1007 = Greater?(x=w1497, y=0.0) -> (0:w1498:bool)
    n1008 = case shown="True" w1498 {
      selector: w1498 -> [_ w1506]
      tunnel: w1497 -> [_ w1505]
      frame False {
      }
      frame True {
        n1009 = case shown="\"lower\"" "limit" {
          tunnel: w1506 -> [w1510 w1630 _]
          tunnel: w1505 -> [w1507 w1627 _]
          frame "lower/upper" {
            n1010 = local read "Prox. distance lower limit"() -> (w1508:dbl)
            n1011 = local read "Prox. distance upper limit"() -> (w1512:dbl)
            n1012 = Less Or Equal?(x=w1507, y=w1508) -> (x <= y?=w1514:bool)
            n1013 = Greater Or Equal?(x=w1507, y=w1512) -> (x >= y?=w1511:bool)
            n1014 = And(x=w1514, y=w1510) -> (x .and. y?=w1513:bool)
            n1015 = And(x=w1511, y=w1510) -> (x .and. y?=w1509:bool)
            n1016 = case shown="True" w1513 {
              tunnel: w1507 -> [w1571 _]
              tunnel: w1508 -> [w1570 _]
              frame False {
                n1017 = Subtract(x=w1571, y=w1570) -> (x-y=w1574:dbl)
                n1018 = Less Or Equal?(x=w1574, y=10.0) -> (x <= y?=w1572:bool)
                n1019 = case shown="False" w1572 {
                  frame False {
                  }
                  frame True {
                    n1020 = local write "Speed Z [mm/s]"(1.0 ("Speed Z [mm/s]")) -> ()
                  }
                }
              }
              frame True {
                n1021 = stacked-sequence {
                  seq-local: [w1579 _ _] -> [_ w1584 _]
                  seq-local: [_ w1583 _] -> [_ _ w1622]
                  frame #0 {
                    (unwired) 0
                    n1022 = local read "Assignment"() -> (w1582:cluster{"Microstep Size":dbl, "Device":string}[])
                    n1023 = local read "Port"() -> (w1578:refnum<visa-resource-name>)
                    n1024 = Index Array(array=w1582, index=2) -> (element=w1579:cluster{"Microstep Size":dbl, "Device":string})
                    n1025 = local read "ZaberError"() -> (w1577:errorcluster)
                    n1026 = Unbundle(w1579) -> ("Device"=w1580:string)  [unwired: 1 out]
                    n1027 = call "Stop.vi"("error in (no error)"=w1577, "Device and Axis"=w1580, "VISA resource name"=w1578) -> ("error out"=w1576:errorcluster)  [unwired: 7 in, 1 out]
                    n1028 = local write "ZaberError"(w1576) -> ()
                  }
                  frame #1 {
                    n1029 = while {
                      tunnel: w1584 -> [w1586]
                      tunnel: [w1585] -> w1583
                      stop <- w1590 stop-if-true
                      w1599 = u16 2 items=["microsteps", "microns", "millimeters", "inches"] ("Units (0: microsteps)")
                      w1611 = u16 2 items=["device units", "microns/s^2", "mm/s^2", "inches/s^2", "degrees/s^2"] ("Units (0: data)")
                      w1606 = u16 2 items=["device speed units", "microns per second", "millimeters per second", "inches per second", "degrees per second"] ("Units (0: device speed units)")
                      # "move at specified velocity command"
                      n1030 = local read "Acceleration\n [mm/s^2]"() -> (w1610:dbl)
                      n1031 = local read "Port"() -> (w1591:refnum<visa-resource-name>)
                      n1032 = local read "ZaberError"() -> (w1609:errorcluster)
                      n1033 = Negate(x=2.0) -> (-x=w1605:dbl)
                      n1034 = Wait (ms)(milliseconds to wait=u32 10) -> ()  [unwired: 1 out]
                      n1035 = Unbundle(w1586) -> ("Microstep Size"=w1608:dbl, "Device"=w1607:string)
                      n1036 = call "Set Acceleration.vi"("Units (0: data)"=w1611, "New Acceleration"=w1610, "error in (no error)"=w1609, "Device and Axis"=w1607, "Microstep Size (0)"=w1608, "VISA resource name"=w1591) -> ("error out"=w1603:errorcluster, "VISA resource name out"=w1604:refnum<visa-resource-name>)  [unwired: 4 in]
                      n1037 = call "Move at Velocity.vi"("Units (0: device speed units)"=w1606, "Velocity"=w1605, "error in (no error)"=w1603, "Device and Axis"=w1607, "Microstep Size (0)"=w1608, "VISA resource name"=w1604) -> ("error out"=w1602:errorcluster, "VISA resource name out"=w1601:refnum<visa-resource-name>)  [unwired: 4 in]
                      n1038 = Unbundle(w1586) -> ("Microstep Size"=w1597:dbl, "Device"=w1587:string)
                      n1039 = local read "Prox. distance lower limit"() -> (w1595:dbl)
                      n1040 = local read "Proximity distance"() -> (w1594:dbl)
                      n1041 = call "Read Current Position.vi"("Units (0: microsteps)"=w1599, "error in (no error)"=w1602, "Device and Axis"=w1587, "Microstep Size (0)"=w1597, "VISA resource name"=w1601) -> ("error out"=w1612:errorcluster, "Position"=w1598:dbl)  [unwired: 4 in, 1 out]
                      n1042 = local read "Program Closed"() -> (w1596:bool)
                      n1043 = local write "ZaberError"(w1612) -> ()
                      n1044 = local write "Z [mm]"(w1598) -> ()
                      n1045 = Greater?(x=w1594, y=w1595) -> (0:w1589:bool)
                      n1046 = Less Than 0?(x=w1594) -> (x < 0?=w1593:bool)
                      n1047 = case shown="True" w1589 {
                        tunnel: w1586 -> [w1613 w1616]
                        tunnel: [w1613 w1614] -> w1585
                        frame False {
                        }
                        frame True {
                          n1048 = for {
                            N: 0 -> [_]
                            shift-right: [w1617] -> w1614
                            shift-left: w1616 -> [w1617]
                            # "stop command"
                            n1049 = Unbundle(w1617) -> ("Device"=w1618:string)  [unwired: 1 out]
                            n1050 = local read "Port"() -> (w1619:refnum<visa-resource-name>)
                            n1051 = local read "ZaberError"() -> (w1620:errorcluster)
                            n1052 = call "Stop.vi"("error in (no error)"=w1620, "Device and Axis"=w1618, "VISA resource name"=w1619) -> ("error out"=w1621:errorcluster)  [unwired: 7 in, 1 out]
                            n1053 = local write "ZaberError"(w1621) -> ()
                          }
                        }
                      }
                      n1054 = Or(x=w1589, y=w1596) -> (x .or. y?=w1592:bool)
                      n1055 = Or(x=w1593, y=w1592) -> (x .or. y?=w1590:bool)
                    }
                  }
                  frame #2 {
                    # "stop command"
                    n1056 = Unbundle(w1622) -> ("Device"=w1623:string)  [unwired: 1 out]
                    n1057 = local read "Port"() -> (w1624:refnum<visa-resource-name>)
                    n1058 = local read "ZaberError"() -> (w1625:errorcluster)
                    n1059 = call "Stop.vi"("error in (no error)"=w1625, "Device and Axis"=w1623, "VISA resource name"=w1624) -> ("error out"=w1626:errorcluster)  [unwired: 7 in, 1 out]
                    n1060 = local write "ZaberError"(w1626) -> ()
                  }
                }
              }
            }
            n1061 = case shown="True" w1509 {
              frame False {
              }
              frame True {
                n1062 = stacked-sequence {
                  seq-local: [w1518 _ _] -> [_ w1523 _]
                  seq-local: [_ w1522 _] -> [_ _ w1565]
                  frame #0 {
                    (unwired) 0
                    n1063 = local read "Assignment"() -> (w1521:cluster{"Microstep Size":dbl, "Device":string}[])
                    n1064 = local read "Port"() -> (w1517:refnum<visa-resource-name>)
                    n1065 = Index Array(array=w1521, index=2) -> (element=w1518:cluster{"Microstep Size":dbl, "Device":string})
                    n1066 = local read "ZaberError"() -> (w1516:errorcluster)
                    n1067 = Unbundle(w1518) -> ("Device"=w1519:string)  [unwired: 1 out]
                    n1068 = call "Stop.vi"("error in (no error)"=w1516, "Device and Axis"=w1519, "VISA resource name"=w1517) -> ("error out"=w1515:errorcluster)  [unwired: 7 in, 1 out]
                    n1069 = local write "ZaberError"(w1515) -> ()
                  }
                  frame #1 {
                    n1070 = while {
                      tunnel: w1523 -> [w1535]
                      tunnel: [w1534] -> w1522
                      stop <- w1524 stop-if-true
                      w1543 = u16 2 items=["microsteps", "microns", "millimeters", "inches"] ("Units (0: microsteps)")
                      w1554 = u16 2 items=["device units", "microns/s^2", "mm/s^2", "inches/s^2", "degrees/s^2"] ("Units (0: data)")
                      w1549 = u16 2 items=["device speed units", "microns per second", "millimeters per second", "inches per second", "degrees per second"] ("Units (0: device speed units)")
                      # "move at specified velocity command"
                      n1071 = local read "Acceleration\n [mm/s^2]"() -> (w1553:dbl)
                      n1072 = local read "Port"() -> (w1537:refnum<visa-resource-name>)
                      n1073 = local read "ZaberError"() -> (w1552:errorcluster)
                      n1074 = Wait (ms)(milliseconds to wait=u32 10) -> ()  [unwired: 1 out]
                      n1075 = Unbundle(w1535) -> ("Microstep Size"=w1551:dbl, "Device"=w1550:string)
                      n1076 = call "Set Acceleration.vi"("Units (0: data)"=w1554, "New Acceleration"=w1553, "error in (no error)"=w1552, "Device and Axis"=w1550, "Microstep Size (0)"=w1551, "VISA resource name"=w1537) -> ("error out"=w1547:errorcluster, "VISA resource name out"=w1548:refnum<visa-resource-name>)  [unwired: 4 in]
                      n1077 = call "Move at Velocity.vi"("Units (0: device speed units)"=w1549, "Velocity"=2.0 ("x"), "error in (no error)"=w1547, "Device and Axis"=w1550, "Microstep Size (0)"=w1551, "VISA resource name"=w1548) -> ("error out"=w1546:errorcluster, "VISA resource name out"=w1545:refnum<visa-resource-name>)  [unwired: 4 in]
                      n1078 = local read "Prox. distance upper limit"() -> (w1532:dbl)
                      n1079 = Unbundle(w1535) -> ("Microstep Size"=w1541:dbl, "Device"=w1536:string)
                      n1080 = local read "Proximity distance"() -> (w1531:dbl)
                      n1081 = call "Read Current Position.vi"("Units (0: microsteps)"=w1543, "error in (no error)"=w1546, "Device and Axis"=w1536, "Microstep Size (0)"=w1541, "VISA resource name"=w1545) -> ("error out"=w1555:errorcluster, "Position"=w1542:dbl)  [unwired: 4 in, 1 out]
                      n1082 = local read "limit"() -> (w1530:T4)
                      n1083 = local write "ZaberError"(w1555) -> ()
                      n1084 = Equal?(x=w1530, y=T4."off Selection 4") -> (x = y?=w1528:bool)
                      n1085 = local write "Z [mm]"(w1542) -> ()
                      n1086 = Less?(x=w1531, y=w1532) -> (x < y?=w1527:bool)
                      n1087 = Or(x=w1527, y=w1528) -> (x .or. y?=w1525:bool)
                      n1088 = Less Than 0?(x=w1531) -> (x < 0?=w1539:bool)
                      n1089 = local read "Program Closed"() -> (w1540:bool)
                      n1090 = case shown="True" w1525 {
                        tunnel: w1535 -> [w1556 w1559]
                        tunnel: [w1556 w1557] -> w1534
                        frame False {
                        }
                        frame True {
                          n1091 = for {
                            N: 0 -> [_]
                            shift-right: [w1560] -> w1557
                            shift-left: w1559 -> [w1560]
                            # "stop command"
                            n1092 = Unbundle(w1560) -> ("Device"=w1561:string)  [unwired: 1 out]
                            n1093 = local read "Port"() -> (w1562:refnum<visa-resource-name>)
                            n1094 = local read "ZaberError"() -> (w1563:errorcluster)
                            n1095 = call "Stop.vi"("error in (no error)"=w1563, "Device and Axis"=w1561, "VISA resource name"=w1562) -> ("error out"=w1564:errorcluster)  [unwired: 7 in, 1 out]
                            n1096 = local write "ZaberError"(w1564) -> ()
                          }
                        }
                      }
                      n1097 = Or(x=w1527, y=w1540) -> (x .or. y?=w1538:bool)
                      n1098 = Or(x=w1539, y=w1538) -> (x .or. y?=w1526:bool)
                      n1099 = Or(x=w1526, y=w1525) -> (x .or. y?=w1524:bool)
                    }
                  }
                  frame #2 {
                    # "stop command"
                    n1100 = Unbundle(w1565) -> ("Device"=w1566:string)  [unwired: 1 out]
                    n1101 = local read "Port"() -> (w1567:refnum<visa-resource-name>)
                    n1102 = local read "ZaberError"() -> (w1568:errorcluster)
                    n1103 = call "Stop.vi"("error in (no error)"=w1568, "Device and Axis"=w1566, "VISA resource name"=w1567) -> ("error out"=w1569:errorcluster)  [unwired: 7 in, 1 out]
                    n1104 = local write "ZaberError"(w1569) -> ()
                  }
                }
              }
            }
          }
          frame "lower" {
            n1105 = local read "Prox. distance lower limit"() -> (w1628:dbl)
            n1106 = Less Or Equal?(x=w1627, y=w1628) -> (x <= y?=w1629:bool)
            n1107 = And(x=w1629, y=w1630) -> ()  [unwired: 1 out]
            n1108 = case shown="True" w1629 {
              tunnel: w1627 -> [w1632 _]
              tunnel: w1628 -> [w1631 _]
              frame False {
                n1109 = Subtract(x=w1632, y=w1631) -> (x-y=w1635:dbl)
                n1110 = Less Or Equal?(x=w1635, y=10.0) -> (x <= y?=w1633:bool)
                n1111 = case shown="True" w1633 {
                  frame False {
                  }
                  frame True {
                    n1112 = local write "Speed Z [mm/s]"(1.0 ("Speed Z [mm/s]")) -> ()
                  }
                }
              }
              frame True {
                n1113 = stacked-sequence {
                  seq-local: [w1640 _ _] -> [_ w1645 _]
                  seq-local: [_ w1644 _] -> [_ _ w1684]
                  frame #0 {
                    n1114 = local read "Assignment"() -> (w1643:cluster{"Microstep Size":dbl, "Device":string}[])
                    n1115 = local read "Port"() -> (w1639:refnum<visa-resource-name>)
                    n1116 = Index Array(array=w1643, index=2) -> (element=w1640:cluster{"Microstep Size":dbl, "Device":string})
                    n1117 = local read "ZaberError"() -> (w1638:errorcluster)
                    n1118 = Unbundle(w1640) -> ("Device"=w1641:string)  [unwired: 1 out]
                    n1119 = call "Stop.vi"("error in (no error)"=w1638, "Device and Axis"=w1641, "VISA resource name"=w1639) -> ("error out"=w1637:errorcluster)  [unwired: 7 in, 1 out]
                    n1120 = local write "ZaberError"(w1637) -> ()
                  }
                  frame #1 {
                    n1121 = while {
                      tunnel: w1645 -> [w1647]
                      tunnel: [w1646] -> w1644
                      stop <- w1651 stop-if-true
                      w1660 = u16 2 items=["microsteps", "microns", "millimeters", "inches"] ("Units (0: microsteps)")
                      w1672 = u16 2 items=["device units", "microns/s^2", "mm/s^2", "inches/s^2", "degrees/s^2"] ("Units (0: data)")
                      w1667 = u16 2 items=["device speed units", "microns per second", "millimeters per second", "inches per second", "degrees per second"] ("Units (0: device speed units)")
                      # "move at specified velocity command"
                      n1122 = local read "Acceleration\n [mm/s^2]"() -> (w1671:dbl)
                      n1123 = local read "Port"() -> (w1652:refnum<visa-resource-name>)
                      n1124 = local read "ZaberError"() -> (w1670:errorcluster)
                      n1125 = Negate(x=1.0) -> (-x=w1666:dbl)
                      n1126 = Wait (ms)(milliseconds to wait=u32 10) -> ()  [unwired: 1 out]
                      n1127 = Unbundle(w1647) -> ("Microstep Size"=w1669:dbl, "Device"=w1668:string)
                      n1128 = call "Set Acceleration.vi"("Units (0: data)"=w1672, "New Acceleration"=w1671, "error in (no error)"=w1670, "Device and Axis"=w1668, "Microstep Size (0)"=w1669, "VISA resource name"=w1652) -> ("error out"=w1664:errorcluster, "VISA resource name out"=w1665:refnum<visa-resource-name>)  [unwired: 4 in]
                      n1129 = call "Move at Velocity.vi"("Units (0: device speed units)"=w1667, "Velocity"=w1666, "error in (no error)"=w1664, "Device and Axis"=w1668, "Microstep Size (0)"=w1669, "VISA resource name"=w1665) -> ("error out"=w1663:errorcluster, "VISA resource name out"=w1662:refnum<visa-resource-name>)  [unwired: 4 in]
                      n1130 = Unbundle(w1647) -> ("Microstep Size"=w1658:dbl, "Device"=w1648:string)
                      n1131 = local read "Prox. distance lower limit"() -> (w1656:dbl)
                      n1132 = local read "Proximity distance"() -> (w1655:dbl)
                      n1133 = call "Read Current Position.vi"("Units (0: microsteps)"=w1660, "error in (no error)"=w1663, "Device and Axis"=w1648, "Microstep Size (0)"=w1658, "VISA resource name"=w1662) -> ("error out"=w1673:errorcluster, "Position"=w1659:dbl)  [unwired: 4 in, 1 out]
                      n1134 = local read "Program Closed"() -> (w1657:bool)
                      n1135 = local write "ZaberError"(w1673) -> ()
                      n1136 = local write "Z [mm]"(w1659) -> ()
                      n1137 = Greater?(x=w1655, y=w1656) -> (0:w1650:bool)
                      n1138 = Less Than 0?(x=w1655) -> (x < 0?=w1654:bool)
                      n1139 = case shown="True" w1650 {
                        tunnel: w1647 -> [w1674 w1677]
                        tunnel: [w1674 w1675] -> w1646
                        frame False {
                        }
                        frame True {
                          n1140 = for {
                            N: 0 -> [_]
                            shift-right: [w1678] -> w1675
                            shift-left: w1677 -> [w1678]
                            # "stop command"
                            n1141 = Unbundle(w1678) -> ("Device"=w1679:string)  [unwired: 1 out]
                            n1142 = local read "Port"() -> (w1680:refnum<visa-resource-name>)
                            n1143 = local read "ZaberError"() -> (w1681:errorcluster)
                            n1144 = call "Stop.vi"("error in (no error)"=w1681, "Device and Axis"=w1679, "VISA resource name"=w1680) -> ("error out"=w1682:errorcluster)  [unwired: 7 in, 1 out]
                            n1145 = local write "ZaberError"(w1682) -> ()
                          }
                        }
                      }
                      n1146 = Or(x=w1650, y=w1657) -> (x .or. y?=w1653:bool)
                      n1147 = Or(x=w1654, y=w1653) -> (x .or. y?=w1651:bool)
                    }
                  }
                  frame #2 {
                    n1148 = for {
                      N: 0 -> [_]
                      tunnel: w1684 -> [w1689]
                      # "stop command"
                      n1149 = Unbundle(w1689) -> ("Device"=w1685:string)  [unwired: 1 out]
                      n1150 = local read "Port"() -> (w1686:refnum<visa-resource-name>)
                      n1151 = local read "ZaberError"() -> (w1687:errorcluster)
                      n1152 = call "Stop.vi"("error in (no error)"=w1687, "Device and Axis"=w1685, "VISA resource name"=w1686) -> ("error out"=w1688:errorcluster)  [unwired: 7 in, 1 out]
                      n1153 = local write "ZaberError"(w1688) -> ()
                    }
                  }
                }
              }
            }
          }
          frame "off Selection 4", Default {
          }
        }
      }
    }
    n1154 = local read "limit"() -> (w1495:T4)
    n1155 = case shown="\"off Selection 4\"" w1495 {
      frame "lower", Default {
        n1156 = property on="Prox. distance upper limit" class="DigNum (strict)"("DisabledEnum"=T15."Disabled and Grayed Out" ("Disabled")) -> ()  [unwired: 2 in, 2 out]
        n1157 = property on="Prox. distance lower limit" class="DigNum (strict)"("DisabledEnum"=T15."Enabled" ("Disabled")) -> ()  [unwired: 2 in, 2 out]
      }
      frame "lower/upper" {
        w1502 = T15."Enabled" ("Disabled")
        n1158 = property on="Prox. distance upper limit" class="DigNum (strict)"("DisabledEnum"=w1502) -> ()  [unwired: 2 in, 2 out]
        n1159 = property on="Prox. distance lower limit" class="DigNum (strict)"("DisabledEnum"=w1502) -> ()  [unwired: 2 in, 2 out]
      }
      frame "off Selection 4" {
        w1503 = T15."Disabled and Grayed Out" ("Disabled")
        n1160 = property on="Prox. distance upper limit" class="DigNum (strict)"("DisabledEnum"=w1503) -> ()  [unwired: 2 in, 2 out]
        n1161 = property on="Prox. distance lower limit" class="DigNum (strict)"("DisabledEnum"=w1503) -> ()  [unwired: 2 in, 2 out]
      }
    }
    n1162 = local read "Program Closed"() -> (w1496:bool)
  }
  n1163 = disable-structure shown="Disabled" {
    frame Disabled {
      (unwired) 0.0 ("y")
      n1164 = Greater Or Equal?() -> (x=w1690:dbl)  [unwired: 1 in, 1 out]
      n1165 = case shown="True" {
        selector: _ -> [_ _]
        tunnel: _ -> [_ w1694]
        frame False {
          w1691 = T15."Enabled" ("Disabled")
        }
        frame True {
          n1166 = local read "Prox. distance lower limit"() -> (w1692:dbl)
          n1167 = Greater Or Equal?(x=w1694, y=w1692) -> (x >= y?=w1693:bool)
          n1168 = case shown="False" w1693 {
            frame False {
              (unwired) T15."Disabled and Grayed Out" ("Disabled")
            }
            frame True {
              w1695 = T15."Enabled" ("Disabled")
            }
          }
        }
      }
    }
    frame Enabled {
    }
  }
  n1169 = while {
    stop <- w1697 stop-if-true
    n1170 = case shown="True" "Connect/Disconnect Camera" {
      frame False {
      }
      frame True {
        n1171 = call "Camera.vi"("Refnum in"="Session In") -> ()  [unwired: 10 in, 1 out]
      }
    }
    n1172 = local read "Program Closed"() -> (w1697:bool)
  }
  n1173 = disable-structure shown="Disabled" {
    frame Disabled {
      n1174 = property on="Property Node" class="Ctl"(reference="Pause button 2") -> ("Value"=w1702:variant)  [unwired: 1 in, 2 out]
      n1175 = Variant To Data(type=TRUE, Variant=w1702) -> (data=w1699:bool)  [unwired: 1 in, 1 out]
      n1176 = case shown="True" w1699 {
        frame False {
        }
        frame True {
          n1177 = while {
            stop <- w1703 continue-if-true
            n1178 = local read "Pause button 2"() -> (w1704:refnum<vi>)
            n1179 = Wait (ms)(milliseconds to wait=u32 10) -> ()  [unwired: 1 out]
            n1180 = property on="Property Node" class="Ctl"(reference=w1704) -> ("Value"=w1706:variant)  [unwired: 1 in, 2 out]
            n1181 = Variant To Data(type=TRUE, Variant=w1706) -> (data=w1703:bool)  [unwired: 1 in, 1 out]
          }
        }
      }
    }
    frame Enabled {
    }
  }
  n1182 = disable-structure shown="Disabled" {
    frame Disabled {
      n1183 = local read "Prox. distance lower limit"() -> (w1709:dbl)
      n1184 = local read "Proximity distance"() -> (w1708:dbl)
      n1185 = case shown="True" {
        selector: _ -> [_ _]
        frame False {
        }
        frame True {
          n1186 = property on="Closer" class="Bool (strict)"("DisabledEnum"=T15."Enabled" ("Disabled")) -> ()  [unwired: 2 in, 2 out]
        }
      }
      n1187 = Greater Or Equal?(x=w1708, y=w1709) -> (x >= y?=w1710:bool)
    }
    frame Enabled {
    }
  }
  "Proximity on" <- FALSE ("Proximity on")
  "Program Closed" <- FALSE ("Program Close")
  "Measurement On!" <- FALSE ("Measurement On!")
